vi "H2O_DIAL_NCAR_4CH_v4.09.vi"() -> ()   [LabVIEW 2012]
uses:
  C:/Users/H2ODial/Desktop/Shared Telescope WV DIAL Code/Libraries and VIs/PowerMeterCommands.dll
  Shared Telescope WV DIAL Code/Libraries and VIs/PowerMeterCommands.dll
  <vilib>/DAQmx/write.llb/DAQmx Write (Digital 1D Bool NChan 1Samp 1Line).vi
  <vilib>/DAQmx/miscellaneous.llb/DAQmx Fill In Error Info.vi
  <vilib>/Analysis/baseanly.llb/Mean (DBL).vi
  AMCS_Data.vi
  Libraries and VIs/Scalar_Data.vi
  <vilib>/Analysis/NI_AALBase.lvlib
  Libraries and VIs/Scalar_Data_2.vi
  Libraries and VIs/Scalar_Data_4.vi
  Libraries and VIs/Scalar_Data_3.vi
  Shared Telescope WV DIAL Code/bristol/CLDevIFace.dll
panel:
  out "FileHour":i32=18
  out "L_Count":i32=271
  out "sigma_off_total":dbl[](array[numeric])=[5.540716545669956e-25, 5.509038515319884e-25, 5.47745233176751e-25, 5.445958679910823e-25, 5.414558240969882e-25, 5.383251691981853e-25, 5.352039705244152e-25, 5.320922947769417e-25, 5.289902080890823e-25, 5.258977759647611e-25, 5.228150632368401e-25, 5.197421340189991e-25, 5.166790516619597e-25, 5.1362587870950455e-25, 5.1058267685284e-25, 5.075495068909035e-25, 5.045264286935022e-25, 5.015135011569438e-25, 4.9851078217155e-25, 4.955183285861175e-25, 4.925361961723897e-25, 4.895644395896113e-25, 4.866031123592904e-25, 4.83652266834119e-25, 4.807119541641849e-25, 4.77782224277593e-25, 4.7486312585251305e-25, 4.719547062922376e-25, 4.690570117073194e-25, 4.661700868866856e-25, 4.632939752896641e-25, 4.604287190200865e-25, 4.575743588116101e-25, 4.547309340157799e-25, 4.518984825887645e-25, 4.490770410729631e-25, 4.462666445972589e-25, 4.434673268575131e-25, 4.40679120118145e-25, 4.379020551981193e-25, 4.351361614712452e-25, 4.3238146686004e-25, 4.296379978359628e-25, 4.26905779413425e-25, 4.241848351562388e-25, 4.214751871753208e-25, 4.187768561289679e-25, 4.160898612350621e-25, 4.134142202652132e-25, 4.1074994956030275e-25, 4.0809706402935364e-25, 4.054555771658063e-25, 4.0282550104859823e-25, 4.002068463591525e-25, 3.9759962238789642e-25, 3.9500383704632943e-25, 3.9241949688533782e-25, 3.89846607100192e-25, 3.8728517155268345e-25, 3.8473519278212167e-25, 3.8219667202352144e-25, 3.7966960922230447e-25, 3.7715400305383413e-25, 3.74649850940483e-25, 3.7215714907036218e-25, 3.6967589241566724e-25, 3.672060747564097e-25, 3.647476886940111e-25, 3.6230072567890353e-25, 3.598651760279724e-25, 3.5744102894632373e-25, 3.550282725512238e-25, 3.5262689389447565e-25, 3.502368789807654e-25, 3.47858212798661e-25, 3.454908793351493e-25, 3.4313486160611974e-25, 3.407901416757848e-25, 3.3845670068390906e-25, 3.36134518864904e-25, 3.3382357557846445e-25, 3.31523849327317e-25, 3.292353177855014e-25, 3.269579578225686e-25, 3.2469174552554615e-25, 3.224366562247346e-25, 3.201926645171508e-25, 3.179597442913807e-25, 3.157378687515629e-25, 3.135270104405692e-25, 3.113271412644526e-25, 3.091382325146825e-25, 3.069602548935796e-25, 3.0479317853615826e-25, 3.026369730325113e-25, 3.004916074531155e-25, 2.9835705036817056e-25, 2.9623326987117465e-25, 2.941202336026831e-25, 2.9201790876899676e-25, 2.899262621653904e-25, 2.8784526019663433e-25, 2.8577486889781736e-25, 2.8371505395538697e-25, 2.8166578072571985e-25, 2.7962701425816637e-25, 2.775987193103717e-25, 2.7558086037064965e-25, 2.735734016758066e-25, 2.71576307229708e-25, 2.6958954082151585e-25, 2.6761306604360893e-25, 2.6564684630829226e-25, 2.6369084486778265e-25, 2.61745024828016e-25, 2.598093491667028e-25, 2.578837807496939e-25, 2.559682823474498e-25, 2.54062816650001e-25, 2.521673462824945e-25, 2.502818338212059e-25, 2.484062418077259e-25, 2.4654053276440287e-25, 2.446846692077008e-25, 2.4283861366280177e-25, 2.410023286792255e-25, 2.391757768411529e-25, 2.3735892078424688e-25, 2.3555172320627342e-25, 2.337541468826103e-25, 2.3196615467596074e-25, 2.3018770955218097e-25, 2.2841877458964754e-25, 2.2665931299334314e-25, 2.2490928810607227e-25, 2.2316866341927193e-25, 2.2143740258515955e-25, 2.197154694282537e-25, 2.1800282795472234e-25, 2.1629944236413983e-25, 2.146052770592492e-25, 2.1292029665592434e-25, 2.112444659932193e-25, 2.0957775014166358e-25, 2.0792011441327743e-25, 2.0627152437013555e-25, 2.0463194583169568e-25, 2.0300134488359706e-25, 2.0137968788457824e-25, 1.9976694147385576e-25, 1.9816307257768824e-25, 1.9656804841491914e-25, 1.9498183650353885e-25, 1.934044046652418e-25, 1.9183572103011107e-25, 1.9027575404100786e-25, 1.8872447245712642e-25, 1.871818453566729e-25, 1.8564784213957954e-25, 1.841224325294735e-25, 1.8260558657484057e-25, 1.810972746495391e-25, 1.7959746745324166e-25, 1.7810613601054828e-25, 1.7662325167008742e-25, 1.751487861025293e-25, 1.7368271129853726e-25, 1.7222499956532122e-25, 1.7077562352346513e-25, 1.6933455610234437e-25, 1.6790177053565633e-25, 1.6647724035593172e-25, 1.6506093938856987e-25, 1.636528417453577e-25, 1.6225292181758646e-25, 1.608611542684316e-25, 1.5947751402502352e-25, 1.581019762699804e-25, 1.5673451643257683e-25, 1.5537511017940605e-25, 1.540237334047793e-25, 1.5268036222071082e-25, 1.5134497294663046e-25, 1.5001754209881617e-25, 1.4869804637954348e-25, 1.473864626661357e-25, 1.460827679996712e-25, 1.4478693957377917e-25, 1.4349895472319421e-25, 1.4221879091216375e-25, 1.4094642572317599e-25, 1.3968183684535146e-25, 1.3842500206296053e-25, 1.3717589924428774e-25, 1.3593450633030128e-25, 1.3470080132367275e-25, 1.3347476227802004e-25, 1.32256367287135e-25, 1.3104559447485225e-25, 1.2984242198512939e-25, 1.2864682797194944e-25, 1.2745879059051496e-25, 1.2627828798814573e-25, 1.2510529829571843e-25, 1.2393979961981194e-25, 1.2278177003500287e-25, 1.2163118757700842e-25, 1.204880302361001e-25, 1.193522759513445e-25, 1.1822390260474241e-25, 1.1710288801689803e-25, 1.1598920994272827e-25, 1.1488284606766496e-25, 1.1378377400487363e-25, 1.1269197129279468e-25, 1.1160741539351538e-25, 1.1053008369155443e-25, 1.094599534933665e-25, 1.0839700202769103e-25, 1.0734120644581644e-25, 1.0629254382333933e-25, 1.0525099116192388e-25, 1.0421652539159365e-25, 1.0318912337377015e-25, 1.0216876190431015e-25, 1.0115541771807728e-25, 1.0014906749271105e-25, 9.914968785310339e-26, 9.815725537656191e-26, 9.717174659823899e-26, 9.619313801588218e-26, 9.522140609573087e-26, 9.425652727838355e-26, 9.329847798391668e-26, 9.234723461772877e-26, 9.140277357589357e-26, 9.046507125086315e-26, 8.953410403602918e-26, 8.860984833089776e-26, 8.769228054525757e-26, 8.678137710332858e-26, 8.587711444744364e-26, 8.497946904095774e-26, 8.408841737046818e-26, 8.320393594822389e-26, 8.232600131299494e-26, 8.145459003094604e-26, 8.058967869545014e-26, 7.973124392609961e-26, 7.887926236794523e-26, 7.80337106887695e-26, 7.719456557686526e-26, 7.636180373727653e-26, 7.553540188807418e-26, 7.47153367556762e-26, 7.390158506951166e-26, 7.309412355721905e-26, 7.22929289380143e-26, 7.149797791632498e-26, 7.070924717536157e-26, 6.992671337018222e-26, 6.915035312057113e-26, 6.838014300354704e-26, 6.761605954618939e-26, 6.685807921858866e-26, 6.61061784263726e-26, 6.536033350360778e-26, 6.462052070600663e-26, 6.388671620424742e-26, 6.315889607734174e-26, 6.243703630693181e-26, 6.172111277147462e-26, 6.101110124059749e-26, 6.030697737083214e-26, 5.960871670108947e-26, 5.891629464803492e-26, 5.822968650369955e-26]
  out "sigma_on_total":dbl[](array[numeric])=[3.7287541155959287e-23, 3.7294473381390915e-23, 3.729895983299971e-23, 3.7300992376506543e-23, 3.730056364270663e-23, 3.729766703617701e-23, 3.729229674071814e-23, 3.728444772415678e-23, 3.7274115748913616e-23, 3.7261297371484216e-23, 3.724598994972533e-23, 3.722819164604523e-23, 3.720790143143009e-23, 3.718511908815845e-23, 3.7159845210402426e-23, 3.71320812064078e-23, 3.710182930085371e-23, 3.7069092532052533e-23, 3.7033874753800484e-23, 3.69961806343696e-23, 3.6956015654087493e-23, 3.691338610146597e-23, 3.686829907341892e-23, 3.682076247098229e-23, 3.677078499195744e-23, 3.6718376130128133e-23, 3.666354616830143e-23, 3.6606306171503594e-23, 3.65466679828621e-23, 3.648464421148751e-23, 3.642024823133154e-23, 3.635349416790373e-23, 3.628439689018491e-23, 3.6212972002870696e-23, 3.613923583641449e-23, 3.6063205432233156e-23, 3.5984898538517206e-23, 3.590433359182844e-23, 3.582152971111225e-23, 3.573650667999674e-23, 3.5649284937303634e-23, 3.5559885561897056e-23, 3.546833026061457e-23, 3.537464135047522e-23, 3.5278841748472396e-23, 3.518095495390081e-23, 3.5081005031164986e-23, 3.49790166003625e-23, 3.4875014813139384e-23, 3.476902534357424e-23, 3.4661074365208697e-23, 3.455118854053173e-23, 3.443939499746446e-23, 3.432572131749493e-23, 3.421019551446019e-23, 3.409284601679323e-23, 3.3973701654248835e-23, 3.385279163246072e-23, 3.3730145521256737e-23, 3.360579323268562e-23, 3.3479765004528353e-23, 3.3352091380022967e-23, 3.322280319128026e-23, 3.3091931539878165e-23, 3.2959507778385764e-23, 3.2825563490963637e-23, 3.269013047870121e-23, 3.255324073466697e-23, 3.2414926432195465e-23, 3.227521990292009e-23, 3.2134153618673575e-23, 3.1991760175402e-23, 3.18480722753372e-23, 3.1703122704608974e-23, 3.155694432423841e-23, 3.1409570043398513e-23, 3.126103280985793e-23, 3.1111365588382064e-23, 3.096060134785198e-23, 3.0808773039207797e-23, 3.065591358683448e-23, 3.050205586515653e-23, 3.0347232687749715e-23, 3.0191476792033654e-23, 3.003482082145855e-23, 2.987729731269763e-23, 2.971893868034824e-23, 2.9559777203834095e-23, 2.939984501370705e-23, 2.923917407736587e-23, 2.907779618698884e-23, 2.891574294504204e-23, 2.875304575478364e-23, 2.8589735806501847e-23, 2.842584406506734e-23, 2.826140126245158e-23, 2.809643788235476e-23, 2.7930984151658057e-23, 2.7765070033138635e-23, 2.759872521128409e-23, 2.743197908578835e-23, 2.726486076178917e-23, 2.7097399041404717e-23, 2.6929622416549404e-23, 2.67615590585557e-23, 2.6593236816217257e-23, 2.6424683201727417e-23, 2.62559253894762e-23, 2.6086990208089785e-23, 2.5917904134629101e-23, 2.5748693289157014e-23, 2.5579383429670766e-23, 2.5409999945669205e-23, 2.524056785899295e-23, 2.507111181376249e-23, 2.4901656075333742e-23, 2.4732224526983488e-23, 2.4562840667772406e-23, 2.4393527608193136e-23, 2.422430806785886e-23, 2.405520437517099e-23, 2.3886238463936548e-23, 2.3717431873629354e-23, 2.3548805745800924e-23, 2.3380380824113516e-23, 2.3212177457869647e-23, 2.304421559359465e-23, 2.287651478317675e-23, 2.2709094177653898e-23, 2.2541972534144295e-23, 2.2375168208619667e-23, 2.2208699165636514e-23, 2.2042582971637662e-23, 2.1876836801909522e-23, 2.1711477440630507e-23, 2.1546521280412932e-23, 2.1381984326685983e-23, 2.121788220142687e-23, 2.1054230141008472e-23, 2.089104300259618e-23, 2.072833526537848e-23, 2.0566121033484556e-23, 2.0404414040514995e-23, 2.02432276490701e-23, 2.0082574857776725e-23, 1.992246830471324e-23, 1.9762920267394525e-23, 1.960394267008934e-23, 1.94455470854802e-23, 1.9287744739998634e-23, 1.913054651781045e-23, 1.897396296213913e-23, 1.8818004283613368e-23, 1.866268036173684e-23, 1.850800074923581e-23, 1.8353974677805328e-23, 1.8200611062528066e-23, 1.8047918504372124e-23, 1.789590529608809e-23, 1.7744579427440173e-23, 1.7593948589158073e-23, 1.7444020176312072e-23, 1.7294801295571033e-23, 1.714629876734015e-23, 1.6998519132395303e-23, 1.6851468654733394e-23, 1.6705153329424692e-23, 1.6559578883024505e-23, 1.6414750782637343e-23, 1.627067423639568e-23, 1.6127354201852297e-23, 1.5984795389478323e-23, 1.5843002266790507e-23, 1.570197906249157e-23, 1.556172977348953e-23, 1.5422258167225992e-23, 1.5283567787481222e-23, 1.514566195785594e-23, 1.5008543789162912e-23, 1.487221618004476e-23, 1.4736681823753744e-23, 1.460194321315896e-23, 1.4468002643544782e-23, 1.433486221757719e-23, 1.4202523850725678e-23, 1.4070989273456306e-23, 1.3940260038142742e-23, 1.381033752066934e-23, 1.3681222925678252e-23, 1.3552917292213956e-23, 1.342542149475035e-23, 1.329873624926878e-23, 1.3172862117706144e-23, 1.3047799509899543e-23, 1.2923548688946826e-23, 1.28001097745283e-23, 1.2677482746200306e-23, 1.2555667448526746e-23, 1.2434663593300286e-23, 1.2314470762702532e-23, 1.2195088415608677e-23, 1.2076515887836906e-23, 1.1958752396973187e-23, 1.1841797046178551e-23, 1.1725648826604141e-23, 1.1610306621528463e-23, 1.1495769208674356e-23, 1.1382035263790303e-23, 1.1269103362890336e-23, 1.115697198739454e-23, 1.1045639524974975e-23, 1.093510427291206e-23, 1.0825364441772833e-23, 1.0716418157387284e-23, 1.0608263464003192e-23, 1.05008983265787e-23, 1.0394320633818336e-23, 1.0288528200747024e-23, 1.0183518770471538e-23, 1.0079290018187703e-23, 9.975839552068408e-24, 9.873164916030698e-24, 9.771263592427396e-24, 9.670133003943853e-24, 9.569770516892366e-24, 9.47017344121427e-24, 9.371339034057028e-24, 9.273264502176353e-24, 9.175947003243377e-24, 9.079383647147766e-24, 8.983571499638456e-24, 8.888507583162242e-24, 8.794188878048888e-24, 8.700612325636301e-24, 8.607774829344434e-24, 8.515673256698243e-24, 8.424304440033053e-24, 8.333665179389652e-24, 8.243752243138888e-24, 8.154562370142944e-24, 8.066092270936068e-24, 7.978338628885573e-24, 7.891298101920694e-24, 7.80496732449342e-24, 7.719342907741134e-24, 7.634421441676455e-24, 7.550199495880042e-24, 7.466673621028348e-24, 7.383840350642027e-24, 7.30169620086398e-24, 7.220237672979087e-24, 7.139461253422007e-24, 7.05936341566137e-24, 6.979940620701889e-24, 6.901189318360428e-24, 6.823105948747092e-24, 6.745686941679033e-24, 6.668928718892326e-24, 6.59282769491507e-24, 6.5173802774298634e-24, 6.442582868121181e-24, 6.3684318634960925e-24, 6.2949236561454545e-24, 6.22205463525479e-24, 6.149821186879232e-24, 6.078219695127621e-24, 6.007246542845252e-24, 5.936898112053741e-24, 5.867170784601514e-24, 5.798060943221433e-24, 5.729564971475294e-24, 5.661679254562057e-24, 5.5944001805038156e-24, 5.527724139630574e-24, 5.461647525332996e-24, 5.396166735778275e-24, 5.331278172562546e-24]
  out "background start":u32=269
  in  "Tab Control 2":enum32{"WV ND narrow", "WV ND wide"}(tab)
  out "Water Vapor Number Density":dbl[][](graph)=[[1.5907904720888795, 1.2034317017988099, 0.9296649854345478, 1.1616212259902245, 1.143482414199353, 1.0161811220951331, 0.8436353618874357, 0.7348131682216585, 0.9164975212685635, 0.89811228919073, 0.7564201784133333, 0.837060094458364, 0.8546078060158476, 0.7580143042655286, 0.6660142729911659, 0.6130668071131011, 0.6226907103035824, 0.6044805130262904, 0.5136178398800642, 0.587738349780248, 0.7635774576583904, 0.7303067839902722, 0.4730691906410508, 0.3471652620966176, 0.41542162880598704, 0.5685575754839206, 0.7718433146264597, 0.7768105364827741, 0.6405925914018273, 0.4205887096400592, 0.40995294682639616, 0.7155794757740925, 0.920696843571624, 0.7649553709487822, 0.5302468241911644, 0.37096623546502394, 0.25769406190441974, -0.0080589765834906, -0.40357224901269145, -0.1794034230022969, 0.06823996411751274, -0.1224198075171402, 0.022920705948691274, 0.18133520539603096, 0.2313748454435181, 0.0652983697869732, -0.08869448307680232, -0.06007364897889734, -0.11102303519223886, -0.38389030387136974, -0.05447089846963266, 0.41844177760203766, 0.15079134457634047, -0.02984752116025162, 0.2182655699308987, 0.15944961231343657, 0.06694794530398825, -0.05077164509929912, 0.06906989476289672, 0.9067190268404879, 1.1453363881332252, 0.03472136913021536, 0.264565708581504, 0.43254477196191593, -0.47233628799813854, -0.29156055249168833, 0.1180678634792738, -0.09550337931524557, -0.10840044132528848, -0.6189329864228708, -1.0240098553620418, -0.6312727028738709, -0.9049119791449917, 0.22972264353619823, 0.8701075357624027, -0.03976535090548336, 0.23740439151064743, 0.6623974919824076, 0.5592431387574105, 0.3109308799725782, 0.3052939198256978, 0.6723826982889436, 0.8009120776096694, -0.4441313017280432, -0.3880356203973259, 0.5908496254246882, 0.1180230114318088, -0.01970262960437462, -0.31072879343114695, 0.27355192712564147, 0.6844411802637508, -0.32638781722295945, -0.2121915813145855, -0.34767820762694274, -0.8163608698872435, -0.9184353604486615, 0.3869192876522108, 0.40060562557133866, -0.095288682053356, -0.313027214072189, 0.3330781553600768, 0.8460255883855125, 0.601755995217996, 0.7754619300108345, 0.9765559065251931, 1.2271405584166755, -0.1658917325023355, -0.6358745698746214, 0.5914143596226265, 0.3637480127737773, -3.804191129911014, 1.7349758337131993, 3.649406363513137, 3.170084841477165, 2.7107594981208476, 4.46218946669049, -0.8382710343005657, -3.926831136573211, -4.486781021243031, -2.588326606030171, 1.9223034296942394, -2.3247951492620063, -6.536774240649516, -1.7562773314567135, -5.600536422111381, -7.337941687196924, -2.5387360902995404, 1.105817947103975, 6.324135594448845, 3.5648446608266893, -2.486757603992552, -2.422866895285222, -0.38960203240978497, -9.035086985848327, -1.5683938012810983, 10.011163431560586, 9.216674690323467, 5.255808387763412, -3.465437027624479, -4.196720002137542, 1.1705350848689553, -2.1809542243340996, 0.6006947251125062, 4.770499709190255, -2.6554725073402805, -15.030268047279796, -6.802745114341266, 0.11993457124003391, -4.6755558693463195, -2.366147968637075, -2.878254308609073, -0.6714780835778198, 3.5925789031525404, 13.368751255421428, 12.455719203731226, -0.05985744528603264, 2.7510736142942425, -5.73541466983283, 1.1185576943051152, 6.217299010474867, 3.5118216444138146, 4.524381746749669, -2.366889618966624, -5.853801494466987, -9.859632826133716, 5.264317843451557, -13.239841159796926, -5.835489303175296, -6.856046068640341, -2.931243755146569, 1.7279250440517042, -2.5519203638730312, -8.40861731587334, -10.899346396172595, -0.5346687063856269, -5.331897062505065, 7.557385703757733, 11.7065020006105, 2.946693090049258, -13.090521829508926, 0.12945987300255424, 2.202161925374446, -3.3974959113211276, -2.1035236517762215, -6.873354435596117, 4.147469539646433, -9.299678021367697, -19.337116943953266, -6.52923929570179, 9.028137640587774, -2.5392877408600474, 8.684390946594228, 10.72485032797892, 2.6585182442080395, 3.293002306885864, -4.886636914469689, 9.766253413272993, 12.193301254863965, 7.719788066440548, -4.754884429943826, -17.13597095272275, -12.751353082806622, -5.375215583749998, -6.476632305845586, -2.208373363948193, -15.699582657418768, -5.677063755349945, 12.830240222974858, -2.363703015187705, 5.711208752282037, 15.96797510796814, 10.384366912962465, 12.793559331104248, 4.892315968247829, 15.262636300291334, 26.82949168143399, -25.386500576518493, -28.825339119768802, 6.6240516935873295, -12.1943057084576, -15.705603079063485, -17.239016867432447, -24.131046157506326, -7.692424625838223, -21.695120224534115, 9.216178268982365, 14.146901600795102, 7.514076113222446, -15.034259757068584, 8.507536833359039, 8.923486850615697, 18.85572266218953, 8.12380444446765, 1.259268077023489, -15.627451138756522, -41.18212544212433, 12.547106790703646, 9.808576087000565, 6.905576895548879, -43.22640447137988, -8.598442304470684, -21.432640937029724, -36.852744144658345, -7.986086979764478, 8.247535761925763, 14.354499632201671, -7.321765339253622, -8.957884617681414, 4.555596819004534, 39.990037008305876, 14.57933556870722, -34.65987801636803, 27.309780862368687, 10.28770562322102, -0.551570352035954, 3.7735022403998273, 16.910498698261218, 45.99805730845316, 2.6131709059900223, 0.9278756920238553, -11.315937931604367, 49.57606981212727, 50.40635075338968, -12.147992445798641, 11.54303622375683, -6.904533648249454, -9.4388422387742, -44.10612578209894, -7.55259670107014, 3.2842370521836184, -4.114095565580007, -19.832024130620947, -49.705810949430884, 3.5348659680191195, -6.116300118169566, -1.594820427102057, 0.0, 0.0, 0.0, 0.0]]
  out "Water Vapor Number Density 2":dbl[][](graph)=[[nan, nan, nan, nan, nan, nan, nan, nan, nan, nan, nan, nan, nan, nan, nan, nan, nan, nan, nan, nan, nan, nan, nan, nan, nan, nan, nan, nan, nan, nan, nan, nan, nan, nan, nan, nan, nan, nan, nan, nan, nan, nan, nan, nan, nan, nan, nan, nan, nan, nan, nan, nan, nan, nan, nan, nan, nan, nan, nan, nan, nan, nan, nan, nan, nan, nan, nan, nan, nan, nan, nan, nan, nan, nan, nan, nan, nan, nan, nan, nan, nan, nan, nan, nan, nan, nan, nan, nan, nan, nan, nan, nan, nan, nan, nan, nan, nan, nan, nan, nan, nan, nan, nan, nan, nan, nan, nan, nan, nan, nan, nan, nan, nan, nan, nan, nan, nan, nan, nan, nan, nan, nan, nan, nan, nan, nan, nan, nan, nan, nan, nan, nan, nan, nan, nan, nan, nan, nan, nan, nan, nan, nan, nan, nan, nan, nan, nan, nan, nan, nan, nan, nan, nan, nan, nan, nan, nan, nan, nan, nan, nan, nan, nan, nan, nan, nan, nan, nan, nan, nan, nan, nan, nan, nan, nan, nan, nan, nan, nan, nan, nan, nan, nan, nan, nan, nan, nan, nan, nan, nan, nan, nan, nan, nan, nan, nan, nan, nan, nan, nan, nan, nan, nan, nan, nan, nan, nan, nan, nan, nan, nan, nan, nan, nan, nan, nan, nan, nan, nan, nan, nan, nan, nan, nan, nan, nan, nan, nan, nan, nan, nan, nan, nan, nan, nan, nan, nan, nan, nan, nan, nan, nan, nan, nan, nan, nan, nan, nan, nan, nan, nan, nan, nan, nan, nan, nan, nan, nan, nan, nan, nan, nan, nan, nan, nan, nan, nan, nan, nan, nan, nan, nan, nan, nan, nan, nan, 0.0, 0.0, 0.0, 0.0]] caption="Water Vapor Number Density"
  out "RingBuffer offline near":dbl[][](array[numeric])
  out "RingBuffer aerosol near":dbl[][](array[numeric])
  in  "?":T1(tab)
  out "NRB":dbl[][](graph)=[[1.234433300946586e-05, 5.1443483535392135e-05, 0.0001360213302022216, 0.00029113411007152754, 0.0005291807150624411, 0.0008826085456535516, 0.0014179373109353436, 0.0022510743244282417, 0.0034346663092669366, 0.00468268704743922, 0.005843069772728496, 0.007044930989790705, 0.008465338155639778, 0.009887181304892077, 0.011144357796541531, 0.012460718085578401, 0.013638073480806067, 0.015173484188794429, 0.017034621925368268, 0.019105492601255148, 0.021009384725544634, 0.022470108325935656, 0.024130710960447638, 0.025765965264351678, 0.027159417434196115, 0.028604277736811165, 0.030119284330183314, 0.03157610749073622, 0.03294928394697462, 0.034075064898022686, 0.035216817414831625, 0.03642083222121654, 0.03753856548137726, 0.03859373028073722, 0.039101350263739086, 0.03960016791827977, 0.03981519724115361, 0.03863242188934803, 0.036395371073058215, 0.032576523686743235, 0.028702944157995663, 0.02564600175172518, 0.02362705484468087, 0.02280774719217402, 0.02216446437445086, 0.021413362357354467, 0.020877565084704834, 0.021659799562053533, 0.021487289922586413, 0.020956875606443524, 0.020915183915428803, 0.020347241033551313, 0.02060540082840942, 0.020894728731721424, 0.022140905736160944, 0.02184175911887354, 0.019642024957991524, 0.020179379702574357, 0.020227721433660584, 0.019183059778169514, 0.019538781169616343, 0.020159764890089398, 0.021335593065996264, 0.021176459855630513, 0.02025716830842799, 0.019644638108401676, 0.01895143905507171, 0.020718574913986026, 0.020739199761896174, 0.018410987106026507, 0.018638968117081673, 0.019796828627004198, 0.02030744459723528, 0.0195473749072039, 0.018213419551479874, 0.01654349442693267, 0.01652124608667888, 0.01724847147270722, 0.018582194958477478, 0.02042251544846188, 0.018813105830755603, 0.017169913884120043, 0.01626486889125005, 0.017549617362589077, 0.01829726425647039, 0.022918652005612054, 0.1154604309066741, 0.4441988571570757, 0.868165199511663, 1.0249560287953854, 0.8733755618521651, 0.5904076748185508, 0.2799568095326156, 0.07974835673518459, 0.02624347617856174, 0.01789704422404187, 0.01615591486633874, 0.012684032852312382, 0.013166196384633485, 0.012980539485474155, 0.015650930530186635, 0.03383904814031927, 0.07012968637531532, 0.08809419238107312, 0.05931906216833834, 0.02792789508630294, 0.019158624376438255, 0.02019774408185465, 0.03506737203278766, 0.07520747328840331, 0.14844367179765303, 0.19752717680716583, 0.17433158925257825, 0.10942606582589529, 0.04590320608974301, 0.014810807017588898, 0.0095087897288594, 0.009739603190666676, 0.007774898812201258, 0.007882823515984447, 0.008867404826696852, 0.007762528503511155, 0.007792408016191122, 0.008939453762149085, 0.0046355793197030825, 0.004093675381731552, 0.0112819635063389, 0.007299129778193877, 0.002998798427775306, 0.008403857221283667, 0.007700808323427195, 0.003619061977076943, -0.0007325244276094363, 0.004397635643609695, 0.007028456680075337, 0.00716288823689265, 0.013401866147882677, 0.010702301794589367, 0.004731940202171024, 0.0004248550800729844, 0.005705271730534755, 0.006569333553426059, 0.0007740484680471754, 0.0046424206139200645, 0.006679785361861954, 0.006530862074299372, 0.007040107555841286, 0.001998405760258702, -0.0014939782963201535, 0.0017616060616320367, 0.007317801716963137, 0.007116049712545383, 0.007172121894223776, 0.0069592642647561325, 0.00417397871278734, 0.00950326259717531, 0.009465992936290947, 0.004700563845798458, -0.000597071407086473, -0.0013914188590054815, 0.005970975152700096, 0.00846525969960583, 0.005991304905256514, 0.005847500472455955, 0.009618473488323316, 0.005188621107788106, -0.001921856401090672, 0.0010683526804324646, 0.006163288706577327, -0.001804528109304894, 0.0026204935547409157, 0.009255466222221528, 0.004715561768675386, -0.00380047290439554, -0.004290137015315642, 0.007686604269562794, 0.014210582847400515, 0.02113730772503547, 0.005359312013519044, -0.0013417260135986074, 0.008500520818808645, 0.008648292220440447, 0.009122807482367197, 0.01880723852216641, 0.02222345248041923, 0.010263840137244662, 0.0017762058907801136, -0.004665338597325305, -0.0087598804790557, 0.0003153411780736893, 0.005393802481392054, 0.0025880518002595714, 0.00014461238894867371, 0.002520487356106442, 0.008267073373926888, -0.002647281562777412, -0.008449934734266263, 0.006176914817706903, 0.015464279343800926, -0.0018505669675625345, -0.007946975837463982, 0.0010164908204106052, -0.0059061288231068146, -0.0095996518081358, -0.011325507559330376, -0.015623558657425672, -0.004200405409994922, 0.005066952322658379, 0.006246357871514664, -0.004608386446194331, -0.0035000915705954106, 0.00744481811619893, 0.0065611320535040075, 0.002622475046995397, -0.0034097306422209, -0.006988685479635922, -0.014518329666749605, -0.007964333628519648, 0.005694635078767304, 0.0010491319324251254, -0.0031286588465574898, 0.0032208315257082278, -0.00921872246730583, -0.019771796907954692, 0.00486443833633705, 0.018292800913009243, 0.0003667617929685996, -0.008879944646630627, -0.0007295394001955482, -0.012116985094404025, -0.009719385382020803, 0.00734852761980512, -5.269175333552519e-05, 0.00393274230797513, 0.004859769900681597, 0.0012973778279251357, 0.002489588612626492, 0.013597889384939226, -0.0016262509228943656, -0.021672315728432614, -0.014149283740657563, -0.012277550085026154, -0.0023497764480885732, 0.013906902950541, 0.006447356183760933, 0.003171726253791945, -0.009138646957028207, -0.005531669009374023, 0.018795463977986007, 4.044078657698842e-05, -0.0007745338429362863, 0.006923766628336878, 0.008117809454301834, 0.017157475167751162, 0.021605586968950964, 0.001314563392099188, -0.0014530626921270076, 0.00305800445458022, -0.003754518442223117, -0.009360470125742724, -0.02012131218995404, -0.024828344148993344, -0.00946583845920866, 0.025412511568150713, 0.0068613557202605955, -0.035206321462813654, -0.007449597763327604, 0.009341302591007442, 0.018307338829631026, 0.004174566139531062, -0.023831068930836932, -0.00868864373808385, -0.014298361371619944, -0.0060236676379142404, -0.0021530650031317093, -0.003893892385808913, 0.007993312007819367, 0.0, 0.0, 0.0]] caption="Water Vapor Number Density"
  out "NRB 2":dbl[][](graph) caption="Water Vapor Number Density"
  out "raw counts":dbl[][](graph)=[[72.4, 66.4, 81.4, 72.4, 99.4, 123.4, 159.4, 183.4, 203.4, 231.4, 254.4, 244.4, 254.4, 279.4, 257.4, 291.4, 229.4, 245.4, 252.4, 253.4, 244.4, 209.4, 256.4, 235.4, 255.4, 225.4, 214.4, 190.4, 210.4, 203.4, 193.4, 193.4, 171.4, 183.4, 175.4, 159.4, 151.4, 147.4, 143.4, 111.4, 95.4, 101.4, 67.4, 90.4, 62.400000000000006, 39.400000000000006, 68.4, 56.400000000000006, 49.400000000000006, 29.400000000000006, 48.400000000000006, 53.400000000000006, 58.400000000000006, 46.400000000000006, 39.400000000000006, 54.400000000000006, 41.400000000000006, 47.400000000000006, 42.400000000000006, 23.400000000000006, 34.400000000000006, 13.400000000000006, 38.400000000000006, 16.400000000000006, 45.400000000000006, 33.400000000000006, 12.400000000000006, 16.400000000000006, 30.400000000000006, 19.400000000000006, 15.400000000000006, 17.400000000000006, 28.400000000000006, 35.400000000000006, 16.400000000000006, 13.400000000000006, 1.4000000000000057, 24.400000000000006, 18.400000000000006, 32.400000000000006, 35.400000000000006, 33.400000000000006, 18.400000000000006, 10.400000000000006, 15.400000000000006, 23.400000000000006, 47.400000000000006, 237.4, 414.4, 401.4, 308.4, 325.4, 162.4, 40.400000000000006, 10.400000000000006, 12.400000000000006, 9.400000000000006, 3.4000000000000057, 12.400000000000006, -3.5999999999999943, -1.5999999999999943, 27.400000000000006, -11.599999999999994, 28.400000000000006, 13.400000000000006, 19.400000000000006, 27.400000000000006, 15.400000000000006, 16.400000000000006, 30.400000000000006, 89.4, 78.4, 101.4, 100.4, 57.400000000000006, 17.400000000000006, 9.400000000000006, 1.4000000000000057, 18.400000000000006, -7.599999999999994, 16.400000000000006, -2.5999999999999943, 17.400000000000006, 7.400000000000006, 10.400000000000006, 9.400000000000006, -7.599999999999994, 22.400000000000006, 2.4000000000000057, 8.400000000000006, 11.400000000000006, -6.599999999999994, 15.400000000000006, -0.5999999999999943, -2.5999999999999943, 8.400000000000006, 8.400000000000006, 5.400000000000006, 18.400000000000006, 1.4000000000000057, -8.599999999999994, 4.400000000000006, -6.599999999999994, 13.400000000000006, -0.5999999999999943, -0.5999999999999943, 13.400000000000006, 25.400000000000006, -8.599999999999994, -10.599999999999994, -6.599999999999994, -5.599999999999994, -1.5999999999999943, -2.5999999999999943, -0.5999999999999943, 19.400000000000006, 11.400000000000006, 15.400000000000006, 4.400000000000006, -9.599999999999994, -5.599999999999994, 0.4000000000000057, -1.5999999999999943, 14.400000000000006, 13.400000000000006, 6.400000000000006, 5.400000000000006, -11.599999999999994, 14.400000000000006, -21.599999999999994, 3.4000000000000057, 6.400000000000006, 10.400000000000006, 7.400000000000006, -2.5999999999999943, -1.5999999999999943, -0.5999999999999943, 2.4000000000000057, 4.400000000000006, -5.599999999999994, -2.5999999999999943, -4.599999999999994, 21.400000000000006, -3.5999999999999943, 10.400000000000006, 5.400000000000006, 1.4000000000000057, 2.4000000000000057, 0.4000000000000057, -1.5999999999999943, -2.5999999999999943, 1.4000000000000057, 3.4000000000000057, 12.400000000000006, 22.400000000000006, 7.400000000000006, -11.599999999999994, 25.400000000000006, 5.400000000000006, -2.5999999999999943, 0.4000000000000057, 3.4000000000000057, 0.4000000000000057, 4.400000000000006, 8.400000000000006, 23.400000000000006, -21.599999999999994, 0.4000000000000057, -6.599999999999994, 3.4000000000000057, 2.4000000000000057, 17.400000000000006, 7.400000000000006, 0.4000000000000057, 7.400000000000006, 6.400000000000006, -2.5999999999999943, -6.599999999999994, 8.400000000000006, -14.599999999999994, 3.4000000000000057, 23.400000000000006, -6.599999999999994, 1.4000000000000057, -3.5999999999999943, 16.400000000000006, -1.5999999999999943, 15.400000000000006, 1.4000000000000057, 5.400000000000006, -6.599999999999994, 18.400000000000006, 11.400000000000006, 1.4000000000000057, 2.4000000000000057, 10.400000000000006, -0.5999999999999943, 2.4000000000000057, 8.400000000000006, -9.599999999999994, 17.400000000000006, -0.5999999999999943, 19.400000000000006, -0.5999999999999943, 11.400000000000006, 6.400000000000006, 2.4000000000000057, 16.400000000000006, 15.400000000000006, 13.400000000000006, 19.400000000000006, 15.400000000000006, 0.4000000000000057, 3.4000000000000057, 0.4000000000000057, 1.4000000000000057, 14.400000000000006, -7.599999999999994, 1.4000000000000057, 4.400000000000006, -0.5999999999999943, -6.599999999999994, -1.5999999999999943, 13.400000000000006, -2.5999999999999943, -7.599999999999994, -17.599999999999994, -17.599999999999994, 8.400000000000006, 19.400000000000006, 3.4000000000000057, 5.400000000000006, 6.400000000000006, -9.599999999999994, 1.4000000000000057, -9.599999999999994, 1.4000000000000057, -16.599999999999994, -1.5999999999999943, 0.0]] caption="Water Vapor Number Density"
  out "raw counts near":dbl[][](graph) caption="Water Vapor Number Density"
  out "Aerosol Smoothed 2":dbl[](array[numeric])
  out "Off-Line Smoothed 2":dbl[](array[numeric])
  out "Off-Line Bin Readings 2":dbl[](array[numeric])
  out "On-Line Smoothed 2":dbl[](array[numeric])
  out "On-Line Bin Readings 2":dbl[](array[numeric])
  in  "stop":bool
  in  "Reset Average":bool=TRUE
  in  "Save Data?":bool=TRUE
  in  "Collect Data?":bool=TRUE
  in  "ILX Address":i32=6 min=0 step=1
  in  "Lambda On DBR Current":dbl=171.13999999999868
  in  "Lambda Off DBR Current":dbl=172.9499999999997
  in  "Tab Control":T2(tab)=enum."NRB"
  out "Water Vapor Number Density  2":cluster{"Y":dbl[], "Y":dbl[]}[](graph)=[{"Y"=array[276 elements], "Y"=array[280 elements]}, {"Y"=[nan, nan, nan, nan, nan, nan, nan, nan, nan, nan, nan, nan, nan, nan, nan, nan, nan, nan, nan, nan, nan, nan, nan, nan, nan, nan, nan, nan, nan, nan, nan, nan, nan, nan, nan, nan, nan, nan, nan, nan, nan, nan, nan, nan, nan, nan, nan, nan, nan, nan, nan, nan, nan, nan, nan, nan, nan, nan, nan, nan, nan, nan, nan, nan, nan, nan, nan, nan, nan, nan, nan, nan, nan, nan, nan, nan, nan, nan, nan, nan, nan, nan, nan, nan, nan, nan, nan, nan, nan, nan, nan, nan, nan, nan, nan, nan, nan, nan, nan, nan, nan, nan, nan, nan, nan, nan, nan, nan, nan, nan, nan, nan, nan, nan, nan, nan, nan, nan, nan, nan, nan, nan, nan, nan, nan, nan, nan, nan, nan, nan, nan, nan, nan, nan, nan, nan, nan, nan, nan, nan, nan, nan, nan, nan, nan, nan, nan, nan, nan, nan, nan, nan, nan, nan, nan, nan, nan, nan, nan, nan, nan, nan, nan, nan, nan, nan, nan, nan, nan, nan, nan, nan, nan, nan, nan, nan, nan, nan, nan, nan, nan, nan, nan, nan, nan, nan, nan, nan, nan, nan, nan, nan, nan, nan, nan, nan, nan, nan, nan, nan, nan, nan, nan, nan, nan, nan, nan, nan, nan, nan, nan, nan, nan, nan, nan, nan, nan, nan, nan, nan, nan, nan, nan, nan, nan, nan, nan, nan, nan, nan, nan, nan, nan, nan, nan, nan, nan, nan, nan, nan, nan, nan, nan, nan, nan, nan, nan, nan, nan, nan, nan, nan, nan, nan, nan, nan, nan, nan, nan, nan, nan, nan, nan, nan, nan, nan, nan, nan, nan, nan, nan, nan, nan, nan, nan, nan], "Y"=array[280 elements]}]
  out "Absolute Humidity":cluster{"Y":dbl[], "Y":dbl[]}[](graph)=[{"Y"=array[276 elements], "Y"=array[280 elements]}, {"Y"=[nan, nan, nan, nan, nan, nan, nan, nan, nan, nan, nan, nan, nan, nan, nan, nan, nan, nan, nan, nan, nan, nan, nan, nan, nan, nan, nan, nan, nan, nan, nan, nan, nan, nan, nan, nan, nan, nan, nan, nan, nan, nan, nan, nan, nan, nan, nan, nan, nan, nan, nan, nan, nan, nan, nan, nan, nan, nan, nan, nan, nan, nan, nan, nan, nan, nan, nan, nan, nan, nan, nan, nan, nan, nan, nan, nan, nan, nan, nan, nan, nan, nan, nan, nan, nan, nan, nan, nan, nan, nan, nan, nan, nan, nan, nan, nan, nan, nan, nan, nan, nan, nan, nan, nan, nan, nan, nan, nan, nan, nan, nan, nan, nan, nan, nan, nan, nan, nan, nan, nan, nan, nan, nan, nan, nan, nan, nan, nan, nan, nan, nan, nan, nan, nan, nan, nan, nan, nan, nan, nan, nan, nan, nan, nan, nan, nan, nan, nan, nan, nan, nan, nan, nan, nan, nan, nan, nan, nan, nan, nan, nan, nan, nan, nan, nan, nan, nan, nan, nan, nan, nan, nan, nan, nan, nan, nan, nan, nan, nan, nan, nan, nan, nan, nan, nan, nan, nan, nan, nan, nan, nan, nan, nan, nan, nan, nan, nan, nan, nan, nan, nan, nan, nan, nan, nan, nan, nan, nan, nan, nan, nan, nan, nan, nan, nan, nan, nan, nan, nan, nan, nan, nan, nan, nan, nan, nan, nan, nan, nan, nan, nan, nan, nan, nan, nan, nan, nan, nan, nan, nan, nan, nan, nan, nan, nan, nan, nan, nan, nan, nan, nan, nan, nan, nan, nan, nan, nan, nan, nan, nan, nan, nan, nan, nan, nan, nan, nan, nan, nan, nan, nan, nan, nan, nan, nan, nan], "Y"=array[280 elements]}]
  out "NRB plot":cluster{"Y":dbl[], "Y":dbl[]}[](graph)
  in  "background length":i32=10
  out "Correction":cluster{"Y":dbl[], "Y":dbl[]}[](graph)=[{"Y"=array[277 elements], "Y"=array[280 elements]}, {"Y"=[1.0, 1.0, 1.0, 1.0, 1.0, 1.0, 1.0, 1.0, 1.0, 1.0, 1.0, 1.0, 1.0, 1.0, 1.0, 1.0, 1.0, 1.0, 1.0, 1.0, 1.0, 1.0, 1.0, 1.0, 1.0, 1.0, 1.0, 1.0, 1.0, 1.0, 1.0, 1.0, 1.0, 1.0, 1.0, 1.0, 1.0, 1.0, 1.0, 1.0, 1.0, 1.0, 1.0, 1.0, 1.0, 1.0, 1.0, 1.0, 1.0, 1.0, 1.0, 1.0, 1.0, 1.0, 1.0, 1.0, 1.0, 1.0, 1.0, 1.0, 1.0, 1.0, 1.0, 1.0, 1.0, 1.0, 1.0, 1.0, 1.0, 1.0, 1.0, 1.0, 1.0, 1.0, 1.0, 1.0, 1.0, 1.0, 1.0, 1.0, 1.0, 1.0, 1.0, 1.0, 1.0, 1.0, 1.0, 1.0, 1.0, 1.0, 1.0, 1.0, 1.0, 1.0, 1.0, 1.0, 1.0, 1.0, 1.0, 1.0, 1.0, 1.0, 1.0, 1.0, 1.0, 1.0, 1.0, 1.0, 1.0, 1.0, 1.0, 1.0, 1.0, 1.0, 1.0, 1.0, 1.0, 1.0, 1.0, 1.0, 1.0, 1.0, 1.0, 1.0, 1.0, 1.0, 1.0, 1.0, 1.0, 1.0, 1.0, 1.0, 1.0, 1.0, 1.0, 1.0, 1.0, 1.0, 1.0, 1.0, 1.0, 1.0, 1.0, 1.0, 1.0, 1.0, 1.0, 1.0, 1.0, 1.0, 1.0, 1.0, 1.0, 1.0, 1.0, 1.0, 1.0, 1.0, 1.0, 1.0, 1.0, 1.0, 1.0, 1.0, 1.0, 1.0, 1.0, 1.0, 1.0, 1.0, 1.0, 1.0, 1.0, 1.0, 1.0, 1.0, 1.0, 1.0, 1.0, 1.0, 1.0, 1.0, 1.0, 1.0, 1.0, 1.0, 1.0, 1.0, 1.0, 1.0, 1.0, 1.0, 1.0, 1.0, 1.0, 1.0, 1.0, 1.0, 1.0, 1.0, 1.0, 1.0, 1.0, 1.0, 1.0, 1.0, 1.0, 1.0, 1.0, 1.0, 1.0, 1.0, 1.0, 1.0, 1.0, 1.0, 1.0, 1.0, 1.0, 1.0, 1.0, 1.0, 1.0, 1.0, 1.0, 1.0, 1.0, 1.0, 1.0, 1.0, 1.0, 1.0, 1.0, 1.0, 1.0, 1.0, 1.0, 1.0, 1.0, 1.0, 1.0, 1.0, 1.0, 1.0, 1.0, 1.0, 1.0, 1.0, 1.0, 1.0, 1.0, 1.0, 1.0, 1.0, 1.0, 1.0, 1.0, 1.0, 1.0, 1.0, 1.0, 1.0, 1.0, 1.0, 1.0, 1.0, 1.0, 1.0, 1.0, 1.0, 1.0, 1.0, 1.0, 1.0, 1.0, 1.0, 1.0], "Y"=array[280 elements]}]
  in  "dead time":dbl=3.7e-08
  out "Optical Depth":cluster{"Y":dbl[], "Y":dbl[]}[](graph) caption="XY Graph"
  out "RingBuffer offline far":dbl[][](array[numeric])
  out "RingBuffer aerosol far":dbl[][](array[numeric])
  in  "Weather":T3(tab)=enum."Pulse Energy (Micro Joule)"
  out "Temperature (C)":dbl(graph)=13.42460317460317
  out "Pressure (mb)":dbl(graph)=833.7225274725275
  out "Relative Humdity (%)":dbl(graph)=37.02686202686203
  out "Pulse Energy (Micro Joule)":T4(graph)={"Online Pulse Energy"=4.293568571428572, "Pulse Energy Offline"=4.298335714285714}
  out "?":cluster{"mean":dbl, "mean":dbl}(graph)={"mean"=20920.0, "mean"=0.0}
  out "Index":i32=272
  out "Aerosol Smoothed":dbl[](array[numeric])=[65.75344827586204, 68.50344827586204, 80.49482758620687, 96.89999999999998, 112.7103448275862, 130.5293103448276, 154.03793103448277, 187.18448275862073, 225.59827586206904, 249.08965517241387, 256.8568965517242, 260.2189655172415, 266.41724137931044, 268.296551724138, 263.4431034482759, 258.9000000000001, 251.02068965517248, 249.1155172413794, 251.00344827586213, 254.06379310344835, 253.40862068965524, 246.96034482758628, 242.65862068965527, 237.9689655172415, 231.1844827586208, 225.12413793103457, 219.82241379310352, 214.296551724138, 208.46896551724143, 201.46896551724143, 195.01206896551727, 189.27931034482762, 183.45172413793108, 177.68448275862073, 169.89137931034486, 162.64137931034483, 154.8137931034483, 142.42586206896556, 127.4, 108.41724137931033, 90.93448275862067, 77.43448275862066, 68.06379310344823, 62.75344827586204, 58.30517241379307, 53.90862068965515, 50.34827586206896, 50.08103448275861, 47.67586206896551, 44.658620689655166, 42.839655172413785, 40.089655172413785, 39.081034482758625, 38.175862068965515, 38.994827586206895, 37.106896551724134, 32.210344827586205, 31.960344827586205, 30.960344827586205, 28.391379310344828, 27.977586206896554, 27.94310344827586, 28.641379310344824, 27.546551724137935, 25.54655172413793, 24.029310344827586, 22.494827586206895, 23.874137931034483, 23.210344827586205, 20.02068965517241, 19.701724137931034, 20.348275862068967, 20.305172413793102, 19.020689655172415, 17.25344827586207, 15.26206896551724, 14.848275862068963, 15.106896551724137, 15.865517241379308, 17.00344827586207, 15.279310344827586, 13.606896551724137, 12.58103448275862, 13.253448275862068, 13.494827586206895, 16.51206896551724, 81.2448275862069, 304.99482758620695, 581.5810344827586, 670.9948275862068, 559.7275862068966, 370.71896551724143, 172.2793103448276, 48.08103448275861, 15.494827586206895, 10.348275862068965, 9.149999999999999, 7.0379310344827575, 7.158620689655171, 6.917241379310344, 8.175862068965516, 17.331034482758618, 35.21896551724138, 43.39137931034483, 28.667241379310347, 13.244827586206899, 8.917241379310344, 9.22758620689655, 15.72758620689655, 33.115517241379294, 64.17586206896549, 83.86551724137928, 72.71896551724136, 44.856896551724134, 18.494827586206895, 5.865517241379309, 3.7017241379310333, 3.727586206896551, 2.925862068965517, 2.917241379310344, 3.227586206896551, 2.7793103448275853, 2.7448275862068963, 3.098275862068965, 1.58103448275862, 1.374137931034482, 3.727586206896551, 2.3741379310344817, 0.9603448275862058, 2.6499999999999986, 2.391379310344827, 1.1068965517241374, -0.22068965517241473, 1.3051724137931022, 2.0551724137931022, 2.0637931034482757, 3.8051724137931027, 2.9948275862068954, 1.3051724137931022, 0.11551724137930941, 1.5293103448275853, 1.7362068965517232, 0.20172413793103355, 1.1931034482758613, 1.6931034482758613, 1.6327586206896543, 1.7362068965517232, 0.4862068965517233, -0.35862068965517335, 0.41724137931034394, 1.7103448275862059, 1.6413793103448266, 1.6327586206896545, 1.5637931034482753, 0.9258620689655164, 2.08103448275862, 2.0465517241379305, 1.003448275862068, -0.1258620689655181, -0.289655172413794, 1.2275862068965508, 1.7189655172413785, 1.2017241379310335, 1.1586206896551716, 1.8827586206896543, 1.003448275862068, -0.36724137931034573, 0.2017241379310335, 1.149999999999999, -0.3327586206896561, 0.4775862068965512, 1.6672413793103442, 0.839655172413792, -0.6689655172413803, -0.7465517241379318, 1.3224137931034474, 2.4172413793103438, 3.5551724137931027, 0.8913793103448266, -0.220689655172415, 1.3827586206896543, 1.3913793103448269, 1.4517241379310337, 2.960344827586206, 3.460344827586206, 1.58103448275862, 0.27068965517241284, -0.7034482758620699, -1.3068965517241389, 0.04655172413793007, 0.7879310344827577, 0.37413793103448184, 0.02068965517241289, 0.3568965517241366, 1.1586206896551712, -0.36724137931034573, -1.1603448275862078, 0.8396551724137921, 2.0810344827586196, -0.2465517241379318, -1.0482758620689665, 0.13275862068965424, -0.7637931034482764, -1.2293103448275868, -1.4362068965517252, -1.9620689655172425, -0.5224137931034492, 0.6241379310344819, 0.7620689655172405, -0.5568965517241389, -0.4189655172413803, 0.8827586206896543, 0.770689655172413, 0.30517241379310256, -0.39310344827586297, -0.7982758620689664, -1.6431034482758629, -0.8931034482758629, 0.6327586206896544, 0.11551724137930952, -0.3413793103448285, 0.3482758620689646, -0.9879310344827592, -2.1000000000000005, 0.5120689655172405, 1.9086206896551714, 0.0379310344827577, -0.9103448275862078, -0.07413793103448368, -1.220689655172415, -0.9706896551724149, 0.7275862068965508, -0.0051724137931043745, 0.38275862068965427, 0.4689655172413784, 0.12413793103448183, 0.23620689655172322, 1.2793103448275853, -0.15172413793103545, -2.0051724137931046, -1.2982758620689667, -1.117241379310346, -0.2120689655172423, 1.2448275862068954, 0.572413793103447, 0.27931034482758527, -0.7982758620689666, -0.4793103448275877, 1.615517241379309, 0.003448275862067973, -0.06551724137931131, 0.5810344827586198, 0.6758620689655163, 1.4172413793103438, 1.7706896551724127, 0.10689655172413692, -0.11724137931034584, 0.2448275862068956, -0.2982758620689664, -0.7379310344827595, -1.5741379310344836, -1.9275862068965526, -0.7293103448275872, 1.9431034482758611, 0.5206896551724126, -2.6517241379310352, -0.5568965517241384, 0.6931034482758612, 1.3482758620689648, 0.30517241379310267, -1.7293103448275873, -0.6258620689655182, -1.0224137931034492, -0.4275862068965527, -0.15172413793103542, -0.2724137931034491, 0.5551724137931027]
  out "Off-Line  Bin Readings":dbl[](array[numeric])=[177.0, 171.0, 186.0, 177.0, 204.0, 228.0, 264.0, 288.0, 308.0, 336.0, 359.0, 349.0, 359.0, 384.0, 362.0, 396.0, 334.0, 350.0, 357.0, 358.0, 349.0, 314.0, 361.0, 340.0, 360.0, 330.0, 319.0, 295.0, 315.0, 308.0, 298.0, 298.0, 276.0, 288.0, 280.0, 264.0, 256.0, 252.0, 248.0, 216.0, 200.0, 206.0, 172.0, 195.0, 167.0, 144.0, 173.0, 161.0, 154.0, 134.0, 153.0, 158.0, 163.0, 151.0, 144.0, 159.0, 146.0, 152.0, 147.0, 128.0, 139.0, 118.0, 143.0, 121.0, 150.0, 138.0, 117.0, 121.0, 135.0, 124.0, 120.0, 122.0, 133.0, 140.0, 121.0, 118.0, 106.0, 129.0, 123.0, 137.0, 140.0, 138.0, 123.0, 115.0, 120.0, 128.0, 152.0, 342.0, 519.0, 506.0, 413.0, 430.0, 267.0, 145.0, 115.0, 117.0, 114.0, 108.0, 117.0, 101.0, 103.0, 132.0, 93.0, 133.0, 118.0, 124.0, 132.0, 120.0, 121.0, 135.0, 194.0, 183.0, 206.0, 205.0, 162.0, 122.0, 114.0, 106.0, 123.0, 97.0, 121.0, 102.0, 122.0, 112.0, 115.0, 114.0, 97.0, 127.0, 107.0, 113.0, 116.0, 98.0, 120.0, 104.0, 102.0, 113.0, 113.0, 110.0, 123.0, 106.0, 96.0, 109.0, 98.0, 118.0, 104.0, 104.0, 118.0, 130.0, 96.0, 94.0, 98.0, 99.0, 103.0, 102.0, 104.0, 124.0, 116.0, 120.0, 109.0, 95.0, 99.0, 105.0, 103.0, 119.0, 118.0, 111.0, 110.0, 93.0, 119.0, 83.0, 108.0, 111.0, 115.0, 112.0, 102.0, 103.0, 104.0, 107.0, 109.0, 99.0, 102.0, 100.0, 126.0, 101.0, 115.0, 110.0, 106.0, 107.0, 105.0, 103.0, 102.0, 106.0, 108.0, 117.0, 127.0, 112.0, 93.0, 130.0, 110.0, 102.0, 105.0, 108.0, 105.0, 109.0, 113.0, 128.0, 83.0, 105.0, 98.0, 108.0, 107.0, 122.0, 112.0, 105.0, 112.0, 111.0, 102.0, 98.0, 113.0, 90.0, 108.0, 128.0, 98.0, 106.0, 101.0, 121.0, 103.0, 120.0, 106.0, 110.0, 98.0, 123.0, 116.0, 106.0, 107.0, 115.0, 104.0, 107.0, 113.0, 95.0, 122.0, 104.0, 124.0, 104.0, 116.0, 111.0, 107.0, 121.0, 120.0, 118.0, 124.0, 120.0, 105.0, 108.0, 105.0, 106.0, 119.0, 97.0, 106.0, 109.0, 104.0, 98.0, 103.0, 118.0, 102.0, 97.0, 87.0, 87.0, 113.0, 124.0, 108.0, 110.0, 111.0, 95.0, 106.0, 95.0, 106.0, 88.0, 103.0]
  out "Off-Line Smoothed":dbl[](array[numeric])=[63.63882681564251, 65.58575418994417, 76.6891061452514, 92.50893854748603, 109.33016759776532, 128.6597765363128, 154.62206703910613, 188.87625698324018, 223.40139664804454, 246.44888268156404, 257.03268156424565, 261.7966480446926, 267.7226256983238, 271.38882681564223, 267.39162011173164, 260.3790502793295, 255.8678770949719, 254.99497206703896, 256.65977653631273, 256.46843575418984, 253.58715083798867, 250.053631284916, 245.45027932960875, 241.10670391061433, 236.06480446927355, 230.44888268156416, 223.91536312849155, 217.19748603351945, 210.48100558659206, 203.636033519553, 196.85810055865917, 190.26452513966478, 184.21564245810055, 177.9865921787709, 172.27150837988825, 165.4935754189944, 157.0857541899441, 145.59134078212287, 129.59134078212287, 110.51452513966476, 93.17234636871505, 80.09553072625698, 69.93631284916204, 62.78687150837994, 58.644413407821276, 55.79525139664808, 52.70586592178773, 49.964245810055885, 47.55363128491621, 45.54106145251397, 43.61927374301677, 41.69050279329609, 40.58156424581006, 38.53407821229051, 36.06759776536313, 34.668156424581014, 33.4586592178771, 32.51312849162012, 31.035474860335203, 29.578770949720678, 28.97262569832403, 27.83296089385475, 26.691899441340784, 25.7854748603352, 24.62765363128492, 24.0173184357542, 23.858100558659228, 24.15558659217878, 24.103910614525148, 22.5941340782123, 21.507541899441346, 21.22402234636872, 20.08296089385475, 18.169553072625696, 17.265921787709487, 16.57318435754189, 15.923743016759767, 15.818994413407811, 15.725418994413397, 15.105307262569823, 14.218435754189937, 14.439106145251388, 18.89301675977653, 38.02290502793296, 69.93212290502794, 120.52569832402236, 280.27569832402236, 541.2170391061452, 666.0983240223464, 550.9949720670392, 379.36508379888255, 259.9963687150837, 155.9572625698324, 71.24497206703913, 24.784078212290503, 9.775698324022347, 7.638826815642457, 6.788268156424579, 6.696089385474858, 6.968435754189944, 6.996368715083799, 8.434916201117318, 12.622067039106142, 15.676536312849151, 14.556424581005576, 12.624860335195528, 16.559217877094973, 31.38184357541899, 46.746368715083804, 50.6709497206704, 52.007541899441335, 58.01592178770949, 55.48938547486033, 37.54525139664804, 15.974022346368718, 5.10949720670391, 3.5005586592178766, 3.20167597765363, 3.5089385474860313, 3.7282122905027912, 3.564804469273744, 3.0773743016759787, 2.7715083798882683, 2.5522346368715083, 2.842737430167598, 3.464245810055866, 3.363687150837989, 3.437709497206704, 2.37486033519553, 2.0620111731843567, 1.901396648044692, 1.9083798882681564, 2.2966480446927378, 2.387430167597765, 2.876256983240223, 2.4726256983240225, 1.8916201117318439, 1.7882681564245813, 1.2547486033519557, 1.0075418994413405, 1.810614525139665, 2.0662011173184363, 2.4782122905027926, 2.8511173184357546, 2.137430167597766, 1.761731843575419, 1.9698324022346376, 1.5801675977653633, 1.4391061452513965, 1.366480446927374, 0.7114525139664797, 0.441899441340782, 1.1527932960893856, 1.531284916201117, 1.0689944134078206, 1.3594972067039104, 1.2296089385474858, 0.5508379888268151, 0.5801675977653629, 0.9712290502793295, 0.9837988826815636, 1.1122905027932954, 1.661173184357542, 1.2645251396648045, 0.913966480446927, 0.8203910614525132, 0.6150837988826812, 1.1737430167597764, 1.2365921787709497, 0.3525139664804469, 0.38743016759776505, 0.4041899441340778, 0.3022346368715082, 0.07458100558659175, -0.1097765363128495, 0.5187150837988825, 1.5215083798882685, 1.5606145251396653, 0.3636871508379887, 0.5759776536312842, 1.1849162011173173, 1.0243016759776529, 1.12486033519553, 1.401396648044693, 0.6472067039106156, 0.13324022346368752, 0.7337988826815642, 0.7268156424581005, -0.10279329608938553, -0.11396648044692759, -0.101396648044693, -0.27318435754189957, 0.03407821229050292, 0.12206703910614534, 0.15139664804469266, 0.5396648044692736, 0.8553072625698324, 1.3553072625698328, 1.0717877094972073, 0.4670391061452515, 0.549441340782123, 0.41536312849162044, 0.3357541899441342, 0.42932960893854755, 0.24217877094972057, -0.38770949720670406, -0.060893854748603315, 0.04944134078212295, 0.06480446927374284, 0.3650837988826814, -0.05111731843575412, 0.06899441340782109, 0.4782122905027934, 0.5061452513966485, 0.4209497206703911, 0.5298882681564243, 0.5522346368715081, 0.6402234636871506, 0.8189944134078206, 0.3594972067039103, 0.6053072625698319, 0.5159217877094968, -0.003631284916201051, 0.09972067039106139, 0.13882681564245766, 0.13044692737430136, -0.13212290502793284, -0.33044692737430165, 0.22541899441340804, 0.09553072625698333, 0.1569832402234635, 0.7589385474860335, 0.17513966480446952, -0.34720670391061437, -0.15865921787709497, 0.6108938547486031, 0.3343575418994411, -0.4966480446927377, 0.1988826815642456, 0.5089385474860336, 0.05363128491620123, 0.07178770949720688, 0.26312849162011187, 0.5229050279329609, 0.4600558659217877, 0.006145251396648149, 0.3385474860335196, 0.4293296089385475, 0.003351955307262615, -0.07486033519553065, -0.15726256983240197, 0.27150837988826826, 0.10251396648044703, 0.25335195530726257, 0.2533519553072624, 0.028491620111731814, 0.43212290502793305, -0.006424581005586599, -0.19357541899441344, 0.3902234636871506, 0.09413407821229036, -0.33044692737430154, 0.2505586592178771, 0.4921787709497206, -0.5972067039106147, -0.870949720670391, 0.457262569832402, 0.6807262569832397, 0.5354748603351954, 0.1458100558659216, -0.07206703910614518, -0.19776536312849155, -0.3513966480446928, 0.4768156424581005, -0.09581005586592234, -0.6474860335195535, 0.1918994413407821]
  out "On-Line  Smoothed":dbl[](array[numeric])=[39.28938547486035, 37.15111731843578, 39.73212290502795, 45.891340782122896, 51.12458100558658, 56.15111731843574, 63.737709497206666, 73.69301675977651, 83.90949720670392, 88.67346368715086, 87.26564245810059, 85.32011173184358, 83.62877094972066, 80.6594972067039, 76.02821229050278, 71.19720670391058, 67.6162011173184, 65.18463687150833, 63.34525139664801, 61.35642458100556, 59.162290502793276, 56.095251396648024, 52.67765363128489, 49.941620111731815, 48.11480446927372, 45.96256983240224, 43.62178770949722, 40.72513966480449, 37.71117318435756, 35.10083798882684, 32.90949720670393, 31.339664804469294, 29.46536312849164, 27.145530726257, 24.96117318435755, 23.253072625698323, 21.50586592178771, 19.662290502793297, 17.261452513966486, 14.937430167597771, 12.95279329608939, 11.033798882681566, 9.329888268156424, 7.526815642458098, 6.56871508379888, 6.294972067039104, 6.952793296089383, 7.181843575418991, 6.254469273743016, 5.598044692737433, 5.370391061452516, 5.54078212290503, 5.656703910614528, 4.771229050279331, 4.2907821229050285, 4.769832402234638, 4.5351955307262575, 3.7740223463687164, 3.7810055865921797, 3.69441340782123, 3.2027932960893866, 3.410893854748604, 3.5854748603351974, 3.2740223463687164, 2.836871508379889, 2.1134078212290515, 1.8424581005586598, 2.753072625698325, 2.5756983240223477, 2.28100558659218, 2.977932960893857, 2.976536312849163, 2.5324022346368724, 2.401117318435756, 2.091061452513968, 1.9695530726257, 2.0170391061452526, 2.4234636871508393, 2.5701117318435767, 1.3885474860335203, 1.318715083798883, 2.0505586592178786, 2.138547486033522, 3.716759776536314, 6.588268156424579, 12.456983240223465, 30.857821229050295, 60.72653631284917, 75.1203910614525, 61.9290502793296, 41.96675977653632, 28.243296089385485, 16.73631284916201, 7.056145251396648, 2.6818435754189958, 0.9025139664804477, 0.6301675977653636, 0.8689944134078217, 0.8215083798882686, 0.9011173184357547, 1.0798882681564257, 1.3340782122905046, 1.16368715083799, 1.332681564245811, 1.6399441340782137, 1.335474860335197, 1.220949720670392, 2.860614525139666, 4.503072625698325, 4.794972067039108, 5.3787709497206695, 5.5784916201117305, 5.456983240223462, 4.085474860335195, 1.4290502793296098, -0.4689944134078202, -1.0695530726256972, -0.15614525139664773, 0.08966480446927391, -0.11145251396648007, -0.13659217877094926, 0.05893854748603386, 0.3550279329608942, 1.0659217877094982, 1.2027932960893863, 0.7768156424581014, 0.48910614525139745, -0.3865921787709491, -0.6114525139664797, -0.12262569832402177, 0.5156424581005594, 0.4835195530726263, 0.7000000000000004, 0.6622905027932965, 0.1483240223463692, 0.1720670391061456, -0.610055865921787, -0.4452513966480437, 0.35502793296089435, 1.09245810055866, 0.7907821229050287, 0.024022346368715336, 0.04357541899441378, 0.15251396648044746, 0.3312849162011177, -0.44804469273742975, -0.4229050279329605, 0.7139664804469281, 0.32569832402234733, -0.3209497206703905, 0.6050279329608944, 0.4444134078212294, -0.1673184357541897, 0.08966480446927413, 0.6301675977653637, 0.6706703910614531, 0.5966480446927381, 0.2921787709497214, 0.0519553072625705, -0.006703910614524272, 0.02821229050279392, 0.9779329608938556, 0.11899441340782224, -0.3474860335195525, 0.3662011173184363, 0.07709497206703952, 0.11201117318435799, 0.18044692737430218, -0.20223463687150794, 0.012849162011173698, 0.13715083798882727, 0.08826815642458144, 0.5351955307262576, -0.07932960893854663, -0.2092178770949714, -0.10586592178770912, 0.19581005586592254, 0.45418994413407904, 0.417877094972068, 0.2921787709497215, -0.48715083798882647, -0.7734636871508371, -0.35167597765363057, -0.11284916201117302, -0.5723463687150832, -0.450837988826815, -0.10307262569832366, 0.13994413407821282, 0.21815642458100615, 0.08826815642458131, 0.16927374301675996, 0.08826815642458144, 0.07011173184357616, 0.5198324022346378, 0.47793296089385545, 0.2921787709497212, 0.2307262569832409, 0.05893854748603402, 0.282402234636872, 0.21815642458100604, -0.45921787709497136, -0.3432960893854742, 0.10782122905027955, 0.17346368715083837, 0.16368715083798943, 0.4639664804469283, 0.32709497206703997, 0.024022346368715697, 0.04636871508379961, -0.5276536312849154, 0.06173184357542005, 0.7530726256983247, 0.4360335195530729, -0.029050279329608603, -0.43128491620111664, -0.25530726256983166, -0.2092178770949716, -0.06536312849161977, -0.08212290502793265, -0.2245810055865918, -0.06815642458100493, -0.07653631284916176, 0.12039106145251396, 0.44860335195530787, 0.051955307262570694, 0.35782122905028024, 0.4779329608938554, -0.4536312849162008, -0.7860335195530718, 0.18463687150838154, 0.4276536312849173, -0.04301675977653596, 0.6748603351955315, 0.5268156424581012, 0.47234636871508434, 0.5393854748603357, 0.3592178770949723, 0.06452513966480483, 0.22513966480447, 0.785195530726258, 0.8689944134078221, 0.7656424581005592, 0.2139664804469279, -0.25391061452513913, -0.572346368715083, -0.801396648044692, -1.0416201117318429, -0.8377094972067036, -0.2511173184357542, 0.31312849162011214, 0.9304469273743019, 0.5743016759776538, 0.2153631284916205, 0.3983240223463691, 0.22793296089385523, 0.04357541899441439, -0.3041899441340773, -0.41592178770949684, -0.7078212290502787, -0.5737430167597759, 0.537988826815643, 0.49888268156424637, -0.1086592178770946, -0.010893854748603007, -0.44106145251396556, -1.2036312849161999, -0.9550279329608928, -0.3502793296089376, 0.01983240223463753, 0.5561452513966487, -0.11983240223463598, -0.48296089385474783, -0.3502793296089377, -0.6002793296089379, 0.13575418994413435, 0.6650837988826819, 0.5142458100558663]
  out "On-Line Bin Readings":dbl[](array[numeric])=[138.0, 162.0, 148.0, 149.0, 141.0, 171.0, 171.0, 183.0, 183.0, 203.0, 183.0, 180.0, 202.0, 186.0, 183.0, 155.0, 159.0, 165.0, 165.0, 174.0, 140.0, 142.0, 165.0, 156.0, 147.0, 139.0, 169.0, 143.0, 142.0, 131.0, 140.0, 123.0, 135.0, 144.0, 136.0, 122.0, 132.0, 144.0, 112.0, 120.0, 103.0, 131.0, 107.0, 102.0, 105.0, 118.0, 127.0, 106.0, 133.0, 118.0, 114.0, 108.0, 82.0, 110.0, 96.0, 106.0, 104.0, 117.0, 119.0, 118.0, 102.0, 105.0, 83.0, 106.0, 121.0, 116.0, 116.0, 96.0, 124.0, 97.0, 101.0, 120.0, 108.0, 114.0, 95.0, 93.0, 118.0, 101.0, 114.0, 108.0, 120.0, 107.0, 119.0, 117.0, 85.0, 120.0, 116.0, 138.0, 155.0, 161.0, 145.0, 149.0, 104.0, 117.0, 110.0, 114.0, 108.0, 97.0, 104.0, 128.0, 109.0, 106.0, 92.0, 99.0, 111.0, 140.0, 105.0, 118.0, 104.0, 104.0, 112.0, 118.0, 123.0, 117.0, 127.0, 123.0, 102.0, 115.0, 111.0, 99.0, 114.0, 121.0, 118.0, 109.0, 115.0, 113.0, 126.0, 103.0, 106.0, 99.0, 94.0, 100.0, 112.0, 108.0, 110.0, 125.0, 108.0, 97.0, 104.0, 107.0, 104.0, 116.0, 93.0, 101.0, 98.0, 100.0, 120.0, 120.0, 106.0, 112.0, 98.0, 111.0, 118.0, 106.0, 106.0, 127.0, 102.0, 123.0, 103.0, 88.0, 122.0, 78.0, 130.0, 121.0, 103.0, 116.0, 131.0, 103.0, 105.0, 108.0, 94.0, 109.0, 101.0, 120.0, 98.0, 111.0, 114.0, 91.0, 99.0, 90.0, 98.0, 104.0, 103.0, 122.0, 111.0, 106.0, 108.0, 101.0, 116.0, 90.0, 95.0, 113.0, 102.0, 97.0, 112.0, 112.0, 107.0, 111.0, 100.0, 108.0, 129.0, 113.0, 88.0, 98.0, 85.0, 111.0, 107.0, 112.0, 105.0, 102.0, 87.0, 93.0, 121.0, 112.0, 102.0, 94.0, 106.0, 104.0, 106.0, 97.0, 109.0, 118.0, 109.0, 98.0, 104.0, 94.0, 100.0, 120.0, 119.0, 96.0, 94.0, 102.0, 98.0, 104.0, 101.0, 117.0, 107.0, 99.0, 100.0, 93.0, 116.0, 113.0, 106.0, 111.0, 114.0, 104.0, 112.0, 114.0, 110.0, 99.0, 101.0, 110.0, 111.0, 106.0, 124.0, 111.0, 110.0, 112.0, 115.0, 112.0, 119.0, 98.0, 106.0, 121.0, 107.0, 124.0, 87.0, 97.0, 109.0, 91.0, 106.0, 110.0, 132.0, 87.0, 115.0, 109.0, 122.0, 100.0, 112.0]
  out "Range Corrected Altitude Array":dbl[](array[numeric])=[5625.0, 22500.0, 50625.0, 90000.0, 140625.0, 202500.0, 275625.0, 360000.0, 455625.0, 562500.0, 680625.0, 810000.0, 950625.0, 1102500.0, 1265625.0, 1440000.0, 1625625.0, 1822500.0, 2030625.0, 2250000.0, 2480625.0, 2722500.0, 2975625.0, 3240000.0, 3515625.0, 3802500.0, 4100625.0, 4410000.0, 4730625.0, 5062500.0, 5405625.0, 5760000.0, 6125625.0, 6502500.0, 6890625.0, 7290000.0, 7700625.0, 8122500.0, 8555625.0, 9000000.0, 9455625.0, 9922500.0, 10400625.0, 10890000.0, 11390625.0, 11902500.0, 12425625.0, 12960000.0, 13505625.0, 14062500.0, 14630625.0, 15210000.0, 15800625.0, 16402500.0, 17015625.0, 17640000.0, 18275625.0, 18922500.0, 19580625.0, 20250000.0, 20930625.0, 21622500.0, 22325625.0, 23040000.0, 23765625.0, 24502500.0, 25250625.0, 26010000.0, 26780625.0, 27562500.0, 28355625.0, 29160000.0, 29975625.0, 30802500.0, 31640625.0, 32490000.0, 33350625.0, 34222500.0, 35105625.0, 36000000.0, 36905625.0, 37822500.0, 38750625.0, 39690000.0, 40640625.0, 41602500.0, 42575625.0, 43560000.0, 44555625.0, 45562500.0, 46580625.0, 47610000.0, 48650625.0, 49702500.0, 50765625.0, 51840000.0, 52925625.0, 54022500.0, 55130625.0, 56250000.0, 57380625.0, 58522500.0, 59675625.0, 60840000.0, 62015625.0, 63202500.0, 64400625.0, 65610000.0, 66830625.0, 68062500.0, 69305625.0, 70560000.0, 71825625.0, 73102500.0, 74390625.0, 75690000.0, 77000625.0, 78322500.0, 79655625.0, 81000000.0, 82355625.0, 83722500.0, 85100625.0, 86490000.0, 87890625.0, 89302500.0, 90725625.0, 92160000.0, 93605625.0, 95062500.0, 96530625.0, 98010000.0, 99500625.0, 101002500.0, 102515625.0, 104040000.0, 105575625.0, 107122500.0, 108680625.0, 110250000.0, 111830625.0, 113422500.0, 115025625.0, 116640000.0, 118265625.0, 119902500.0, 121550625.0, 123210000.0, 124880625.0, 126562500.0, 128255625.0, 129960000.0, 131675625.0, 133402500.0, 135140625.0, 136890000.0, 138650625.0, 140422500.0, 142205625.0, 144000000.0, 145805625.0, 147622500.0, 149450625.0, 151290000.0, 153140625.0, 155002500.0, 156875625.0, 158760000.0, 160655625.0, 162562500.0, 164480625.0, 166410000.0, 168350625.0, 170302500.0, 172265625.0, 174240000.0, 176225625.0, 178222500.0, 180230625.0, 182250000.0, 184280625.0, 186322500.0, 188375625.0, 190440000.0, 192515625.0, 194602500.0, 196700625.0, 198810000.0, 200930625.0, 203062500.0, 205205625.0, 207360000.0, 209525625.0, 211702500.0, 213890625.0, 216090000.0, 218300625.0, 220522500.0, 222755625.0, 225000000.0, 227255625.0, 229522500.0, 231800625.0, 234090000.0, 236390625.0, 238702500.0, 241025625.0, 243360000.0, 245705625.0, 248062500.0, 250430625.0, 252810000.0, 255200625.0, 257602500.0, 260015625.0, 262440000.0, 264875625.0, 267322500.0, 269780625.0, 272250000.0, 274730625.0, 277222500.0, 279725625.0, 282240000.0, 284765625.0, 287302500.0, 289850625.0, 292410000.0, 294980625.0, 297562500.0, 300155625.0, 302760000.0, 305375625.0, 308002500.0, 310640625.0, 313290000.0, 315950625.0, 318622500.0, 321305625.0, 324000000.0, 326705625.0, 329422500.0, 332150625.0, 334890000.0, 337640625.0, 340402500.0, 343175625.0, 345960000.0, 348755625.0, 351562500.0, 354380625.0, 357210000.0, 360050625.0, 362902500.0, 365765625.0, 368640000.0, 371525625.0, 374422500.0, 377330625.0, 380250000.0, 383180625.0, 386122500.0, 389075625.0, 392040000.0, 395015625.0, 398002500.0, 401000625.0, 404010000.0, 407030625.0, 410062500.0, 413105625.0, 416160000.0, 419225625.0, 422302500.0, 425390625.0, 428490000.0, 431600625.0, 434722500.0, 437855625.0, 441000000.0]
  out "Altitude Array (km)":dbl[](array[numeric])=[0.075, 0.15, 0.22499999999999998, 0.3, 0.375, 0.45, 0.5249999999999999, 0.6, 0.6749999999999999, 0.7499999999999999, 0.825, 0.8999999999999999, 0.9749999999999999, 1.05, 1.125, 1.2, 1.275, 1.3499999999999999, 1.4249999999999998, 1.5, 1.575, 1.65, 1.7249999999999999, 1.7999999999999998, 1.8749999999999998, 1.95, 2.025, 2.1, 2.1750000000000003, 2.25, 2.325, 2.4, 2.475, 2.5500000000000003, 2.625, 2.7, 2.775, 2.85, 2.9250000000000003, 3.0, 3.075, 3.15, 3.225, 3.3000000000000003, 3.375, 3.45, 3.525, 3.6, 3.675, 3.75, 3.825, 3.9, 3.975, 4.05, 4.125, 4.2, 4.275, 4.35, 4.425, 4.5, 4.575, 4.65, 4.725, 4.8, 4.875, 4.95, 5.025, 5.1, 5.175, 5.25, 5.325, 5.4, 5.475, 5.55, 5.625, 5.7, 5.775, 5.85, 5.925, 6.0, 6.075, 6.15, 6.225, 6.3, 6.375, 6.45, 6.525, 6.6, 6.675, 6.75, 6.825, 6.9, 6.975, 7.05, 7.125, 7.2, 7.2749999999999995, 7.35, 7.425, 7.5, 7.575, 7.6499999999999995, 7.725, 7.8, 7.875, 7.95, 8.024999999999999, 8.1, 8.174999999999999, 8.249999999999998, 8.325, 8.399999999999999, 8.475, 8.549999999999999, 8.624999999999998, 8.7, 8.774999999999999, 8.85, 8.924999999999999, 8.999999999999998, 9.075, 9.149999999999999, 9.225, 9.299999999999999, 9.374999999999998, 9.45, 9.524999999999999, 9.6, 9.674999999999999, 9.749999999999998, 9.825, 9.899999999999999, 9.975, 10.049999999999999, 10.124999999999998, 10.2, 10.274999999999999, 10.35, 10.424999999999999, 10.499999999999998, 10.575, 10.649999999999999, 10.725, 10.799999999999999, 10.874999999999998, 10.95, 11.024999999999999, 11.1, 11.174999999999999, 11.249999999999998, 11.325, 11.399999999999999, 11.475, 11.549999999999999, 11.624999999999998, 11.7, 11.774999999999999, 11.85, 11.924999999999999, 11.999999999999998, 12.075, 12.149999999999999, 12.225, 12.299999999999999, 12.374999999999998, 12.45, 12.524999999999999, 12.6, 12.674999999999999, 12.749999999999998, 12.825, 12.899999999999999, 12.975, 13.049999999999999, 13.124999999999998, 13.2, 13.274999999999999, 13.35, 13.424999999999999, 13.499999999999998, 13.575, 13.649999999999999, 13.725, 13.799999999999999, 13.874999999999998, 13.95, 14.024999999999999, 14.1, 14.174999999999999, 14.249999999999998, 14.325, 14.399999999999999, 14.474999999999998, 14.549999999999999, 14.624999999999998, 14.7, 14.774999999999999, 14.849999999999998, 14.924999999999999, 14.999999999999998, 15.075, 15.149999999999999, 15.224999999999998, 15.299999999999999, 15.374999999999998, 15.45, 15.524999999999999, 15.599999999999998, 15.674999999999999, 15.749999999999998, 15.825, 15.899999999999999, 15.974999999999998, 16.05, 16.125, 16.2, 16.275, 16.349999999999998, 16.424999999999997, 16.5, 16.575, 16.65, 16.724999999999998, 16.799999999999997, 16.875, 16.95, 17.025, 17.099999999999998, 17.174999999999997, 17.25, 17.325, 17.4, 17.474999999999998, 17.549999999999997, 17.625, 17.7, 17.775, 17.849999999999998, 17.924999999999997, 18.0, 18.075, 18.15, 18.224999999999998, 18.299999999999997, 18.375, 18.45, 18.525, 18.599999999999998, 18.674999999999997, 18.75, 18.825, 18.9, 18.974999999999998, 19.049999999999997, 19.125, 19.2, 19.275, 19.349999999999998, 19.424999999999997, 19.5, 19.575, 19.65, 19.724999999999998, 19.799999999999997, 19.875, 19.95, 20.025, 20.099999999999998, 20.174999999999997, 20.25, 20.325, 20.4, 20.474999999999998, 20.549999999999997, 20.625, 20.7, 20.775, 20.849999999999998, 20.924999999999997, 21.0]
  out "Offline Pulse Energy":dbl=4.296208571428571
  out "Online Pulse Energy":dbl=4.293568571428572
  in  "Instrument Control":T5(tab)=enum."WS"
  out "Readings":T6={"OnLineTEC"=23.2074528, "OnLineLD"=0.172277346, "OffLineTEC"=29.5224247, "OffLineLD"=0.173082039, "EtalonTEC"=29.3255577, "TSOA-TEC"=19.0006657, "Pro8000"=TRUE, "OnLine TEC"=TRUE, "OnLine LD"=TRUE, "OffLine TEC"=TRUE, "OffLine LD"=TRUE, "Etalon TEC"=TRUE, "TSOA TEC"=TRUE} {"OffLineLD" format="%.4g"; "OnLineLD" format="%.4g"; "TSOA-TEC" format="%.3g"; "EtalonTEC" format="%.3g"; "OffLineTEC" format="%.3g"; "OnLineTEC" format="%.3g"}
  in  "Settings":T7={"Module"=enum."On Line TEC", "OnLineTEC"=23.201149999999803, "OnLineLD"=0.1722, "OffLineTEC"=29.50044999999965, "OffLineLD"=0.173, "EtalonTEC"=29.0, "TSOA-TEC"=19.0} {"OffLineLD" min=0.0 max=0.175 step=0.001 format="%.3p"; "OnLineLD" min=0.0 max=0.175 step=0.001 format="%.3p"; "TSOA-TEC" format="%.2g"; "EtalonTEC" format="%.2g"; "OffLineTEC" min=0.0 max=30.0 step=0.1 format="%.3g"; "OnLineTEC" min=0.0 max=30.0 step=0.1 format="%.3g"}
  in  "Device In":refnum<visa-resource-name>="Pro8000"
  in  "Pulse B Polarity":enum32{"Low", "High"}(ring)=enum."High"
  in  "Pulse A Delay(ns)":u32=1040 min=80 max=327600
  in  "Pulse B Delay(ns)":u32=170000 min=80 max=327600 step=1
  in  "Accumulation Delay(ns)":u32=10 min=10 max=1270 step=1
  in  "Sync Pulse Polarity":enum32{"Low", "High"}(ring)=enum."High"
  in  "Pulse A Polarity":enum32{"Low", "High"}(ring)=enum."High"
  in  "Number of Bins":u32=280 min=2 max=4095 step=1
  in  "Number of Accumulates":u32=10000 min=1 max=32767 step=1
  in  "Time Resolution Per Bin(ns)":u32=500 min=5 max=1063 step=1
  out "AMCS_Profile":i32=59266
  in  "Lambda On Set (nm)":dbl=828.194 format="%.5f"
  out "Lambda On Read (nm)":dbl=828.1940227293112 format="%.5f"
  out "Lambda Off Read (nm)":dbl=828.293376674672 format="%.5f"
  in  "Lambda Off Set (nm)":dbl=828.29345 format="%#.5f"
  in  "Bristol In":i32=5
  out "Bristol Out":i32
  out "WL_Difference":dbl=2.27293112402549e-05 format="%#_3e"
  out "WL Difference off":dbl=-7.332532800319314e-05 format="%#_3e"
  out "Wavelength Lock Online":bool=TRUE
  out "Wavelength Lock Offline":bool=TRUE
  in  "calculate absorption cross sections":bool
  in  "Online_Tol":dbl=0.0001 format="%#_15g"
  in  "Cancel online":bool
  in  "Offline_Tol":dbl=0.0001 format="%#_15g"
  in  "Cancel Offline":bool
  in  "y":dbl=0.00025 format="%#_6p"
  in  "Smoothing Range":dbl=150.0
  in  "Total DIAL Integration Time (Minutes)":i32=3
  in  "Data Reads (number of loops)":i32=1
  in  "Total Aerosol Integration Time (Minutes)":dbl=0.5
  in  "Scalar Wait Time":u32
  out "Smoothed Bins":dbl=2.0
  in  "NewportIn":string
  in  "logging":bool
  out "Newport Device Key":string="1918-R 15120"
  in  "SampleSize":i32=2
  out "NewportRef":refnum<k24>
  in  "Switch Comm Port":refnum<visa-resource-name>="COM3"
  out "FF_On_Ref":refnum<file>
  out "FF_On_Ptr":i64=622336 format="%.2p"
  out "FF_Off_Ref":refnum<file>
  out "FF_Off_Ptr":i64=622336 format="%.2p"
  out "NF_On_Ref":refnum<file>
  out "NF_On_Ptr":i64=622336 format="%.2p"
  out "NF_Off_Ref":refnum<file>
  out "NF_Off_Ptr":i64=622336 format="%.2p"
  out "DataOpen":bool=TRUE
  out "File Path_Far Field (out)":string="C:\\Users\\H2ODial\\Desktop\\SharedTeleWVData\\161101FF\\18"
  out "File Path_Near Field (out)":string="C:\\Users\\H2ODial\\Desktop\\SharedTeleWVData\\161101NF\\18"
  in  "Data File DIR (in)":string="C:\\Users\\H2ODial\\Desktop\\SharedTeleWVData\\"
  out "TRHP":T8={"Temp C"=13.42460317460317, "RelH %"=37.02686202686203, "Press hPa"=833.7225274725275, "AbH g/m^3"=4.258241758241758}
  in  "WS visa":refnum<visa-resource-name>="LuftWS"
  in  "WS_On/Off":bool=TRUE
  in  "bins":u32=280 min=2 max=4095 step=1
  out "y offset":u32=10
  in  "ns scale":u32=500
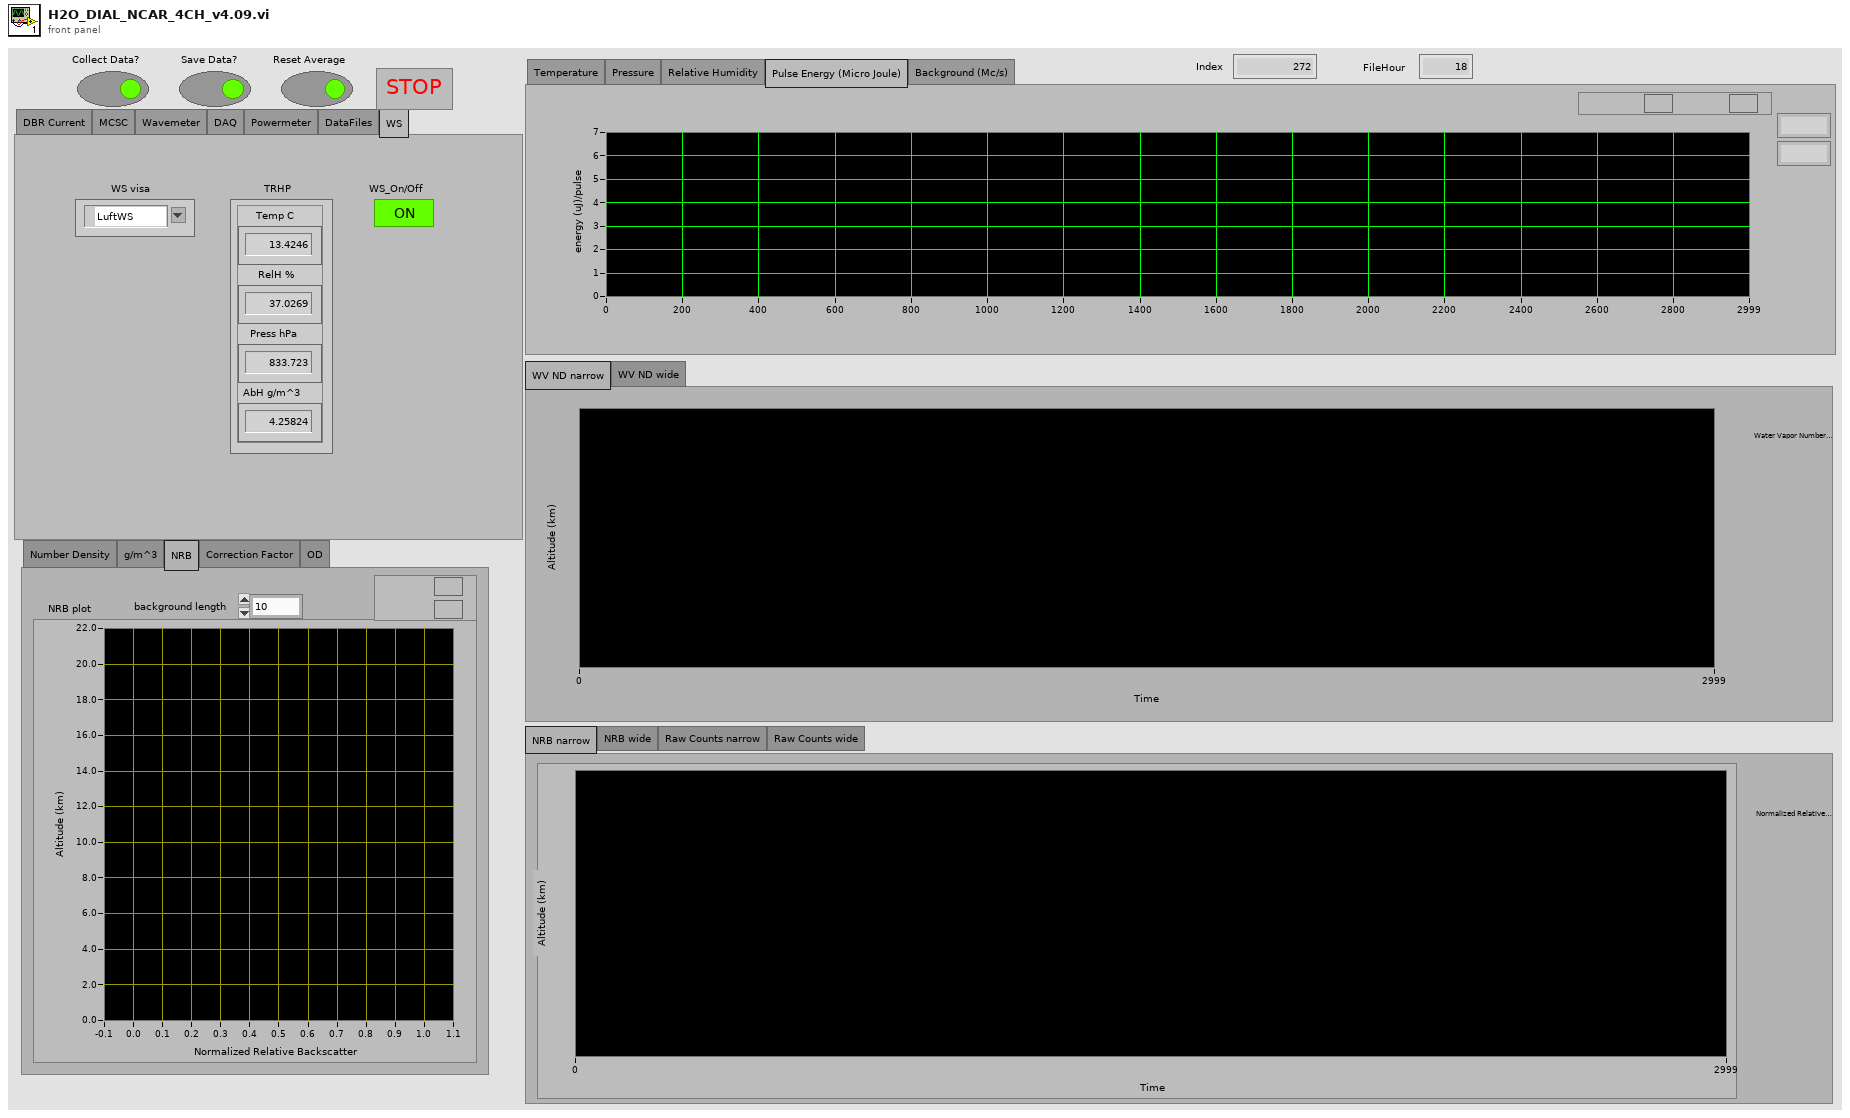
[diagram p1: front panel]
types:
  T1 = enum32{"NRB narrow", "NRB wide", "Raw Counts narrow", "Raw Counts wide"}
  T2 = enum32{"Number Density", "g/m^3", "NRB", "Correction Factor", "OD"}
  T3 = enum32{"Temperature", "Pressure", "Relative Humidity", "Pulse Energy (Micro Joule)", "Background (Mc/s)"}
  T4 = cluster{"Online Pulse Energy":dbl, "Pulse Energy Offline":dbl}
  T5 = enum32{"DBR Current", "MCSC", "Wavemeter", "DAQ", "Powermeter", "DataFiles", "WS"}
  T6 = cluster{"OnLineTEC":dbl, "OnLineLD":dbl, "OffLineTEC":dbl, "OffLineLD":dbl, "EtalonTEC":dbl, "TSOA-TEC":dbl, "Pro8000":bool, "OnLine TEC":bool, "OnLine LD":bool, "OffLine TEC":bool, "OffLine LD":bool, "Etalon TEC":bool, "TSOA TEC":bool}
  T7 = cluster{"Module":enum16{"On Line TEC", "On Line LD", "Off Line TEC", "Off Line LD", "Etalon TEC", "TSOA TEC"}, "OnLineTEC":dbl, "OnLineLD":dbl, "OffLineTEC":dbl, "OffLineLD":dbl, "EtalonTEC":dbl, "TSOA-TEC":dbl}
  T8 = cluster{"Temp C":dbl, "RelH %":dbl, "Press hPa":dbl, "AbH g/m^3":dbl}
  T9 = enum16{"Open_TL", "Close_TL", "Verify_ID", "TEC_Sensor", "SET", "READ", "ON", "OFF", "Set_Limits", "Read_Limits", "Enable_Status", "Read_Status"}
  T10 = enum16{"Initialize ILX", "Set ON T", "Set Off T", "Set ON I", "Set Off I", "Set On Lim", "Set Off Lim", "Read ILX", "TEC ON/OFF", "LASER ON/OFF", "Status?", "ILX OFF"}
  T11 = enum16{"open", "replace", "create", "open or create", "replace or create", "replace or create with confirmation"}
  T12 = enum16{"On Line TEC", "On Line LD", "Off Line TEC", "Off Line LD", "Etalon TEC", "TSOA TEC"}
  T13 = cluster{"Temp":dbl, "RelH":dbl, "Press":dbl, "AbH":dbl}
  T14 = typedef "LVDateTimeRec.ctl" = cluster{"fractional second":dbl, "second":i32, "minute":i32, "hour":i32, "day of month":i32, "month":i32, "year":i32, "day of week":i32, "day of year":i32, "DST":i32}
  T15 = cluster{"Online Pulse Energy":dbl, "Offline Pulse Energy":dbl}
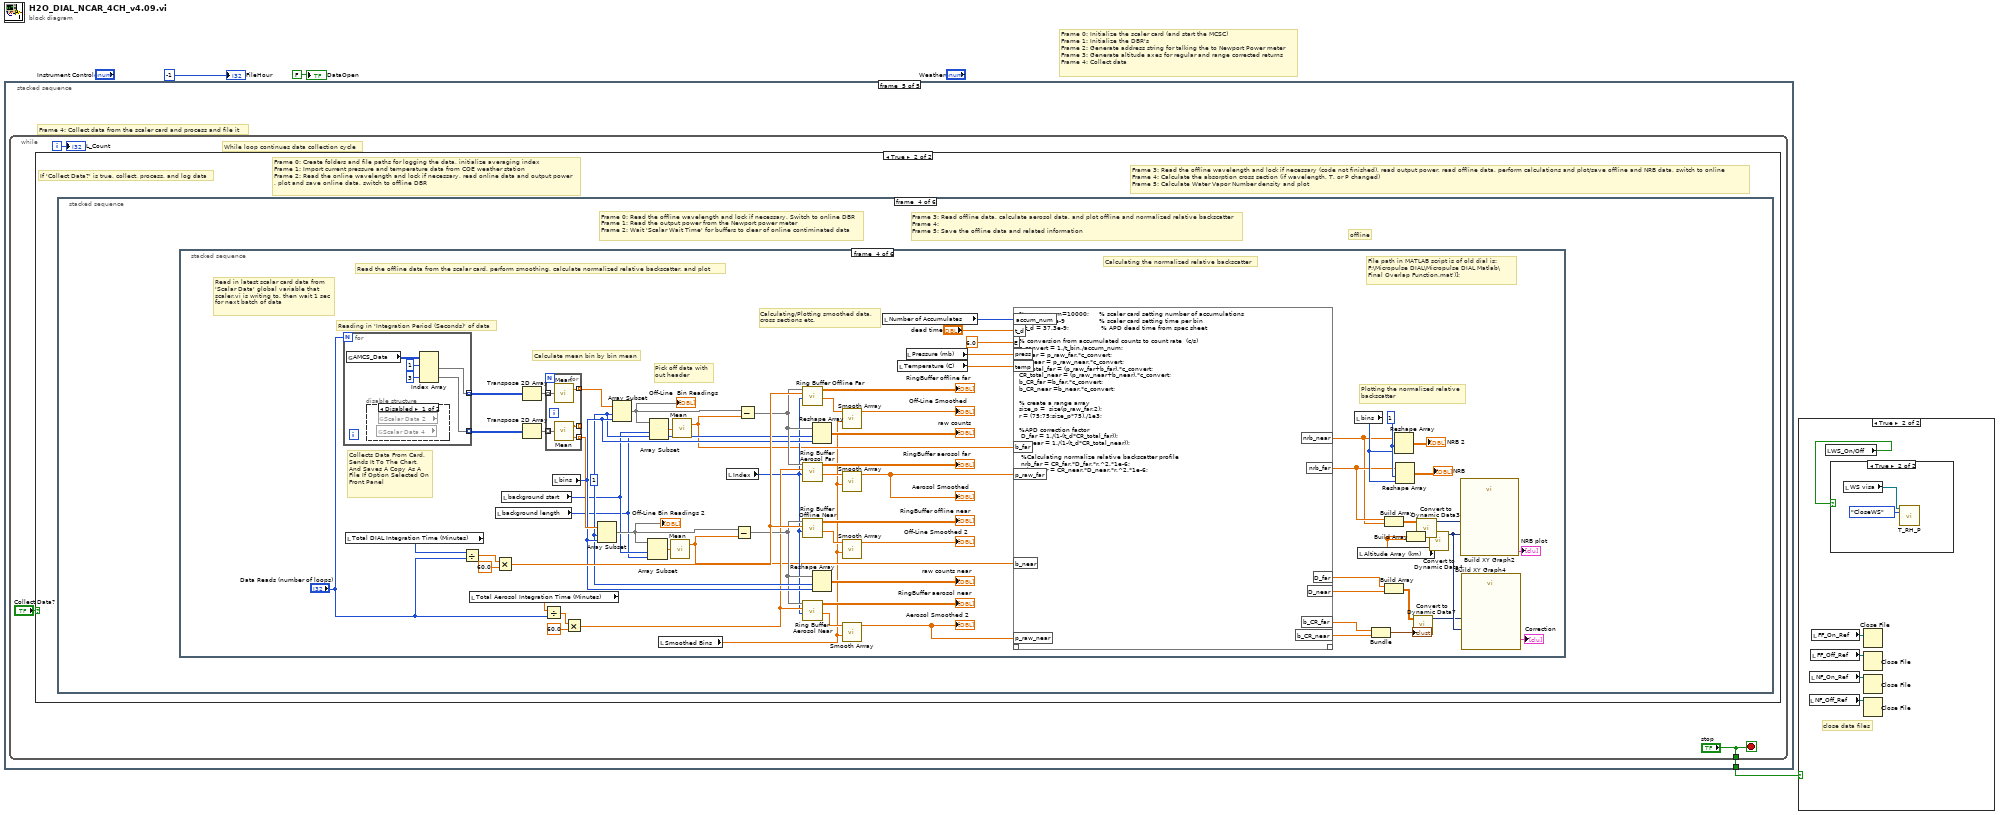
[diagram p0: block diagram]
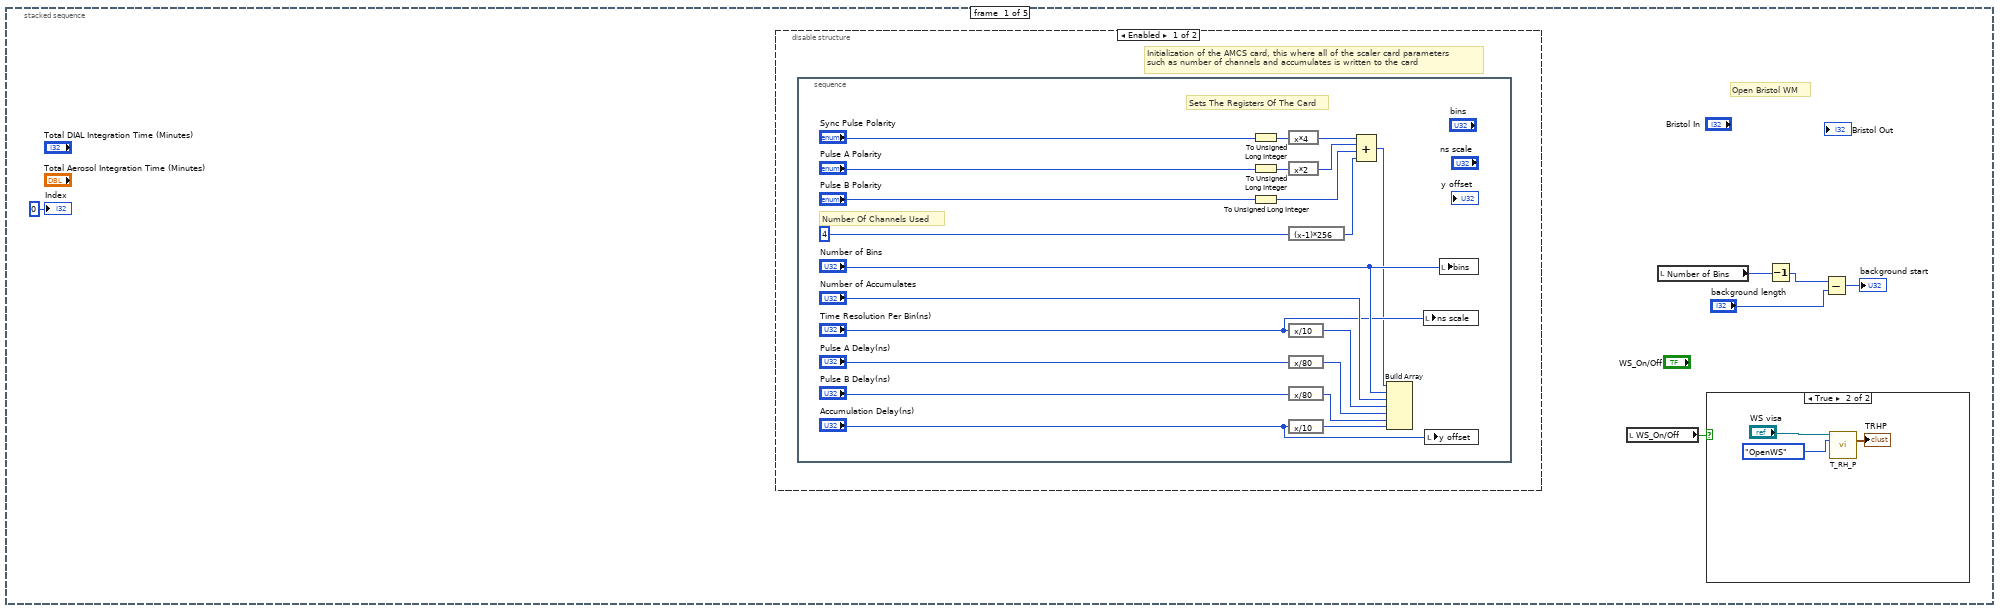
[diagram p4: hidden frame]
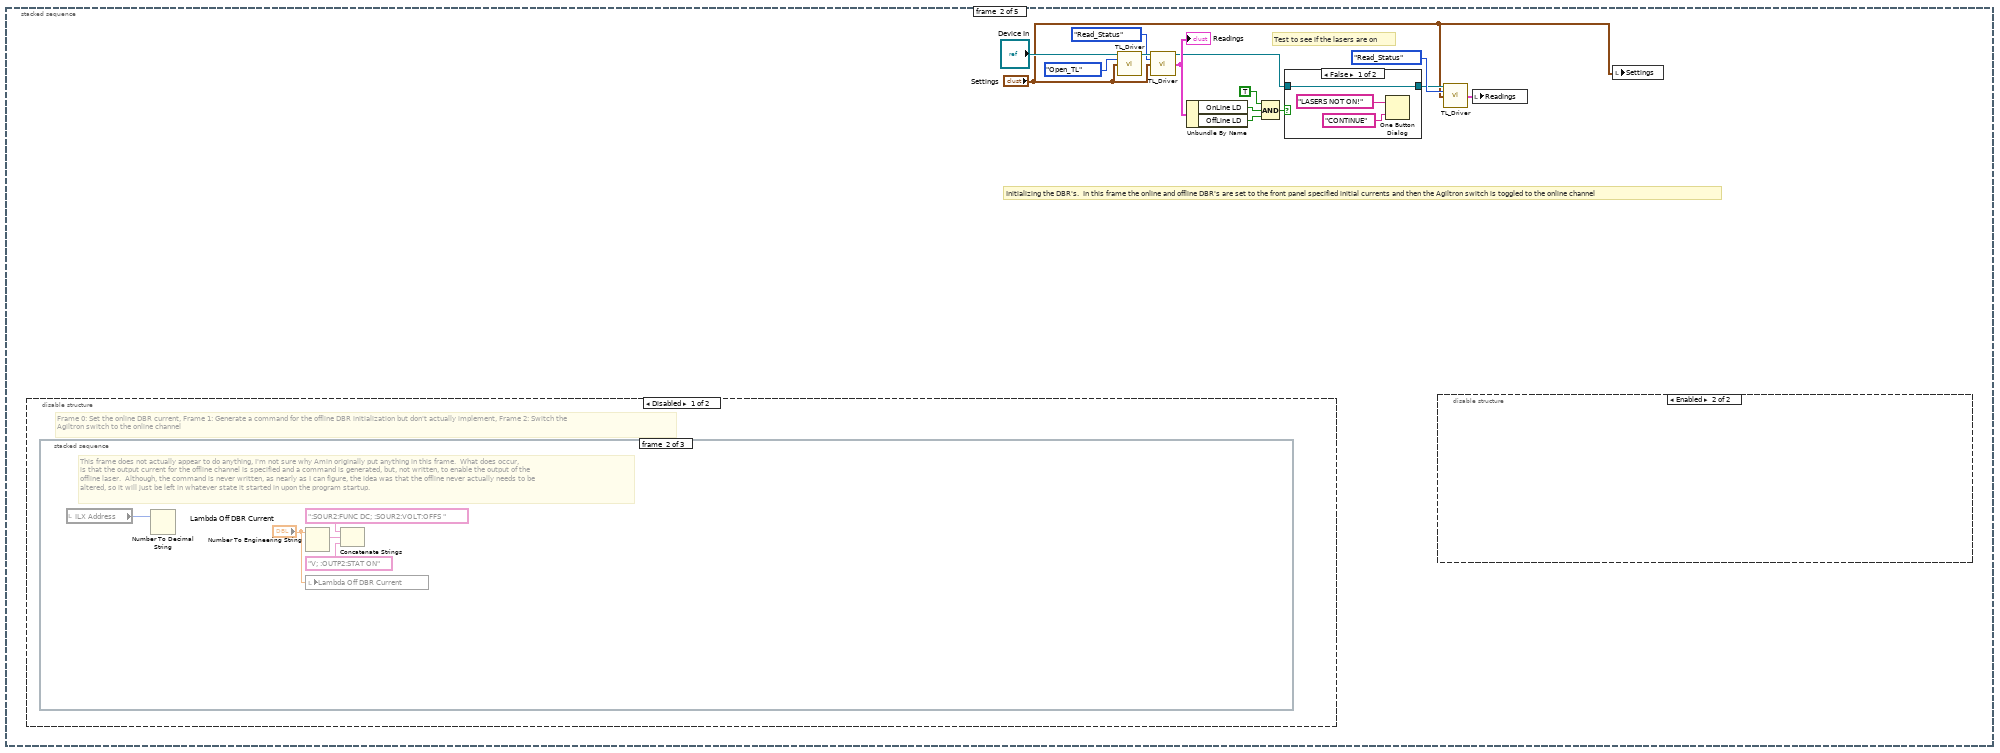
[diagram p7: hidden frame]
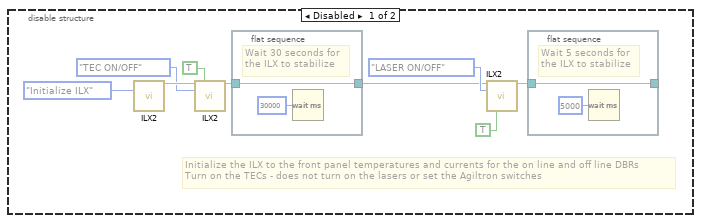
[diagram p9: hidden frame]
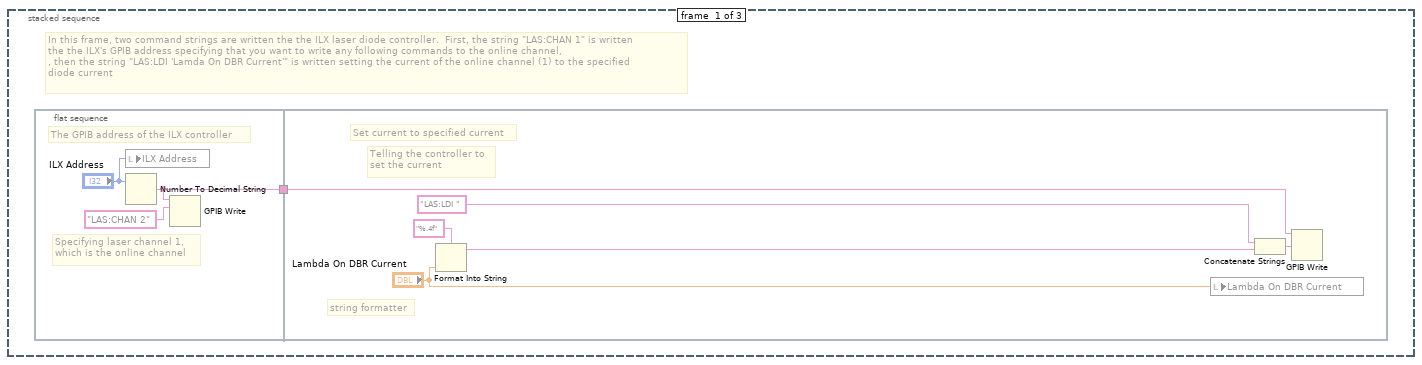
[diagram p10: hidden frame]
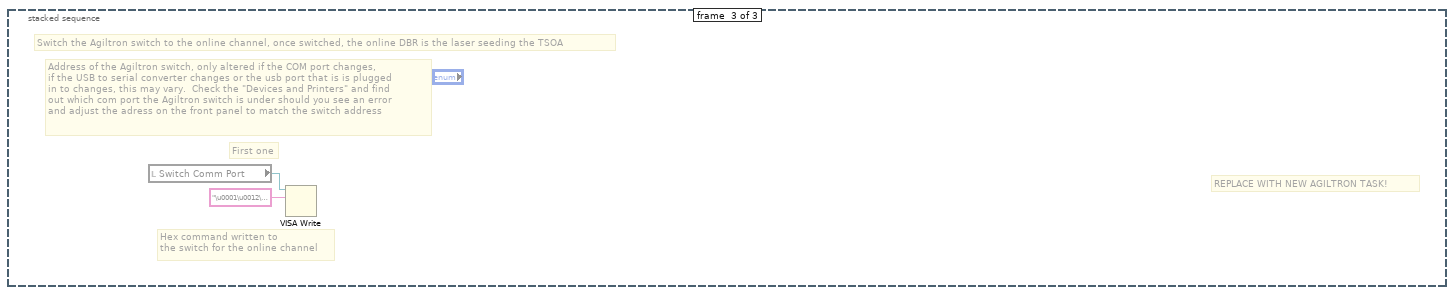
[diagram p11: hidden frame]
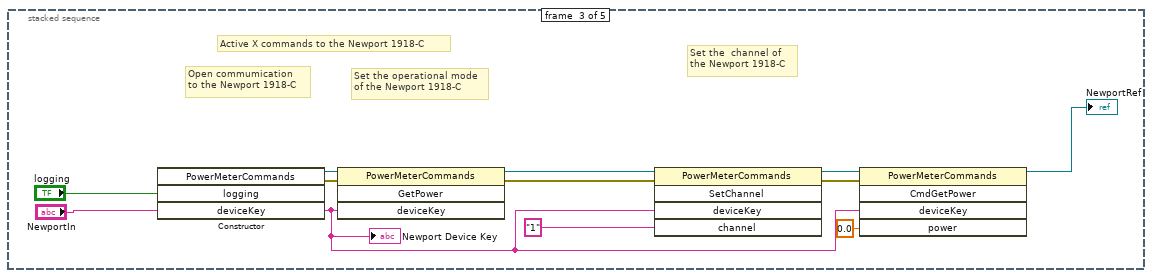
[diagram p13: hidden frame]
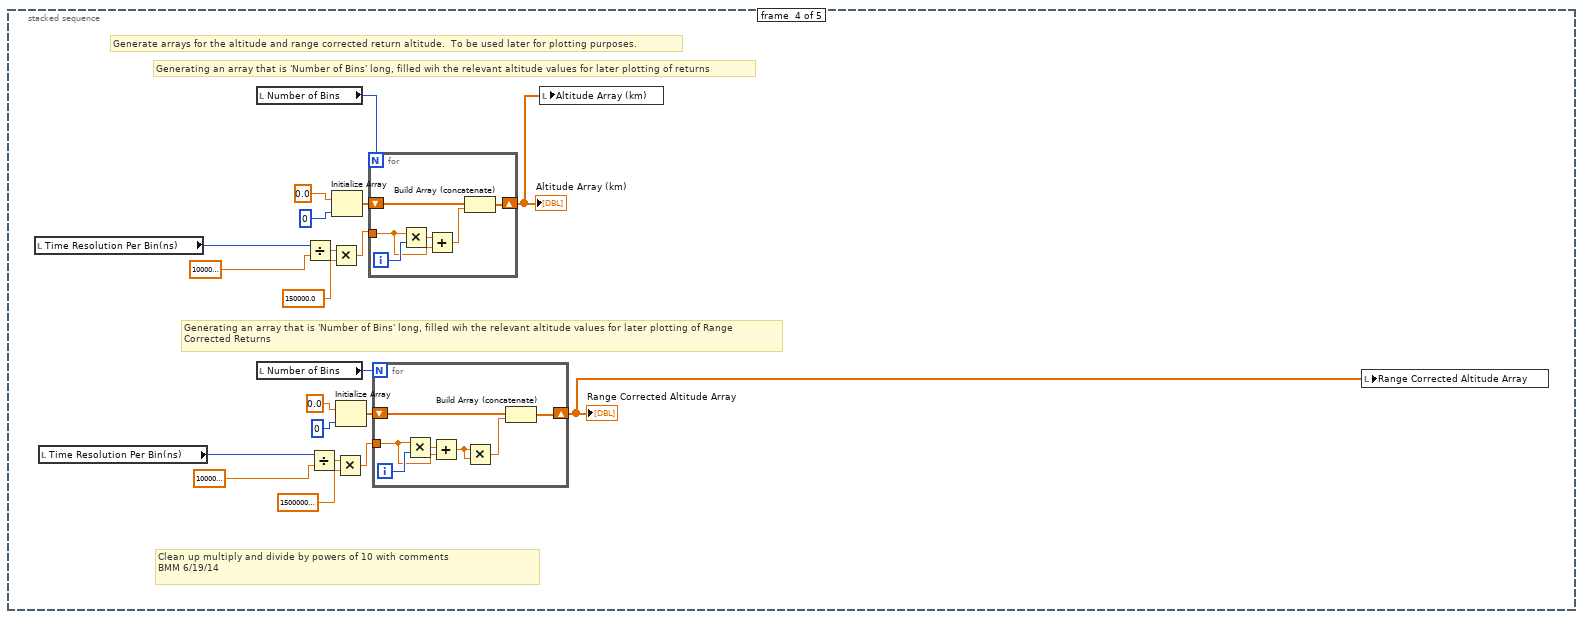
[diagram p14: hidden frame]
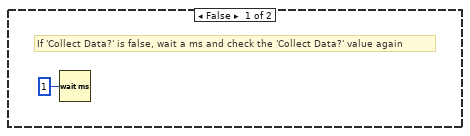
[diagram p15: hidden frame]
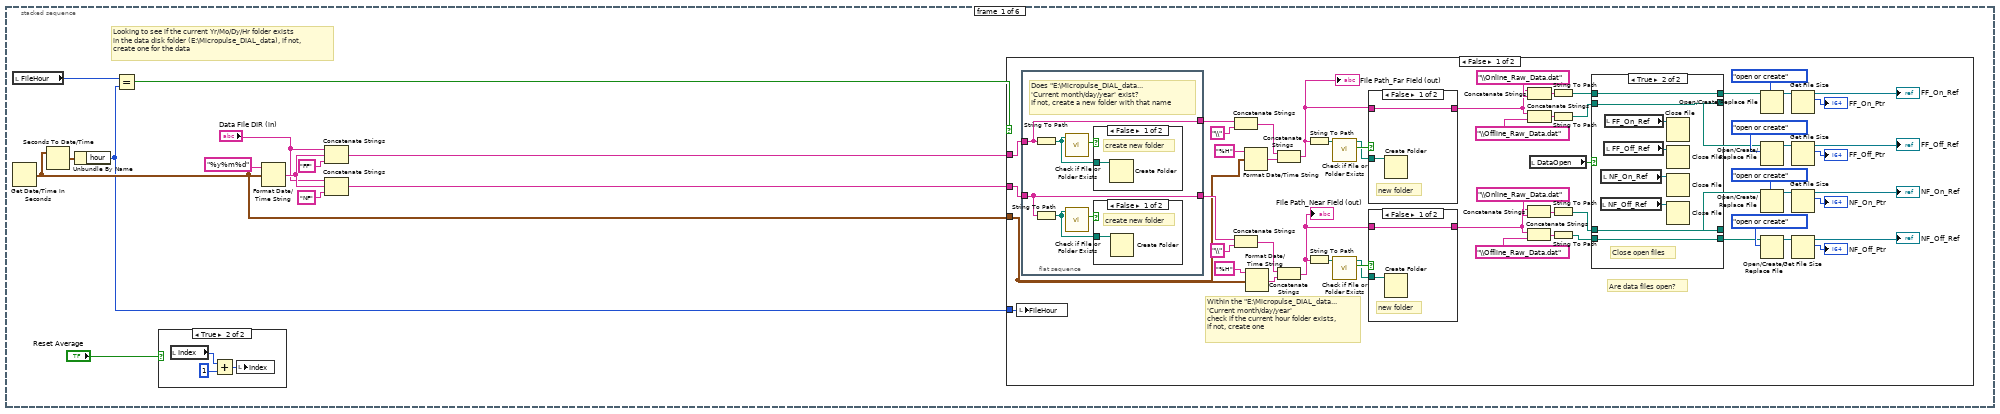
[diagram p16: hidden frame]
diagram:
  # "Frame 0: Initialize the scaler card (and start the MCSC)\nFrame 1: Initialize the DBR's\nFrame 2: Generate address string for talking the to Newport Power meter\nFrame 3: Generate altitude axes for regular and range corrected returns\nFrame 4: Collect data"
  n1 = stacked-sequence {
    tunnel: [_ _ _ _ w127] -> w3
    frame #0 {
      # "Open Bristol WM"
      n2 = disable-structure shown="Enabled" {
        frame Enabled {
          # "Initialization of the AMCS card, this where all of the scaler card parameters\nsuch as number of channels and accumulates is written to the card"
          n3 = stacked-sequence {
            frame #0 {
              # "Sets The Registers Of The Card"
              # "Number Of Channels Used"
              n4 = To Unsigned Long Integer(number="Sync Pulse Polarity") -> (unsigned 32bit integer=w13:u32)
              n5 = To Unsigned Long Integer(number="Pulse A Polarity") -> (unsigned 32bit integer=w17:u32)
              n6 = To Unsigned Long Integer(number="Pulse B Polarity") -> (unsigned 32bit integer=w15:u32)
              n7 = expression code="x*4"(w13) -> (w22:u32)
              n8 = expression code="x*2"(w17) -> (w21:u32)
              n9 = expression code="(x-1)*256"(u32 4 ("Number of Channels Used")) -> (w20:u32)
              n10 = expression code="x/10"("Time Resolution Per Bin(ns)") -> (w24:u32)
              n11 = expression code="x/80"("Pulse A Delay(ns)") -> (w31:u32)
              n12 = expression code="x/80"("Pulse B Delay(ns)") -> (w33:u32)
              n13 = expression code="x/10"("Accumulation Delay(ns)") -> (w32:u32)
              n14 = Compound Arithmetic op=ADD(w22, w21, w15, w20) -> (w19:u32)
              n15 = Build Array(w19, "Number of Bins", "Number of Accumulates", w24, w31, w33, w32) -> ()  [unwired: 1 out]
              n16 = local write "ns scale"("Time Resolution Per Bin(ns)") -> ()
              n17 = local write "y offset"("Accumulation Delay(ns)") -> ()
              n18 = local write "bins"("Number of Bins") -> ()
            }
          }
        }
        frame Disabled {
        }
      }
      n19 = local read "WS_On/Off"() -> (w4:bool)
      n20 = local read "Number of Bins"() -> (w8:u32)
      n21 = case shown="True" w4 {
        frame False {
        }
        frame True {
          n22 = call "T_RH_P.vi"("VISA in"="WS visa", "WS_Commands"=enum16{"OpenWS", "ReadTRHP", "CloseWS"}."OpenWS") -> ("TRHP"=→"TRHP":T13)  [unwired: 11 in, 2 out]
        }
      }
      n23 = Decrement(x=w8) -> (x-1=w7:u32)
      n24 = Subtract(x=w7, y="background length") -> (x-y=→"background start":u32)
      "Index" <- 0 ("Index")
    }
    frame #1 {
      # "Test to see if the lasers are on"
      # "Initializing the DBR's.  In this frame the online and offline DBR's are set to the front panel specified initial currents and then the Agiltron switch is toggled to the online channel"
      n25 = disable-structure shown="Disabled" {
        frame Disabled {
          # "Frame 0: Set the online DBR current, Frame 1: Generate a command for the offline DBR initialization but don't actually implement, Frame 2: Switch the \nAgiltron switch to the online channel"
          n26 = stacked-sequence {
            frame #0 {
              # "In this frame, two command strings are written the the ILX laser diode controller.  First, the string \"LAS:CHAN 1\" is written\nthe the ILX's GPIB address specifying that you want to write any following commands to the online channel,\n, then the string \"LAS:LDI 'Lamda On DBR Current'\" is written setting the current of the online channel (1) to the specified \ndiode current"
              n27 = flat-sequence {
                tunnel: [w67] -> w65
                tunnel: w65 -> [w69]
                frame #0 {
                  # "The GPIB address of the ILX controller"
                  # "Specifying laser channel 1,\nwhich is the online channel"
                  n28 = local write "ILX Address"("ILX Address") -> ()
                  n29 = Number To Decimal String(number="ILX Address") -> (decimal integer string=w67:string)  [unwired: 1 in]
                  n30 = GPIB Write(0:w67, 1:"LAS:CHAN 2") -> ()  [unwired: 3 in, 2 out]
                }
                frame #1 {
                  # "Telling the controller to\nset the current"
                  # "string formatter"
                  # "Set current to specified current"
                  n31 = Format Into String(format string="%.4f" ("Format String"), "Lambda On DBR Current") -> (resulting string=w72:string)  [unwired: 2 in, 1 out]
                  n32 = local write "Lambda On DBR Current"("Lambda On DBR Current") -> ()
                  n33 = Concatenate Strings("LAS:LDI ", w72) -> (w73:string)
                  n34 = GPIB Write(0:w69, 1:w73) -> ()  [unwired: 3 in, 2 out]
                }
              }
            }
            frame #1 {
              # "This frame does not actually appear to do anything, I'm not sure why Amin originally put anything in this frame.  What does occur, \nis that the output current for the offline channel is specified and a command is generated, but, not written, to enable the output of the\noffline laser.  Although, the command is never written, as nearly as I can figure, the idea was that the offline never actually needs to be \naltered, so it will just be left in whatever state it started in upon the program startup."
              n35 = local read "ILX Address"() -> (w75:i32)
              n36 = Number To Decimal String(number=w75) -> ()  [unwired: 1 in, 1 out]
              n37 = Number To Engineering String(4:"Lambda Off DBR Current") -> (0:w79:string)  [unwired: 3 in]
              n38 = local write "Lambda Off DBR Current"("Lambda Off DBR Current") -> ()
              n39 = Concatenate Strings(":SOUR2:FUNC DC; :SOUR2:VOLT:OFFS ", w79, "V; :OUTP2:STAT ON") -> ()  [unwired: 1 out]
            }
            frame #2 {
              # "REPLACE WITH NEW AGILTRON TASK!"
              # "First one"
              # "Address of the Agiltron switch, only altered if the COM port changes,\nif the USB to serial converter changes or the usb port that is is plugged\nin to changes, this may vary.  Check the \"Devices and Printers\" and find \nout which com port the Agiltron switch is under should you see an error \nand adjust the adress on the front panel to match the switch address"
              # "Hex command written to \nthe switch for the online channel"
              # "Switch the Agiltron switch to the online channel, once switched, the online DBR is the laser seeding the TSOA"
              n40 = local read "Switch Comm Port"() -> (w80:refnum<visa-resource-name>)
              n41 = VISA Write(VISA resource name=w80, write buffer="\u0001\u0012\u0000\u0002") -> ()  [unwired: 1 in, 3 out]
            }
          }
        }
        frame Enabled {
        }
      }
      n42 = call "TL_Driver.vi"("Device In"="Device In", "Commands"=T9."Open_TL", "Settings"="Settings") -> ("Device Out"=w45:refnum<visa-resource-name>)  [unwired: 9 in, 3 out]
      n43 = call "TL_Driver.vi"("Device In"=w45, "Commands"=T9."Read_Status", "Settings"="Settings") -> ("Device Out"=w42:refnum<visa-resource-name>, "Readings"=w43:T6)  [unwired: 9 in, 2 out]
      "Readings" <- w43
      n44 = Unbundle By Name(w43) -> ("OnLine LD"=w37:bool, "OffLine LD"=w38:bool)
      n45 = Compound Arithmetic op=AND(TRUE, w37, w38) -> (w36:bool)
      n46 = case shown="False" w36 {
        tunnel: w42 -> [w48 w51]
        tunnel: [w48 w51] -> w40
        frame False {
          n47 = One Button Dialog(message="LASERS NOT ON!", button name ("OK")="CONTINUE") -> ()  [unwired: 1 out]
        }
        frame True {
        }
      }
      n48 = disable-structure shown="Enabled" {
        frame Disabled {
          # "Initialize the ILX to the front panel temperatures and currents for the on line and off line DBRs\nTurn on the TECs - does not turn on the lasers or set the Agiltron switches"
          n49 = call "ILX2.vi"("ILX Command"=T10."Initialize ILX") -> ("Device Out"=w59:refnum<visa-resource-name>)  [unwired: 10 in, 4 out]
          n50 = call "ILX2.vi"("Device In"=w59, "TEC Control"=TRUE, "ILX Command"=T10."TEC ON/OFF") -> ("Device Out"=w56:refnum<visa-resource-name>)  [unwired: 8 in, 4 out]
          n51 = flat-sequence {
            tunnel: w56 -> [w63]
            tunnel: [w63] -> w53
            frame #0 {
              # "Wait 30 seconds for\nthe ILX to stabilize"
              n52 = Wait (ms)(milliseconds to wait=u32 30000) -> ()  [unwired: 1 out]
            }
          }
          n53 = call "ILX2.vi"("Device In"=w53, "ILX Command"=T10."LASER ON/OFF", "Laser Control"=TRUE ("TEC Control")) -> ("Device Out"=w52:refnum<visa-resource-name>)  [unwired: 8 in, 4 out]
          n54 = flat-sequence {
            tunnel: w52 -> [w61]
            tunnel: [w61] -> _
            frame #0 {
              # "Wait 5 seconds for\nthe ILX to stabilize"
              n55 = Wait (ms)(milliseconds to wait=u32 5000) -> ()  [unwired: 1 out]
            }
          }
        }
        frame Enabled {
        }
      }
      n56 = call "TL_Driver.vi"("Device In"=w40, "Commands"=T9."Read_Status", "Settings"="Settings") -> ("Readings"=w34:T6)  [unwired: 9 in, 3 out]
      n57 = local write "Readings"(w34) -> ()
      n58 = local write "Settings"("Settings") -> ()
    }
    frame #2 {
      # "Active X commands to the Newport 1918-C"
      # "Set the  channel of\nthe Newport 1918-C"
      # "Set the operational mode\nof the Newport 1918-C"
      # "Open commumication\nto the Newport 1918-C"
      n59 = constructor class="PowerMeterCommands"("logging"="logging", "deviceKey"="NewportIn") -> (reference out=w93:refnum<k24>, error out=w90:errorcluster, "deviceKey"=w85:string)  [unwired: 3 in, 2 out]
      "Newport Device Key" <- w85
      n60 = invoke class="PowerMeterCommands" method="GetPower"(reference=w93, error in=w90, "deviceKey"=w85) -> (reference out=w92:refnum<k24>, error out=w89:errorcluster)  [unwired: 1 in, 2 out]
      n61 = invoke class="PowerMeterCommands" method="SetChannel"(reference=w92, error in=w89, "deviceKey"=w85, "channel"="1") -> (reference out=w86:refnum<k24>, error out=w88:errorcluster)  [unwired: 1 in, 3 out]
      n62 = invoke class="PowerMeterCommands" method="CmdGetPower"(reference=w86, error in=w88, "deviceKey"=w85, "power"=sgl 0.0) -> (reference out=→"NewportRef":refnum<k24>)  [unwired: 1 in, 4 out]
    }
    frame #3 {
      # "Clean up multiply and divide by powers of 10 with comments\nBMM 6/19/14"
      # "Generating an array that is 'Number of Bins' long, filled wih the relevant altitude values for later plotting of Range \nCorrected Returns"
      # "Generating an array that is 'Number of Bins' long, filled wih the relevant altitude values for later plotting of returns"
      # "Generate arrays for the altitude and range corrected return altitude.  To be used later for plotting purposes."
      n63 = local read "Time Resolution Per Bin(ns)"() -> (w106:u32)
      n64 = local read "Time Resolution Per Bin(ns)"() -> (w96:u32)
      n65 = local read "Number of Bins"() -> (w109:u32)
      n66 = local read "Number of Bins"() -> (w99:u32)
      n67 = Divide(x=w106, y=1000000000.0) -> (x/y=w104:dbl)
      n68 = Divide(x=w96, y=1000000000.0) -> (x/y=w94:dbl)
      n69 = Multiply(x=w104, y=150000.0) -> (x*y=w107:dbl)
      n70 = Initialize Array(0.0, 0) -> (w112:dbl[])
      n71 = Multiply(x=w94, y=150000000.0) -> (x*y=w97:dbl)
      n72 = Initialize Array(0.0, 0) -> (w102:dbl[])
      n73 = for {
        N: w109 -> [_]
        shift-right: [w125] -> w110
        shift-left: w112 -> [w126]
        tunnel: w107 -> [w122]
        i -> [w124]
        n74 = Multiply(x=w122, y=w124) -> (x*y=w123:dbl)
        n75 = Add(x=w123, y=w122) -> (x+y=w121:dbl)
        n76 = Build Array (concatenate)(w126, w121) -> (w125:dbl[])
      }
      "Altitude Array (km)" <- w110
      n77 = for {
        N: w99 -> [_]
        shift-right: [w119] -> w100
        shift-left: w102 -> [w120]
        tunnel: w97 -> [w115]
        i -> [w118]
        n78 = Multiply(x=w115, y=w118) -> (x*y=w116:dbl)
        n79 = Add(x=w116, y=w115) -> (x+y=w114:dbl)
        n80 = Multiply(x=w114, y=w114) -> (x*y=w117:dbl)
        n81 = Build Array (concatenate)(w120, w117) -> (w119:dbl[])
      }
      "Range Corrected Altitude Array" <- w100
      n82 = local write "Altitude Array (km)"(w110) -> ()
      n83 = local write "Range Corrected Altitude Array"(w100) -> ()
    }
    frame #4 {
      # "Frame 4: Collect data from the scaler card and process and file it"
      n84 = while {
        tunnel: ["stop"] -> w127
        i -> [w128]
        stop <- "stop" stop-if-true
        # "While loop continues data collection cycle"
        n85 = case shown="True" "Collect Data?" {
          frame False {
            # "If 'Collect Data?' is false, wait a ms and check the 'Collect Data?' value again"
            n86 = Wait (ms)(milliseconds to wait=u32 1) -> ()  [unwired: 1 out]
          }
          frame True {
            # "Frame 3: Read the offline wavelength and lock if necessary (code not finished), read output power, read offline data, perform calculations and plot/save offline and NRB data, switch to online\nFrame 4: Calculate the absorption cross section (if wavelength, T, or P changed)\nFrame 5: Calculate Water Vapor Number density and plot"
            # "Frame 0: Create folders and file paths for logging the data, initialize averaging index\nFrame 1: Import current pressure and temperature data from COE weather station\nFrame 2: Read the online wavelength and lock if necessary, read online data and output power\n, plot and save online data, switch to offline DBR"
            # "If 'Collect Data?' is true, collect, process, and log data"
            n87 = stacked-sequence {
              frame #0 {
                # "Looking to see if the current Yr/Mo/Dy/Hr folder exists\nin the data disk folder (E:\\Micropulse_DIAL_data), if not,\ncreate one for the data"
                n88 = local read "FileHour"() -> (w141:i32)
                n89 = Get Date/Time In Seconds() -> (seconds since 1Jan1904=w133:timestamp)
                n90 = Seconds To Date/Time(time stamp (now)=w133) -> (date time rec=w143:T14)  [unwired: 1 in]
                n91 = Unbundle By Name(w143) -> ("hour"=w132:i32)
                n92 = Equal?(x=w141, y=w132) -> (x = y?=w142:bool)
                n93 = case shown="True" "Reset Average" {
                  frame False {
                    n94 = local write "Index"(0 ("Index")) -> ()
                  }
                  frame True {
                    n95 = local read "Index"() -> (w231:i32)
                    n96 = Add(x=w231, y=1) -> (x+y=w230:i32)
                    n97 = local write "Index"(w230) -> ()
                  }
                }
                n98 = Format Date/Time String(time format string (%c)="%y%m%d", seconds (now)=w133) -> (date/time string=w137:string)  [unwired: 1 in]
                n99 = Concatenate Strings("Data File DIR (in)", w137, "FF" ("string")) -> (w139:string)
                n100 = Concatenate Strings("Data File DIR (in)", w137, "NF" ("string")) -> (w134:string)
                n101 = case shown="False" w142 {
                  tunnel: w139 -> [w201 _]
                  tunnel: w134 -> [w200 _]
                  tunnel: w133 -> [w187 _]
                  tunnel: w132 -> [w163 _]
                  frame False {
                    # "Are data files open?"
                    # "Within the \"E:\\Micropulse_DIAL_data...\n'Current month/day/year' \ncheck if the current hour folder exists,\nif not, create one"
                    n102 = local write "FileHour"(w163) -> ()
                    n103 = flat-sequence {
                      tunnel: [w221] -> w188
                      tunnel: w201 -> [w220]
                      tunnel: w200 -> [w221]
                      tunnel: [w220] -> w189
                      frame #0 {
                        # "Does \"E:\\Micropulse_DIAL_data...\n'Current month/day/year' exist?\nIf not, create a new folder with that name"
                        n104 = String To Path(string=w220) -> (path=w225:path)
                        n105 = String To Path(string=w221) -> (path=w223:path)
                        n106 = call <vilib>:"Check if File or Folder Exists.vi"("path"=w225) -> ("file or folder exists?"=w224:bool)  [unwired: 8 in, 2 out]
                        n107 = call <vilib>:"Check if File or Folder Exists.vi"("path"=w223) -> ("file or folder exists?"=w222:bool)  [unwired: 8 in, 2 out]
                        n108 = case shown="False" w224 {
                          tunnel: w225 -> [w227 _]
                          frame False {
                            # "create new folder"
                            n109 = Create Folder(path (use dialog)=w227) -> ()  [unwired: 2 in, 3 out]
                          }
                          frame True {
                            # "Folder exists\ndo nothing"
                          }
                        }
                        n110 = case shown="False" w222 {
                          tunnel: w223 -> [w226 _]
                          frame False {
                            # "create new folder"
                            n111 = Create Folder(path (use dialog)=w226) -> ()  [unwired: 2 in, 3 out]
                          }
                          frame True {
                            # "Folder exists\ndo nothing"
                          }
                        }
                      }
                    }
                    n112 = Concatenate Strings(w189, "\\" ("string")) -> (w196:string)
                    n113 = Concatenate Strings(w188, "\\" ("string")) -> (w191:string)
                    n114 = Format Date/Time String(time format string (%c)="%H", seconds (now)=w187) -> (date/time string=w199:string)  [unwired: 1 in]
                    n115 = Format Date/Time String(time format string (%c)="%H", seconds (now)=w187) -> (date/time string=w194:string)  [unwired: 1 in]
                    n116 = Concatenate Strings(w196, w199) -> (w159:string)
                    "File Path_Far Field (out)" <- w159
                    n117 = Concatenate Strings(w191, w194) -> (w160:string)
                    "File Path_Near Field (out)" <- w160
                    n118 = String To Path(string=w159) -> (path=w197:path)
                    n119 = String To Path(string=w160) -> (path=w192:path)
                    n120 = call <vilib>:"Check if File or Folder Exists.vi"("path"=w197) -> ("file or folder exists?"=w186:bool, "dup path"=w184:path)  [unwired: 8 in, 1 out]
                    n121 = call <vilib>:"Check if File or Folder Exists.vi"("path"=w192) -> ("file or folder exists?"=w185:bool, "dup path"=w183:path)  [unwired: 8 in, 1 out]
                    n122 = case shown="False" w186 {
                      tunnel: w184 -> [w218 _]
                      tunnel: w159 -> [w217 w219]
                      tunnel: [w217 w219] -> w157
                      frame False {
                        # "new folder"
                        n123 = Create Folder(path (use dialog)=w218) -> ()  [unwired: 2 in, 3 out]
                      }
                      frame True {
                        # "Folder exists\ndo nothing"
                      }
                    }
                    n124 = case shown="False" w185 {
                      tunnel: w183 -> [w215 _]
                      tunnel: w160 -> [w214 w216]
                      tunnel: [w214 w216] -> w158
                      frame False {
                        # "new folder"
                        n125 = Create Folder(path (use dialog)=w215) -> ()  [unwired: 2 in, 3 out]
                      }
                      frame True {
                        # "Folder exists\ndo nothing"
                      }
                    }
                    n126 = Concatenate Strings(w158, "\\Online_Raw_Data.dat" ("string")) -> (w177:string)
                    n127 = Concatenate Strings(w158, "\\Offline_Raw_Data.dat" ("string")) -> (w176:string)
                    n128 = Concatenate Strings(w157, "\\Online_Raw_Data.dat" ("string")) -> (w182:string)
                    n129 = Concatenate Strings(w157, "\\Offline_Raw_Data.dat" ("string")) -> (w181:string)
                    n130 = local read "DataOpen"() -> (w174:bool)
                    n131 = String To Path(string=w182) -> (path=w173:path)
                    n132 = String To Path(string=w181) -> (path=w172:path)
                    n133 = String To Path(string=w177) -> (path=w171:path)
                    n134 = String To Path(string=w176) -> (path=w170:path)
                    n135 = case shown="True" w174 {
                      tunnel: w173 -> [w205 w209]
                      tunnel: [w205 w209] -> w167
                      tunnel: w172 -> [w204 w208]
                      tunnel: [w204 w208] -> w166
                      tunnel: w171 -> [w203 w207]
                      tunnel: [w203 w207] -> w165
                      tunnel: [w202 w206] -> w164
                      tunnel: w170 -> [w202 w206]
                      frame False {
                        # "No files open\ndo nothing"
                      }
                      frame True {
                        # "Close open files"
                        n136 = local read "NF_Off_Ref"() -> (w211:refnum<file>)
                        n137 = local read "NF_On_Ref"() -> (w210:refnum<file>)
                        n138 = local read "FF_Off_Ref"() -> (w213:refnum<file>)
                        n139 = local read "FF_On_Ref"() -> (w212:refnum<file>)
                        n140 = Close File(refnum=w212) -> ()  [unwired: 1 in, 2 out]
                        n141 = Close File(refnum=w213) -> ()  [unwired: 1 in, 2 out]
                        n142 = Close File(refnum=w210) -> ()  [unwired: 1 in, 2 out]
                        n143 = Close File(refnum=w211) -> ()  [unwired: 1 in, 2 out]
                      }
                    }
                    n144 = Open/Create/Replace File(file path (use dialog)=w167, operation (0:open)=T11."open or create") -> (refnum out=w153:refnum<file>)  [unwired: 4 in, 2 out]
                    n145 = Open/Create/Replace File(file path (use dialog)=w166, operation (0:open)=T11."open or create") -> (refnum out=w154:refnum<file>)  [unwired: 4 in, 2 out]
                    n146 = Open/Create/Replace File(file path (use dialog)=w165, operation (0:open)=T11."open or create") -> (refnum out=w155:refnum<file>)  [unwired: 4 in, 2 out]
                    n147 = Open/Create/Replace File(file path (use dialog)=w164, operation (0:open)=T11."open or create") -> (refnum out=w156:refnum<file>)  [unwired: 4 in, 2 out]
                    n148 = Get File Size(file=w153) -> (refnum out=→"FF_On_Ref":refnum<file>, size (in bytes)=→"FF_On_Ptr":i64)  [unwired: 1 in, 1 out]
                    n149 = Get File Size(file=w154) -> (refnum out=→"FF_Off_Ref":refnum<file>, size (in bytes)=→"FF_Off_Ptr":i64)  [unwired: 1 in, 1 out]
                    n150 = Get File Size(file=w155) -> (refnum out=→"NF_On_Ref":refnum<file>, size (in bytes)=→"NF_On_Ptr":i64)  [unwired: 1 in, 1 out]
                    n151 = Get File Size(file=w156) -> (refnum out=→"NF_Off_Ref":refnum<file>, size (in bytes)=→"NF_Off_Ptr":i64)  [unwired: 1 in, 1 out]
                  }
                  frame True {
                    # "Don't need to do anything!"
                  }
                }
              }
              frame #1 {
                # "Writing and plotting retrieved\nweather parameters"
                # "Matlab script goes online and retrieves most recent press, temp, and relative humidity data \nfrom the weather station on the roof of Cobleigh"
                # "Importing the current weather conditions from the COE weather station"
                n152 = disable-structure shown="Disabled" {
                  frame Disabled {
                    n153 = script code="%try\n%s=urlread('http://www.coe.montana.edu/ee/weather/mostCurrentCSV.php');\n%amin=textscan(s,'%s %s %s %s %s %s %s %s %s %s %s %s %s');\n%data=amin{1}{2};\n%[test remain]=strtok(data,',');\n%remain=str2num(remain);\n%press=remain(3)./1000;\n%temp=remain(5);\n%RH=remain(7);\n%catch\npress=.850;\ntemp=20;\nRH=40;\n%end"() -> ()  [unwired: 1 in, 4 out]
                  }
                  frame Enabled {
                  }
                }
                n154 = local read "WS_On/Off"() -> (w232:bool)
                n155 = case shown="True" w232 {
                  frame False {
                  }
                  frame True {
                    n156 = local read "WS visa"() -> (w237:refnum<visa-resource-name>)
                    n157 = call "T_RH_P.vi"("VISA in"=w237, "WS_Commands"=enum16{"OpenWS", "ReadTRHP", "CloseWS"}."ReadTRHP") -> ("TRHP"=w233:T13)  [unwired: 11 in, 2 out]
                    n158 = local write "TRHP"(w233) -> ()
                    n159 = Unbundle By Name(w233) -> ("Temp"=→"Temperature (C)":dbl, "RelH"=→"Relative Humdity (%)":dbl, "Press"=→"Pressure (mb)":dbl)
                  }
                }
              }
              frame #2 {
                # "Frame 3: Read, process, and plot online data\nFrame 4:\nFrame 5: Write the data to the folders from Frame 0 of outter sequence"
                # "Frame 0: Read the online wavelength and adjust to locking tolerance if out of range, Switch to offline DBR\nFrame 1: Read the output power from the Newport meter, calculate and plot the output pulse energy\nFrame 2: Wait 'Scalar Wait Time' for buffer to clear other wavelength data"
                # "Online"
                n160 = stacked-sequence {
                  frame #0 {
                    # "Read the online wavelength and continue adjusting the online DBR if outside the wavelength tolerance\nuntil it is within tolerance"
                    n161 = while {
                      i -> [w242]
                      stop <- w239 stop-if-true
                      # "Frame 2: Decrement DBR current if above tolerance\nFrame 3: Increment DBR current if below tolerance"
                      # "Frame 0: Read the current wavelength from the wavemeter\nFrame 1: Calculate the difference between desired and actual wavelength"
                      # "Continue reading and adjusting online DBR current until within locking tolerance"
                      n162 = stacked-sequence {
                        tunnel: w242 -> [w244 _ _ _ _]
                        tunnel: [_ _ w257 _ _] -> w240
                        frame #0 {
                          n163 = Equal To 0?(x=w244) -> (x = 0?=w243:bool)
                          n164 = case shown="True" w243 {
                            frame False {
                            }
                            frame True {
                              # "Set the TSOA switch to\namplify the ABSORBING\nwavelength"
                              n165 = Build Array(FALSE ("Boolean")) -> (w245:bool[])
                              n166 = call-poly <vilib>:"DAQmx Write.vi"("task/channels in"=refnum<k21> "BristolWM", "data"=w245) -> ()  [unwired: 11 in, 3 out]
                            }
                          }
                        }
                        frame #1 {
                          # "Reading the wavelength from the wavemeter"
                          n167 = flat-sequence {
                            tunnel: [w250] -> w249
                            tunnel: w249 -> [w253]
                            tunnel: [w252] -> w248
                            tunnel: w248 -> [w256]
                            frame #0 {
                              n168 = local read "Bristol In"() -> (w251:i32)
                              n169 = dll-call lib="C:/Users/H2ODial/Desktop/Shared Telescope WV DIAL Code/bristol/CLDevIface.dll" fn="CLOpenUSBSerialDevice"("commPort"=w251) -> ("return type"=w250:i32)  [unwired: 4 in, 2 out]
                            }
                            frame #1 {
                              n170 = dll-call lib="C:/Users/H2ODial/Desktop/Shared Telescope WV DIAL Code/bristol/CLDevIface.dll" fn="CLGetLambdaReading"("devHandle"=w253) -> ("return type"=→"Lambda On Read (nm)":dbl, "devHandle"=w252:i32)  [unwired: 3 in, 2 out]
                            }
                            frame #2 {
                              n171 = dll-call lib="C:/Users/H2ODial/Desktop/Shared Telescope WV DIAL Code/bristol/CLDevIface.dll" fn="CLCloseDevice"("commPort"=w256) -> ("return type"=w255:i32)  [unwired: 4 in, 2 out]
                              n172 = local write "Bristol Out"(w255) -> ()
                            }
                          }
                        }
                        frame #2 {
                          # "If WL difference is within tolerance, stop looping, and illuminate 'Wavelength Lock Online' indicator"
                          # "Calculating the difference between the actual and desired online wavelength"
                          n173 = local read "Lambda On Read (nm)"() -> (w265:dbl)
                          n174 = local read "Online_Tol"() -> (w262:dbl)
                          n175 = Multiply(x=-1.0, y=w262) -> (x*y=w263:dbl)
                          n176 = Subtract(x=w265, y="Lambda On Set (nm)") -> (x-y=w258:dbl)
                          "WL_Difference" <- w258
                          n177 = Greater?(x=w258, y=w263) -> (0:w259:bool)
                          n178 = Less?(x=w258, y=w262) -> (x < y?=w260:bool)
                          n179 = And(x=w259, y=w260) -> (x .and. y?=w257:bool)
                          "Wavelength Lock Online" <- w257
                        }
                        frame #3 {
                          # "If the wavelength difference is greater that 0.0002 nm, decrement the \nDBR current by 0.01 mA"
                          n180 = local read "WL_Difference"() -> (w268:dbl)
                          n181 = Greater Or Equal?(x=w268, y="Online_Tol") -> (x >= y?=w267:bool)
                          n182 = case shown="True" w267 {
                            frame False {
                              # "Wavelength difference is not greater than 0.0002 nm, do nothing"
                            }
                            frame True {
                              # "Generating a command string\nto decrement the current"
                              # "WL difference is greater than 0.0002 nm,\ndecrement the DBR current by 0.01 mA"
                              n183 = local read "Settings"() -> (w275:T7)
                              n184 = local read "y"() -> (w269:dbl)
                              n185 = Unbundle By Name(w275) -> ("OnLineTEC"=w273:dbl)
                              n186 = local read "Device In"() -> (w270:refnum<visa-resource-name>)
                              n187 = Subtract(x=w273, y=w269) -> (x-y=w272:dbl)
                              n188 = Bundle By Name(cluster=w275, "OnLineTEC"=w272, "Module"=T12."On Line TEC") -> (w277:T7)
                              n189 = call "TL_Driver.vi"("Device In"=w270, "Commands"=T9."SET", "Settings"=w277) -> ("Readings"=w276:T6)  [unwired: 9 in, 3 out]
                              n190 = local write "Settings"(w277) -> ()
                              n191 = local write "Readings"(w276) -> ()
                            }
                          }
                        }
                        frame #4 {
                          # "If WL difference is < 0.0002 nm, increment the DBR current"
                          n192 = local read "Online_Tol"() -> (w279:dbl)
                          n193 = local read "WL_Difference"() -> (w282:dbl)
                          n194 = Multiply(x=-1.0, y=w279) -> (x*y=w278:dbl)
                          n195 = Less Or Equal?(x=w282, y=w278) -> (x <= y?=w281:bool)
                          n196 = case shown="True" w281 {
                            frame False {
                              # "WL difference is no <= to -0.0002 nm, do nothing"
                            }
                            frame True {
                              # "WL difference is < -0.0002,\nincrement the DBR current by 0.01 mA"
                              # "Generating a command string\nto decrement the current"
                              n197 = local read "Settings"() -> (w291:T7)
                              n198 = Unbundle By Name(w291) -> ("OnLineTEC"=w287:dbl)
                              n199 = local read "y"() -> (w283:dbl)
                              n200 = local read "Device In"() -> (w284:refnum<visa-resource-name>)
                              n201 = Add(x=w287, y=w283) -> (x+y=w286:dbl)
                              n202 = Bundle By Name(cluster=w291, "OnLineTEC"=w286, "Module"=T12."On Line TEC") -> (w290:T7)
                              n203 = call "TL_Driver.vi"("Device In"=w284, "Commands"=T9."SET", "Settings"=w290) -> ("Readings"=w289:T6)  [unwired: 9 in, 3 out]
                              n204 = local write "Settings"(w290) -> ()
                              n205 = local write "Readings"(w289) -> ()
                            }
                          }
                        }
                      }
                      n206 = Or(x=w240, y="Cancel online") -> (x .or. y?=w239:bool)
                    }
                  }
                  frame #1 {
                    # "Converting to pulse energy, assumes 5 percent pickoff"
                    # "Reading the Newport Power meter"
                    # "Reading the output power of the laser transmitter from the Newport power meter, once read, convert to corresponding pulse energy and plot"
                    n207 = local read "Newport Device Key"() -> (w296:string)
                    n208 = local read "NewportRef"() -> (w292:refnum<k24>)
                    n209 = disable-structure shown="Disabled" {
                      frame Disabled {
                        # "Plotting the online and offling pulse energies"
                        n210 = local read "Online Pulse Energy"() -> (w307:dbl)
                        n211 = local read "Offline Pulse Energy"() -> (w306:dbl)
                        n212 = Bundle("Online Pulse Energy"=w307, "Offline Pulse Energy"=w306) -> (→"Pulse Energy (Micro Joule)":T15)  [unwired: 1 in]
                      }
                      frame Enabled {
                      }
                    }
                    n213 = Number To Decimal String(number="SampleSize") -> (decimal integer string=w294:string)  [unwired: 1 in]
                    n214 = invoke class="PowerMeterCommands" method="PerformDAQ"(reference=w292, "deviceKey"=w296, "interval"="1", "sampleSize"=w294) -> ("PerformDAQ"=w297:dbl[])  [unwired: 2 in, 5 out]
                    n215 = call-poly <vilib>:"Mean.vi"("X"=w297) -> ("mean"=w295:dbl)  [unwired: 1 out]
                    n216 = Multiply(x=w295, y=1000.0) -> (x*y=w303:dbl)
                    n217 = Divide(x=w303, y=0.05) -> (x/y=w301:dbl)
                    n218 = Divide(x=w301, y=7.0) -> (x/y=→"Online Pulse Energy":dbl)
                  }
                  frame #2 {
                    # "Wait 'Scalar Wait Time' for the next available batch of scalar card data"
                    n219 = local read "AMCS_Profile"() -> (w308:i32)
                    n220 = disable-structure shown="Disabled" {
                      frame Disabled {
                        # "Waiting 'Scalar Wait Time'"
                        n221 = Wait (ms)(milliseconds to wait="Scalar Wait Time") -> ()  [unwired: 1 out]
                      }
                      frame Enabled {
                      }
                    }
                    n222 = while {
                      tunnel: [w315] -> w309
                      tunnel: [w311] -> _
                      tunnel: w308 -> [w311]
                      stop <- w313 stop-if-true
                      n223 = global read "AMCS_Data.vi" "AMCS_Profile"() -> (w315:i32)
                      n224 = Wait (ms)(milliseconds to wait=u32 10) -> ()  [unwired: 1 out]
                      n225 = Equal?(x=w315, y=w311) -> (x = y?=w314:bool)
                      n226 = case shown="False" w314 {
                        tunnel: [TRUE FALSE] -> w313
                        frame False {
                        }
                        frame True {
                        }
                      }
                    }
                    "AMCS_Profile" <- w309
                  }
                  frame #3 {
                    # "convert time per range bin to meters\nand calculate smoothed bins using\nsmoothing range"
                    # "Plotting online cross section and smoothed online data"
                    # "Calculate the bin by bin mean of the data"
                    # "Collect 'Integration Period (Seconds)' number\nof scalar data"
                    # "Reading, processing, and plotting the online data"
                    n227 = local read "Data Reads (number of loops)"() -> (w343:i32)
                    n228 = for {
                      N: w343 -> [_]
                      tunnel: [w364] -> w355 mode=indexing
                      tunnel: [w363] -> w318 mode=indexing
                      # "Scalar Data is retrieved from Global \nVariable that scaler.vi is writing to,"
                      n229 = global read "AMCS_Data.vi" "AMCS_Data"() -> (w367:u16[][])
                      n230 = disable-structure shown="Disabled" {
                        frame Disabled {
                          n231 = global read "Scalar_Data_3.vi" "Scalar Data 3"() -> ()  [unwired: 1 out]
                          n232 = global read "Scalar_Data.vi" "Scalar Data"() -> ()  [unwired: 1 out]
                        }
                        frame Enabled {
                        }
                      }
                      n233 = Index Array(array=w367, index (row) #1=0 ("index (row)"), index (row) #2=2 ("index (row)")) -> (element #1=w364:u16[], element #2=w363:u16[])  [unwired: 2 in]
                    }
                    n234 = Transpose 2D Array(2D array=w355) -> (transposed array=w359:u16[][])
                    n235 = Transpose 2D Array(2D array=w318) -> (transposed array=w341:u16[][])
                    n236 = for {
                      tunnel: w359 -> [w369] mode=indexing
                      tunnel: [w368] -> w360 mode=indexing
                      n237 = call-poly <vilib>:"Mean.vi"("X"=w369) -> ("mean"=w368:dbl)  [unwired: 1 out]
                    }
                    n238 = for {
                      tunnel: w341 -> [w362] mode=indexing
                      tunnel: [w361] -> w342 mode=indexing
                      n239 = call-poly <vilib>:"Mean.vi"("X"=w362) -> ("mean"=w361:dbl)  [unwired: 1 out]
                    }
                    n240 = local read "bins"() -> (w335:u32)
                    n241 = Array Subset(array=w360, index=1 ("dimension size"), length=w335) -> (w347:dbl[])
                    n242 = Array Subset(array=w342, index=1 ("dimension size"), length=w335) -> (w339:dbl[])
                    n243 = local read "background length"() -> (w325:i32)
                    n244 = local read "background start"() -> (w326:u32)
                    n245 = Array Size(array=w347) -> (size(s)=w344:i32)
                    n246 = Array Size(array=w339) -> (size(s)=w336:i32)
                    n247 = Initialize Array(1.0 ("element"), w344) -> (w346:dbl[])
                    n248 = Initialize Array(1.0 ("element"), w336) -> (w338:dbl[])
                    n249 = Multiply(x=w347, y=w346) -> (x*y=w348:dbl[])
                    "On-Line Bin Readings" <- w348
                    n250 = Multiply(x=w339, y=w338) -> (x*y=w329:dbl[])
                    "On-Line Bin Readings 2" <- w329
                    n251 = local read "Total DIAL Integration Time (Minutes)"() -> (w351:i32)
                    n252 = local read "Time Resolution Per Bin(ns)"() -> (w321:u32)
                    n253 = Array Subset(array=w348, index=w326, length=w325) -> (w357:dbl[])
                    n254 = Array Subset(array=w329, index=w326, length=w325) -> (w331:dbl[])
                    n255 = call-poly <vilib>:"Mean.vi"("X"=w357) -> ("mean"=w356:dbl)  [unwired: 1 out]
                    n256 = call-poly <vilib>:"Mean.vi"("X"=w331) -> ("mean"=w332:dbl)  [unwired: 1 out]
                    n257 = Divide(x=w351, y=w343) -> (x/y=w349:dbl)
                    n258 = local read "Index"() -> (w330:i32)
                    n259 = Subtract(x=w348, y=w356) -> (x-y=w353:dbl[])
                    n260 = Subtract(x=w329, y=w332) -> (x-y=w333:dbl[])
                    n261 = To Double Precision Float(number=w321) -> (double precision float=w322:dbl)
                    n262 = Multiply(x=w349, y=60.0) -> (x*y=w327:dbl)
                    n263 = Multiply(x=w322, y=0.15) -> (x*y=w324:dbl)
                    n264 = call "Ring Buffer Online Far.vi"("Index"=w330, "Profiles to Average"=w327, "Input Array"=w353) -> ("AvgArray"=w352:dbl[])  [unwired: 7 in, 1 out]
                    n265 = call "Ring Buffer Online Near.vi"("Index"=w330, "Profiles to Average"=w327, "Input Array"=w333) -> ("AvgArray"=w334:dbl[])  [unwired: 7 in, 1 out]
                    n266 = Divide(x="Smoothing Range", y=w324) -> (x/y=w319:dbl)
                    "Smoothed Bins" <- w319
                    n267 = call "Smooth Arrray.vi"("smooth size"=w319, "Raw Array"=w352) -> ("Smoothed Array"=→"On-Line  Smoothed":dbl[])  [unwired: 9 in]
                    n268 = call "Smooth Arrray.vi"("smooth size"=w319, "Raw Array"=w334) -> ("Smoothed Array"=→"On-Line Smoothed 2":dbl[])  [unwired: 9 in]
                    n269 = disable-structure shown="Disabled" {
                      frame Disabled {
                        n270 = script code="format long;\ncounts=sum(Online);\nif counts >=0.5e6\ntime=time;\nelse\ntime=time\nend"() -> ()  [unwired: 3 in, 2 out]
                      }
                      frame Enabled {
                      }
                    }
                  }
                  frame #4 {
                    # "Toggling the Agiltron switch to the offline DBR seed laser"
                    n271 = disable-structure shown="Disabled" {
                      frame Disabled {
                        n272 = flat-sequence {
                          frame #0 {
                            # "Second one"
                            # "Command the switch to switch to position 2\ncorresponding to the offline DBR"
                            # "Hex string command \ncorrespond to offline"
                            n273 = VISA Write(VISA resource name="Switch Comm Port", write buffer="\u0001\u0012\u0000\u0001") -> ()  [unwired: 1 in, 3 out]
                          }
                        }
                      }
                      frame Enabled {
                      }
                    }
                  }
                  frame #5 {
                    # "Save the recently collected online data if 'Save Data?' is true"
                    n274 = case shown="True" "Save Data?" {
                      frame False {
                        # "'Save Data?' is false, do nothing"
                      }
                      frame True {
                        # "'Save Data?' is true, save onfline data to the Data Disk"
                        # "Write only one copy of data at this time"
                        # "Retrieve Julian Date"
                        n275 = local read "Time Resolution Per Bin(ns)"() -> (w378:u32)
                        n276 = local read "Number of Accumulates"() -> (w376:u32)
                        n277 = local read "Number of Bins"() -> (w377:u32)
                        n278 = local read "Lambda On DBR Current"() -> (w400:dbl)
                        n279 = local read "Lambda On Read (nm)"() -> (w401:dbl)
                        n280 = local read "On-Line Bin Readings 2"() -> (w398:dbl[])
                        n281 = local read "On-Line Bin Readings"() -> (w403:dbl[])
                        n282 = local read "Online Pulse Energy"() -> (w399:dbl)
                        n283 = To Double Precision Float(number=w378) -> (double precision float=w373:dbl)
                        n284 = To Double Precision Float(number=w377) -> (double precision float=w374:dbl)
                        n285 = To Double Precision Float(number=w376) -> (double precision float=w375:dbl)
                        n286 = call "Julian_Date_2.vi"() -> ("Julian Date"=w402:dbl)  [unwired: 11 in]
                        n287 = Build Array (concatenate)(w402, w401, w400, w399, w373, w374, w375, w403) -> (w393:dbl[])
                        n288 = Build Array (concatenate)(w402, w401, w400, w399, w373, w374, w375, w398) -> (w383:dbl[])
                        n289 = local write "DataOpen"(TRUE ("DataOpen")) -> ()
                        n290 = local read "NF_On_Ref"() -> (w381:refnum<file>)
                        n291 = local read "FF_On_Ref"() -> (w397:refnum<file>)
                        n292 = local read "NF_On_Ptr"() -> (w382:i64)
                        n293 = local read "FF_On_Ptr"() -> (w396:i64)
                        n294 = Set File Position(offset (in bytes) (0)=w396, refnum=w397) -> (refnum out=w394:refnum<file>, error out=w391:errorcluster)  [unwired: 2 in]
                        n295 = Set File Position(offset (in bytes) (0)=w382, refnum=w381) -> (refnum out=w387:refnum<file>, error out=w385:errorcluster)  [unwired: 2 in]
                        n296 = Write to Binary File(file (use dialog)=w387, data=w383, error in=w385, 5:FALSE ("prepend array or string size? (T)")) -> (refnum out=w386:refnum<file>, error out=w384:errorcluster)  [unwired: 2 in, 1 out]
                        n297 = Write to Binary File(file (use dialog)=w394, data=w393, error in=w391, 5:FALSE ("prepend array or string size? (T)")) -> (refnum out=w392:refnum<file>, error out=w390:errorcluster)  [unwired: 2 in, 1 out]
                        n298 = Get File Position(4:w384, 7:w386) -> (2:w380:i64)  [unwired: 2 out]
                        n299 = Get File Position(4:w390, 7:w392) -> (2:w389:i64)  [unwired: 2 out]
                        n300 = local write "NF_On_Ptr"(w380) -> ()
                        n301 = local write "FF_On_Ptr"(w389) -> ()
                      }
                    }
                  }
                }
              }
              frame #3 {
                # "Frame 3: Read offline data, calculate aerosol data, and plot offline and normalized relative backscatter\nFrame 4:\nFrame 5: Save the offline data and related information"
                # "Frame 0: Read the offline wavelength and lock if necessary, Switch to online DBR\nFrame 1: Read the output power from the Newport power meter\nFrame 2: Wait 'Scalar Wait Time' for buffers to clear of online contiminated data"
                # "offline"
                n302 = stacked-sequence {
                  frame #0 {
                    # "Every 60 data collection cycles, read the offline DBR wavelength, and if outside of wavelength tolerance, adjust DBR current until within tolerance"
                    n303 = local read "L_Count"() -> (w405:i32)
                    n304 = Quotient & Remainder(x=w405, y=60.0) -> (x-y*floor(x/y)=w406:dbl)  [unwired: 1 out]
                    n305 = Equal To 0?(x=w406) -> (x = 0?=w404:bool)
                    n306 = case shown="True" w404 {
                      frame False {
                      }
                      frame True {
                        n307 = while {
                          i -> [w411]
                          stop <- w409 stop-if-true
                          # "If WL difference is within tolerance, stop looping, and illuminate 'Wavelength Lock Offline' indicator"
                          # "Frame 2: Decrement DBR current if above tolerance\nFrame 3: Increment DBR current if below tolerance"
                          # "Frame 0: Read the current wavelength from the wavemeter\nFrame 1: Calculate the difference between desired and actual wavelength"
                          # "Continue reading and adjusting offline DBR current until within locking tolerance"
                          n308 = stacked-sequence {
                            tunnel: w411 -> [w413 _ _ _ _]
                            tunnel: [_ _ w427 _ _] -> w408
                            frame #0 {
                              n309 = Equal To 0?(x=w413) -> (x = 0?=w412:bool)
                              n310 = case shown="True" w412 {
                                frame False {
                                }
                                frame True {
                                # "Set the TSOA switch to\namplify the non ABSORBING\nwavelength"
                                n311 = Build Array(TRUE ("Boolean")) -> (w415:bool[])
                                n312 = call-poly <vilib>:"DAQmx Write.vi"("task/channels in"=refnum<k21> "BristolWM", "data"=w415) -> ()  [unwired: 11 in, 3 out]
                                n313 = Wait (ms)(milliseconds to wait=u32 3200) -> ()  [unwired: 1 out]
                                }
                              }
                            }
                            frame #1 {
                              # "Reading the wavelength from the wavemeter"
                              n314 = flat-sequence {
                                tunnel: [w420] -> w419
                                tunnel: w419 -> [w423]
                                tunnel: [w422] -> w418
                                tunnel: w418 -> [w426]
                                frame #0 {
                                n315 = local read "Bristol In"() -> (w421:i32)
                                n316 = dll-call lib="C:/Users/H2ODial/Desktop/Shared Telescope WV DIAL Code/bristol/CLDevIface.dll" fn="CLOpenUSBSerialDevice"("commPort"=w421) -> ("return type"=w420:i32)  [unwired: 4 in, 2 out]
                                }
                                frame #1 {
                                n317 = dll-call lib="C:/Users/H2ODial/Desktop/Shared Telescope WV DIAL Code/bristol/CLDevIface.dll" fn="CLGetLambdaReading"("devHandle"=w423) -> ("return type"=→"Lambda Off Read (nm)":dbl, "devHandle"=w422:i32)  [unwired: 3 in, 2 out]
                                }
                                frame #2 {
                                n318 = dll-call lib="C:/Users/H2ODial/Desktop/Shared Telescope WV DIAL Code/bristol/CLDevIface.dll" fn="CLCloseDevice"("commPort"=w426) -> ("return type"=w425:i32)  [unwired: 4 in, 2 out]
                                n319 = local write "Bristol Out"(w425) -> ()
                                }
                              }
                            }
                            frame #2 {
                              # "Calculating the difference between the actual and desired online wavelength"
                              n320 = local read "Offline_Tol"() -> (w429:dbl)
                              n321 = local read "Lambda Off Read (nm)"() -> (w435:dbl)
                              n322 = Multiply(x=-1.0, y=w429) -> (x*y=w428:dbl)
                              n323 = Subtract(x=w435, y="Lambda Off Set (nm)") -> (x-y=w431:dbl)
                              "WL Difference off" <- w431
                              n324 = Greater?(x=w431, y=w428) -> (0:w432:bool)
                              n325 = Less?(x=w431, y=w429) -> (x < y?=w433:bool)
                              n326 = And(x=w432, y=w433) -> (x .and. y?=w427:bool)
                              "Wavelength Lock Offline" <- w427
                              n327 = case shown="True" w427 {
                                frame False {
                                }
                                frame True {
                                # "Set the TSOA switch to\namplify the ABSORBING\nwavelength"
                                n328 = Build Array(FALSE ("Boolean")) -> (w437:bool[])
                                n329 = call-poly <vilib>:"DAQmx Write.vi"("task/channels in"=refnum<k21> "BristolWM", "data"=w437) -> ()  [unwired: 11 in, 3 out]
                                n330 = Wait (ms)(milliseconds to wait=u32 3200) -> ()  [unwired: 1 out]
                                }
                              }
                            }
                            frame #3 {
                              # "If the wavelength difference is greater that 0.0002 nm, decrement the \nDBR current by 0.01 mA"
                              n331 = local read "WL Difference off"() -> (w442:dbl)
                              n332 = Greater Or Equal?(x=w442, y="Offline_Tol") -> (x >= y?=w441:bool)
                              n333 = case shown="True" w441 {
                                frame False {
                                # "Wavelength difference is not greater than 0.0002 nm, do nothing"
                                }
                                frame True {
                                # "Generating a command string\nto decrement the current"
                                n334 = local read "Settings"() -> (w449:T7)
                                n335 = Unbundle By Name(w449) -> ("OffLineTEC"=w446:dbl)
                                n336 = Subtract(x=w446, y="y") -> (x-y=w445:dbl)
                                n337 = local read "Device In"() -> (w443:refnum<visa-resource-name>)
                                n338 = Bundle By Name(cluster=w449, "OffLineTEC"=w445, "Module"=T12."Off Line TEC") -> (w450:T7)
                                n339 = call "TL_Driver.vi"("Device In"=w443, "Commands"=T9."SET", "Settings"=w450) -> ("Readings"=w451:T6)  [unwired: 9 in, 3 out]
                                n340 = local write "Settings"(w450) -> ()
                                n341 = local write "Readings"(w451) -> ()
                                }
                              }
                            }
                            frame #4 {
                              # "If WL difference is < 0.0002 nm, increment the DBR current"
                              n342 = local read "WL Difference off"() -> (w454:dbl)
                              n343 = Less Or Equal?(x=w454, y=-0.0001) -> (x <= y?=w452:bool)
                              n344 = case shown="True" w452 {
                                frame False {
                                # "WL difference is no <= to -0.0002 nm, do nothing"
                                }
                                frame True {
                                # "Generating a command string\nto decrement the current"
                                # "WL difference is less than 0.0002 nm,\nincrement the DBR current by 0.01 mA"
                                n345 = local read "Settings"() -> (w462:T7)
                                n346 = Unbundle By Name(w462) -> ("OffLineTEC"=w459:dbl)
                                n347 = local read "y"() -> (w455:dbl)
                                n348 = Add(x=w459, y=w455) -> (x+y=w458:dbl)
                                n349 = local read "Device In"() -> (w456:refnum<visa-resource-name>)
                                n350 = Bundle By Name(cluster=w462, "OffLineTEC"=w458, "Module"=T12."Off Line TEC") -> (w463:T7)
                                n351 = call "TL_Driver.vi"("Device In"=w456, "Commands"=T9."SET", "Settings"=w463) -> ("Readings"=w461:T6)  [unwired: 9 in, 3 out]
                                n352 = local write "Settings"(w463) -> ()
                                n353 = local write "Readings"(w461) -> ()
                                }
                              }
                            }
                          }
                          n354 = Or(x=w408, y="Cancel Offline") -> (x .or. y?=w409:bool)
                        }
                      }
                    }
                  }
                  frame #1 {
                    # "Reading the power meter"
                    # "Updating the pulse energy plot"
                    # "Converting to pulse energy"
                    # "Reading the offline output power, converting to pulse energy,  and updating the Pulse energy plot"
                    n355 = local read "SampleSize"() -> (w466:i32)
                    n356 = local read "Newport Device Key"() -> (w467:string)
                    n357 = local read "Online Pulse Energy"() -> (w473:dbl)
                    n358 = local read "Offline Pulse Energy"() -> (w472:dbl)
                    n359 = local read "NewportRef"() -> (w464:refnum<k24>)
                    n360 = Number To Decimal String(number=w466) -> (decimal integer string=w468:string)  [unwired: 1 in]
                    n361 = invoke class="PowerMeterCommands" method="PerformDAQ"(reference=w464, "deviceKey"=w467, "interval"="1", "sampleSize"=w468) -> ("PerformDAQ"=w469:dbl[])  [unwired: 2 in, 5 out]
                    n362 = Bundle("Online Pulse Energy"=w473, "Offline Pulse Energy"=w472) -> (w471:T15)  [unwired: 1 in]
                    n363 = local write "Pulse Energy (Micro Joule)"(w471) -> ()
                    n364 = call-poly <vilib>:"Mean.vi"("X"=w469) -> ("mean"=w465:dbl)  [unwired: 1 out]
                    n365 = Multiply(x=w465, y=1000.0) -> (x*y=w478:dbl)
                    n366 = Divide(x=w478, y=0.05) -> (x/y=w476:dbl)
                    n367 = Divide(x=w476, y=7.0) -> (x/y=→"Offline Pulse Energy":dbl)
                  }
                  frame #2 {
                    # "Wait 'Scalar Wait Time' for buffers to clear of online contiminated offline data"
                    n368 = disable-structure shown="Disabled" {
                      frame Disabled {
                        # "Wait 'Scalar Wait Time'"
                        n369 = local read "Scalar Wait Time"() -> (w480:u32)
                        n370 = Wait (ms)(milliseconds to wait=w480) -> ()  [unwired: 1 out]
                      }
                      frame Enabled {
                      }
                    }
                  }
                  frame #3 {
                    w514 = 1 ("dimension size")
                    w518 = 1
                    # "Read in latest scalar card data from \n'Scalar Data' global variable that \nscaler.vi is writing to, then wait 1 sec\nfor next batch of data"
                    # "Plotting the normalized relative \nbackscatter"
                    # "Calculating the normalized relative backscatter"
                    # "Calculating/Plotting smoothed data,\ncross sections etc."
                    # "Pick off data with\nout header"
                    # "Calculate mean bin by bin mean"
                    # "Reading in 'Integration Period (Seconds)' of data"
                    # "Read the offline data from the scalar card, perform smoothing, calculate normalized relative backscatter, and plot"
                    # "File path in MATLAB script is of old dial is:\nF:\\Micropulse DIAL\\Micropulse DIAL Matlab\\\nFinal Overlap Function.mat')];"
                    # "Collects Data From Card,\nSends It To The Chart,\nAnd Saves A Copy As A\nFile If Option Selected On\nFront Panel"
                    n371 = for {
                      N: "Data Reads (number of loops)" -> [_]
                      tunnel: [w550] -> w482 mode=indexing
                      tunnel: [w549] -> w481 mode=indexing
                      n372 = global read "AMCS_Data.vi" "AMCS_Data"() -> (w551:u16[][])
                      n373 = disable-structure shown="Disabled" {
                        frame Disabled {
                          n374 = global read "Scalar_Data_4.vi" "Scalar Data 4"() -> ()  [unwired: 1 out]
                          n375 = global read "Scalar_Data_2.vi" "Scalar Data 2"() -> ()  [unwired: 1 out]
                        }
                        frame Enabled {
                        }
                      }
                      n376 = Index Array(array=w551, index (row) #1=1 ("index (row)"), index (row) #2=3 ("index (row)")) -> (element #1=w550:u16[], element #2=w549:u16[])  [unwired: 2 in]
                    }
                    n377 = local read "Total DIAL Integration Time (Minutes)"() -> (w539:i32)
                    n378 = Divide(x=w539, y="Data Reads (number of loops)") -> (x/y=w537:dbl)
                    n379 = local read "Total Aerosol Integration Time (Minutes)"() -> (w541:dbl)
                    n380 = local read "background length"() -> (w486:i32)
                    n381 = Multiply(x=w537, y=60.0) -> (x*y=w524:dbl)
                    n382 = local read "background start"() -> (w487:u32)
                    n383 = Transpose 2D Array(2D array=w482) -> (transposed array=w547:u16[][])
                    n384 = Transpose 2D Array(2D array=w481) -> (transposed array=w530:u16[][])
                    n385 = Divide(x=w541, y="Data Reads (number of loops)") -> (x/y=w542:dbl)
                    n386 = for {
                      tunnel: w547 -> [w557] mode=indexing
                      tunnel: [w556] -> w548 mode=indexing
                      tunnel: w530 -> [w555] mode=indexing
                      tunnel: [w554] -> _ mode=indexing
                      tunnel: [w554] -> w527 mode=indexing
                      n387 = call-poly <vilib>:"Mean.vi"("X"=w557) -> ("mean"=w556:dbl)  [unwired: 1 out]
                      n388 = call-poly <vilib>:"Mean.vi"("X"=w555) -> ("mean"=w554:dbl)  [unwired: 1 out]
                    }
                    n389 = local read "bins"() -> (w515:u32)
                    n390 = Multiply(x=w542, y=60.0) -> (x*y=w505:dbl)
                    n391 = Array Subset(array=w527, index=w514, length=w515) -> (w528:dbl[])
                    "Off-Line Bin Readings 2" <- w528
                    n392 = Array Subset(array=w548, index=w514, length=w515) -> (w526:dbl[])
                    "Off-Line  Bin Readings" <- w526
                    n393 = Array Subset(array=w528, index=w487, length=w486) -> (w529:dbl[])
                    n394 = Array Subset(array=w526, index=w487, length=w486) -> (w546:dbl[])
                    n395 = local read "Smoothed Bins"() -> (w483:dbl)
                    n396 = call-poly <vilib>:"Mean.vi"("X"=w529) -> ("mean"=w493:dbl)  [unwired: 1 out]
                    n397 = call-poly <vilib>:"Mean.vi"("X"=w546) -> ("mean"=w494:dbl)  [unwired: 1 out]
                    n398 = local read "Index"() -> (w504:i32)
                    n399 = Subtract(x=w528, y=w493) -> (x-y=w506:dbl[])
                    n400 = Subtract(x=w526, y=w494) -> (x-y=w522:dbl[])
                    n401 = call "Ring Buffer Offline Far.vi"("Index"=w504, "Profiles to Average"=w524, "Input Array"=w522) -> ("AvgArray"=w544:dbl[], "RingBufferOut"=→"RingBuffer offline far":dbl[][])  [unwired: 7 in]
                    n402 = call "Ring Buffer Aerosol Far.vi"("Index"=w504, "Profiles to Average"=w505, "Input Array"=w522) -> ("AvgArray"=w540:dbl[], "RingBufferOut"=→"RingBuffer aerosol far":dbl[][])  [unwired: 7 in]
                    n403 = call "Ring Buffer Offline Near.vi"("Index"=w504, "Profiles to Average"=w524, "Input Array"=w506) -> ("AvgArray"=w525:dbl[], "RingBufferOut"=→"RingBuffer offline near":dbl[][])  [unwired: 7 in]
                    n404 = call "Ring Buffer Aerosol Near.vi"("Index"=w504, "Profiles to Average"=w505, "Input Array"=w506) -> ("AvgArray"=w502:dbl[], "RingBufferOut"=→"RingBuffer aerosol near":dbl[][])  [unwired: 7 in]
                    n405 = Reshape Array(w522, w514, w515) -> (→"raw counts":dbl[][])
                    n406 = Reshape Array(w506, w514, w515) -> (→"raw counts near":dbl[][])
                    n407 = call "Smooth Arrray.vi"("smooth size"=w483, "Raw Array"=w544) -> ("Smoothed Array"=→"Off-Line Smoothed":dbl[])  [unwired: 9 in]
                    n408 = call "Smooth Arrray.vi"("smooth size"=w483, "Raw Array"=w540) -> ("Smoothed Array"=w513:dbl[])  [unwired: 9 in]
                    "Aerosol Smoothed" <- w513
                    n409 = call "Smooth Arrray.vi"("smooth size"=w483, "Raw Array"=w525) -> ("Smoothed Array"=→"Off-Line Smoothed 2":dbl[])  [unwired: 9 in]
                    n410 = call "Smooth Arrray.vi"("smooth size"=w483, "Raw Array"=w502) -> ("Smoothed Array"=w485:dbl[])  [unwired: 9 in]
                    "Aerosol Smoothed 2" <- w485
                    n411 = local read "Number of Accumulates"() -> (w489:u32)
                    n412 = local read "Temperature (C)"() -> (w536:dbl)
                    n413 = local read "Pressure (mb)"() -> (w535:dbl)
                    n414 = script code="%accum_num=10000;     % scaler card setting number of accumulations\nt_bin = 500e-9                 % scaler card setting time per bin\n%t_d = 37.3e-9;                % APD dead time from spec sheet\n\n% conversion from accumulated counts to count rate  (c/s)\nc_convert = 1./t_bin./accum_num;\nCR_far = p_raw_far.*c_convert;\nCR_near = p_raw_near.*c_convert;\nCR_total_far = (p_raw_far+b_far).*c_convert;\nCR_total_near = (p_raw_near+b_near).*c_convert;\nb_CR_far =b_far.*c_convert;\nb_CR_near =b_near.*c_convert;\n\n% create a range array\nsize_p =  size(p_raw_far,2);\nr = (75:75:size_p*75)./1e3; \n    \n%APD correction factor\n D_far = 1./(1-(t_d*CR_total_far));\n D_near = 1./(1-(t_d*CR_total_near));\n\n %Calculating normalize relative backscatter profile\n nrb_far = CR_far.*D_far.*r.^2.*1e-6;\n nrb_near = CR_near.*D_near.*r.^2.*1e-6;"("E"=6.0 ("Real"), "temp"=w536, "press"=w535, "p_raw_far"=w513, "b_far"=w494, "b_near"=w493, "p_raw_near"=w485, "accum_num"=w489, "t_d"="dead time") -> ("nrb_far"=w508:cdb[], "D_far"=w499:dbl[], "nrb_near"=w507:cdb[], "D_near"=w498:dbl[], "b_CR_far"=w491:dbl, "b_CR_near"=w490:dbl)  [unwired: 1 in, 1 out]
                    n415 = local read "bins"() -> (w517:u32)
                    n416 = local read "Altitude Array (km)"() -> (w510:dbl[])
                    n417 = Bundle(w491, w490) -> (→"?":cluster{dbl, dbl})  [unwired: 1 in]
                    n418 = Build Array(w508, w507) -> (w512:cdb[][])
                    n419 = Build Array(w499, w498) -> (w497:dbl[][])
                    n420 = Reshape Array(w507, w518, w517) -> (→"NRB 2":cdb[][])
                    n421 = Reshape Array(w508, w518, w517) -> (→"NRB":cdb[][])
                    n422 = Build Array(w510, w510) -> (w509:dbl[][])
                    n423 = call "Convert to Dynamic Data7"("2D Array"=w497) -> ("Dynamic Data Type"=w496:dynamicdata)  [unwired: 3 in]
                    n424 = call "Convert to Dynamic Data3"("2D Array"=w512) -> ("Dynamic Data Type"=w511:dynamicdata)  [unwired: 3 in]
                    n425 = call "Convert to Dynamic Data4"("2D Array"=w509) -> ("Dynamic Data Type"=w500:dynamicdata)  [unwired: 3 in]
                    n426 = call "Build XY Graph2"("Y Input"=w500, "X Input"=w511) -> ("XY Graph"=→"NRB plot":cluster{"Y":dbl[], "Y":dbl[]}[])  [unwired: 3 in, 6 out]
                    n427 = call "Build XY Graph4"("Y Input"=w500, "X Input"=w496) -> ("XY Graph"=→"Correction":cluster{"Y":dbl[], "Y":dbl[]}[])  [unwired: 3 in, 6 out]
                  }
                  frame #4 {
                    # "REPLACE WITH NEW AGILTRON TASK!"
                    # "Toggle Agiltron switch to online DBR"
                    n428 = disable-structure shown="Disabled" {
                      frame Disabled {
                        # "ABSORBING"
                        n429 = flat-sequence {
                          frame #0 {
                            # "Third one"
                            # "Command the switch to switch to position 1\ncorresponding to the online DBR"
                            # "Hex string command \ncorrespond to online"
                            n430 = local read "Switch Comm Port"() -> (w561:refnum<visa-resource-name>)
                            n431 = VISA Write(VISA resource name=w561, write buffer="\u0001\u0012\u0000\u0002") -> ()  [unwired: 1 in, 3 out]
                          }
                        }
                        n432 = Build Array(FALSE ("Boolean")) -> (w560:bool[])
                        n433 = call-poly <vilib>:"DAQmx Write.vi"("task/channels in"=refnum<k21> "AgiltronSwitch", "data"=w560) -> ()  [unwired: 11 in, 3 out]
                      }
                      frame Enabled {
                      }
                    }
                  }
                  frame #5 {
                    # "If 'Save Data?' is true, save all relavant offline info"
                    n434 = local read "Save Data?"() -> (w563:bool)
                    n435 = case shown="True" w563 {
                      frame False {
                        # "'Save Data?' is false, do nothing"
                      }
                      frame True {
                        # "Write only one data file at this time"
                        # "Retrive Julian Date"
                        # "'Save Data?' is true, save offline data to the Data Disk"
                        n436 = local read "Lambda Off DBR Current"() -> (w585:dbl)
                        n437 = local read "Off-Line Bin Readings 2"() -> (w582:dbl[])
                        n438 = local read "Lambda Off Read (nm)"() -> (w584:dbl)
                        n439 = local read "Off-Line  Bin Readings"() -> (w590:dbl[])
                        n440 = local read "Relative Humdity (%)"() -> (w589:dbl)
                        n441 = local read "Offline Pulse Energy"() -> (w586:dbl)
                        n442 = local read "Temperature (C)"() -> (w587:dbl)
                        n443 = local read "Pressure (mb)"() -> (w588:dbl)
                        n444 = call "Julian_Date_2.vi"() -> ("Julian Date"=w583:dbl)  [unwired: 11 in]
                        n445 = Build Array (concatenate)(w583, w584, w585, w586, w587, w588, w589, w590) -> (w568:dbl[])
                        n446 = Build Array (concatenate)(w583, w584, w585, w586, w587, w588, w589, w582) -> (w565:dbl[])
                        n447 = local read "FF_Off_Ref"() -> (w570:refnum<file>)
                        n448 = local read "NF_Off_Ref"() -> (w567:refnum<file>)
                        n449 = local read "FF_Off_Ptr"() -> (w569:i64)
                        n450 = local read "NF_Off_Ptr"() -> (w566:i64)
                        n451 = Set File Position(offset (in bytes) (0)=w569, refnum=w570) -> (refnum out=w581:refnum<file>, error out=w579:errorcluster)  [unwired: 2 in]
                        n452 = Set File Position(offset (in bytes) (0)=w566, refnum=w567) -> (refnum out=w577:refnum<file>, error out=w575:errorcluster)  [unwired: 2 in]
                        n453 = Write to Binary File(file (use dialog)=w581, data=w568, error in=w579, 5:FALSE ("prepend array or string size? (T)")) -> (refnum out=w580:refnum<file>, error out=w578:errorcluster)  [unwired: 2 in, 1 out]
                        n454 = Write to Binary File(file (use dialog)=w577, data=w565, error in=w575, 5:FALSE ("prepend array or string size? (T)")) -> (refnum out=w576:refnum<file>, error out=w574:errorcluster)  [unwired: 2 in, 1 out]
                        n455 = Get File Position(4:w578, 7:w580) -> (2:w571:i64)  [unwired: 2 out]
                        n456 = Get File Position(4:w574, 7:w576) -> (2:w564:i64)  [unwired: 2 out]
                        n457 = local write "FF_Off_Ptr"(w571) -> ()
                        n458 = local write "NF_Off_Ptr"(w564) -> ()
                      }
                    }
                  }
                }
              }
              frame #4 {
                n459 = First Call?() -> (First Call?: T/F=w593:bool)
                n460 = Or(x="calculate absorption cross sections", y=w593) -> (x .or. y?=w591:bool)
                n461 = case shown="True" w591 {
                  frame False {
                  }
                  frame True {
                    # "calculate absorption cross sections from HITRAN data base"
                    n462 = local read "Off-Line Smoothed"() -> (w594:dbl[])
                    n463 = local read "Lambda On Read (nm)"() -> (w597:dbl)
                    n464 = local read "Lambda Off Set (nm)"() -> (w600:dbl)
                    n465 = local read "Temperature (C)"() -> (w598:dbl)
                    n466 = local read "Pressure (mb)"() -> (w599:dbl)
                    n467 = script code="%Importing HITRAN data\n%hitran = dlmread('C:\\Users\\H2ODial\\Desktop\\Shared Telescope WV DIAL Code\\Libraries and VIs\\824nm_841nm_H2O.csv', ',',[0 1 352 7]);\nhitran = dlmread('C:\\Users\\H2ODial\\Desktop\\Shared Telescope WV DIAL Code\\Libraries and VIs\\824nm_841nm_H2O_Spectral_Calc.csv', ',',[1 1 1209 7]);\n\n%Range vector in meters\nrange = ([75:75:size(Online,2)*75]);\n\nif lambda< 828\nlambda=828.195;\nelse\nlambda=lambda;\nend;\n\n%%\n\n%Voigt profile calculation\nWNmin = 12070.0;\nWNmax = 12076.0;\n\n%Find lines from WNmin to WNmax to calculate voigt profile\nline_indices = find(hitran(1:size(hitran,1),1)>WNmin & hitran(1:size(hitran,1),1)<WNmax);\n\nline = (hitran(line_indices, 1:size(hitran,2)));\n\n%Calculate temperature and pressure profile\nT0 = 273+15.6;\nT0 = 273+T0_C;\n\nT = T0-0.005545.*range; \n\nP0  = 1.0;\nP0  = P0_mb/1000*0.986; %pressure in mb converted to atm\n\nP = P0.*(T0./T).^-5.21986;\n\n%linewidth temperature dependence factor\nalpha = line(:,7);        \n\n%initial Lorentz linewidth from HiTRAN [cm^-1]\ngammal0 = line(:,4);     \n\n%ground state transition energy [cm^-1]\nE = line(:,6);           \n\n%initial linestrength from HiTRAN [cm^-1/(mol*cm^-2)]\nS0 = line(:,2);      \n\n%absorption line center wavenumber from HiTRAN [cm^-1]\nnu0_0 = line(:,1);    \n\nnu_on = (1/(lambda)*1e7);\n\nnu_off = (1/(lambda_off)*1e7);\n\n\nfor i = 1:size(Online,2);\n\n    %Pressure shift\n    nu0 = nu0_0-.0428.*P(i);\n    \n    %Calculate Lorentz lineweidth at temperature T [cm^-1]\n    gammal = gammal0.*(P(i)./P0).*((T0./T(i)).^alpha);\n    \n    %Calculate Doppler linewidth at temperature T [cm^-1]\n    gammad = (nu0).*((2.0.*1.38E-23.*T(i).*log(2.0))./(0.018.*3.0E8.*3.0E8./6.022E23)).^(0.5);\n    \n    y = (gammal./gammad).*((log(2.0)).^(0.5));\n    \n    x_on = ((nu_on-nu0)./gammad).*(log(2.0)).^(0.5);\n    \n    x_off = ((nu_off-nu0)./gammad).*(log(2.0)).^(0.5);\n    \n    %setting up Voigt convolution\n    stepsize = 1;\n    \n    t = [-200:1:199].*stepsize;\n    \n    t = repmat(t',1,length(x_on))';\n    \n    x_on = repmat(x_on,1,length(t));\n    \n    x_off = repmat(x_off,1,length(t));\n    \n    y = repmat(y,1,length(t));\n    \n    f_on = (exp(-t.^2.0))./(y.^2.0+(x_on-t).^2.0);\n    \n    f_off = (exp(-t.^2.0))./(y.^2.0+(x_off-t).^2.0);\n    \n    %Set the integration sum to zero to start\n    integral_on = 0.0;\n    \n    integral_off = 0.0;\n    \n    %Voigt integration\n    z_on = trapz(t(1,:),f_on,2);\n    \n    z_off =  trapz(t(1,:),f_off,2);\n    \n    integral_on = z_on;\n    \n    integral_off = z_off;\n    \n    %Calculate linestrength at temperature T\n    S = S0.*((T0./T(i)).^(1.5)).*exp(1.439.*E.*((1./T0)-(1./T(i))));\n    \n    %Calculate Doppler line-center cross section [cm^2]\n    K = (S./gammad).*(((log(2.0))./pi).^(0.5));\n    \n    %Calculate the Voigt profile\n    V_on = (y(1)/pi).*integral_on;\n    \n    V_off = (y(1)./pi).*integral_off;\n    \n    %Calculate the Voigt profile absorption cross section [cm^2]\n    sigmav_on = K.*V_on;\n    \n    sigmav_off = K.*V_off;\n    \n    %Sum contributions from all of the surrounding lines\n    sigma_on_total(i) = sum(sigmav_on);\n    \n    sigma_off_total(i) = sum(sigmav_off);\n    \nend;"("lambda"=w597, "lambda_off"=w600, "P0_mb"=w599, "T0_C"=w598, "Online"=w594) -> ("sigma_on_total"=→"sigma_on_total":dbl[], "sigma_off_total"=→"sigma_off_total":dbl[])  [unwired: 1 in, 1 out]
                  }
                }
              }
              frame #5 {
                w611 = 1
                # "normalization factor\nfrom 300 to 450m"
                # "OPTICAL DEPTH PLOT"
                # "new rainbow color bar display"
                # "Data Processing Far Channel"
                # "new rainbow color bar display"
                # "Calculating the range resolved water vapor number density and plotting"
                n468 = local read "sigma_off_total"() -> (w634:dbl[])
                n469 = local read "sigma_on_total"() -> (w631:dbl[])
                n470 = local read "On-Line  Smoothed"() -> (w609:dbl[])
                n471 = local read "Off-Line Smoothed"() -> (w608:dbl[])
                n472 = local read "Off-Line Smoothed 2"() -> (w632:dbl[])
                n473 = local read "On-Line Smoothed 2"() -> (w633:dbl[])
                n474 = script code="%Time averaging in seconds.  600 Seconds =10 minutes\ntemporal_average = 600;\n\n%Spatial averaging in bins.  2 bins = 150 meters\nspatial_average = 2;\n\n%Creating r and r+deltar vectors..this can also be acsomplished using the\n%diff command\np_oni = Online(:,1:size(Online,2)-1);\n\np_onii = Online(:,2:size(Online,2));\n\np_offi = Offline(:,1:size(Offline,2)-1);\n\np_offii = Offline(:,2:size(Offline,2));\n\nInside = (p_oni.*p_offii)./(p_onii.*p_offi);\n\ndel_cross = 1./(2.*(sigma_on_total(1:size(Online,2)-1)-sigma_off_total(1:size(Offline,2)-1)).*75*100);\n\ndel_cross(isinf(del_cross)) = 0;\n\n%Calculating Number density\nN = del_cross.*log(Inside);\n\n%Spatial smoothing of the profiles\nfilter1 = ones(1,2)./2;\n\nN_1 = N;\n\nN_1_avg = filter2(filter1,N_1);\n\nfilter1 = ones(1,10)./10;\n\nN_2 = N;\n\nN_2_avg = filter2(filter1,N_2);\n\nN_new = zeros(size(N,1),size(N,2));\n \n%Using different averaging windows for different altitudes \nN_avg=[N_1_avg(:,1:40)';N_2_avg(:,41:size(N,2))']';\n\n\nw = N_avg.*1e6.*18.015./6.022e23"("Online"=w633, "Offline"=w632, "sigma_on_total"=w631, "sigma_off_total"=w634) -> ("N_avg"=w635:cdb[], "w"=w644:cdb[])  [unwired: 1 in, 1 out]
                n475 = script code="%Time averaging in seconds.  600 Seconds = 10 minutes\ntemporal_average = 600;\n\n%Spatial averaging in bins.  2 bins = 150 meters\nspatial_average = 2;\n\n%Creating r and r+deltar vectors..this can also be acsomplished using the\n%diff command\np_oni = Online(:,1:size(Online,2)-1);\n\np_onii = Online(:,2:size(Online,2));\n\np_offi = Offline(:,1:size(Offline,2)-1);\n\np_offii = Offline(:,2:size(Offline,2));\n\nInside = (p_oni.*p_offii)./(p_onii.*p_offi);\n\ndel_cross = 1./(2.*(sigma_on_total(1:size(Online,2)-1)-sigma_off_total(1:size(Offline,2)-1)).*75*100);\n\ndel_cross(isinf(del_cross)) = 0;\n\n%Calculating Number density\nN = del_cross.*log(Inside);\n\n%Spatial smoothing of the profiles\nfilter1 = ones(1,2)./2;\n\nN_1 = N;\n\nN_1_avg = filter2(filter1,N_1);\n\nfilter1 = ones(1,10)./10;\n\nN_2 = N;\n\nN_2_avg = filter2(filter1,N_2);\n\nN_new = zeros(size(N,1),size(N,2));\n \n%Using different averaging windows for different altitudes \nN_avg=[N_1_avg(:,1:40)';N_2_avg(:,41:size(N,2))']';\n\n \nw = N_avg.*1e6.*18.015./6.022e23"("Online"=w609, "Offline"=w608, "sigma_on_total"=w631, "sigma_off_total"=w634) -> ("N_avg"=w640:cdb[], "w"=w641:cdb[])  [unwired: 1 in, 1 out]
                n476 = local read "Time Resolution Per Bin(ns)"() -> (w610:u32)
                n477 = local read "bins"() -> (w636:u32)
                n478 = local read "Altitude Array (km)"() -> (w606:dbl[])
                n479 = Build Array(w641, w644) -> (w647:cdb[][])
                n480 = To Double Precision Float(number=w610) -> (double precision float=w629:dbl)
                n481 = Reshape Array(w640, w611, w636) -> (w651:cdb[][])
                n482 = Reshape Array(w635, w611, w636) -> (w638:cdb[][])
                n483 = Multiply(x=0.15, y=w629) -> (x*y=w627:dbl)
                n484 = Build Array(w640, w635) -> (w645:cdb[][])
                n485 = Divide(x=300.0, y=w627) -> (x/y=w624:dbl)
                n486 = Divide(x=450.0, y=w627) -> (x/y=w623:dbl)
                n487 = Build Array(w606, w606) -> (w630:dbl[][])
                n488 = call "Convert to Dynamic Data5"("2D Array"=w647) -> ("Dynamic Data Type"=w646:dynamicdata)  [unwired: 3 in]
                n489 = call "Convert to Dynamic Data2"("2D Array"=w645) -> ("Dynamic Data Type"=w642:dynamicdata)  [unwired: 3 in]
                n490 = Divide(x=w651, y=1e+17) -> (x/y=→"Water Vapor Number Density":cdb[][])
                n491 = Divide(x=w638, y=1e+17) -> (x/y=→"Water Vapor Number Density 2":cdb[][])
                n492 = call "Convert to Dynamic Data6"("Array"=w606) -> ("Dynamic Data Type"=w607:dynamicdata)  [unwired: 3 in]
                n493 = To Long Integer(number=w624) -> (32bit integer=w622:i32)
                n494 = To Long Integer(number=w623) -> (32bit integer=w621:i32)
                n495 = call "Convert to Dynamic Data"("2D Array"=w630) -> ("Dynamic Data Type"=w643:dynamicdata)  [unwired: 3 in]
                n496 = call "Convert to Dynamic Data8"("2D Array"=w630) -> ("Dynamic Data Type"=w648:dynamicdata)  [unwired: 3 in]
                n497 = Decrement(x=w622) -> (x-1=w619:i32)
                n498 = Decrement(x=w621) -> (x-1=w620:i32)
                n499 = call "Build XY Graph"("Y Input"=w643, "X Input"=w642) -> ("XY Graph"=→"Water Vapor Number Density  2":cluster{"Y":dbl[], "Y":dbl[]}[])  [unwired: 3 in, 6 out]
                n500 = call "Build XY Graph3"("Y Input"=w648, "X Input"=w646) -> ("XY Graph"=→"Absolute Humidity":cluster{"Y":dbl[], "Y":dbl[]}[])  [unwired: 3 in, 6 out]
                n501 = Array Subset(array=w609, index=w619, length=w620) -> (w618:dbl[])
                n502 = Array Subset(array=w608, index=w619, length=w620) -> (w617:dbl[])
                n503 = call-poly <vilib>:"Mean.vi"("X"=w618) -> ("mean"=w616:dbl)  [unwired: 1 out]
                n504 = call-poly <vilib>:"Mean.vi"("X"=w617) -> ("mean"=w615:dbl)  [unwired: 1 out]
                n505 = Divide(x=w616, y=w615) -> (x/y=w614:dbl)
                n506 = Multiply(x=w608, y=w614) -> (x*y=w613:dbl[])
                n507 = Divide(x=w609, y=w613) -> (x/y=w612:dbl[])
                n508 = Natural Logarithm(1:w612) -> (0:w603:dbl[])
                n509 = Multiply(x=-1.0, y=w603) -> (x*y=w602:dbl[])
                n510 = call "Convert to Dynamic Data9"("Array"=w602) -> ("Dynamic Data Type"=w605:dynamicdata)  [unwired: 3 in]
                n511 = call "Build OD Plot"("Y Input"=w607, "X Input"=w605) -> ("XY Graph"=→"Optical Depth":cluster{"Y":dbl[], "Y":dbl[]}[])  [unwired: 3 in, 6 out]
              }
            }
          }
        }
        "L_Count" <- w128
      }
    }
  }
  n512 = case shown="True" w3 {
    frame False {
    }
    frame True {
      # "close data files"
      n513 = local read "NF_Off_Ref"() -> (w655:refnum<file>)
      n514 = local read "NF_On_Ref"() -> (w656:refnum<file>)
      n515 = local read "FF_Off_Ref"() -> (w657:refnum<file>)
      n516 = local read "FF_On_Ref"() -> (w658:refnum<file>)
      n517 = local read "WS_On/Off"() -> (w654:bool)
      n518 = case shown="True" w654 {
        frame False {
        }
        frame True {
          n519 = local read "WS visa"() -> (w659:refnum<visa-resource-name>)
          n520 = call "T_RH_P.vi"("VISA in"=w659, "WS_Commands"=enum16{"OpenWS", "ReadTRHP", "CloseWS"}."CloseWS") -> ()  [unwired: 11 in, 3 out]
        }
      }
      n521 = Close File(refnum=w658) -> ()  [unwired: 1 in, 2 out]
      n522 = Close File(refnum=w657) -> ()  [unwired: 1 in, 2 out]
      n523 = Close File(refnum=w656) -> ()  [unwired: 1 in, 2 out]
      n524 = Close File(refnum=w655) -> ()  [unwired: 1 in, 2 out]
    }
  }
  "FileHour" <- -1 ("FileHour")
  "DataOpen" <- FALSE
